vi "COD主界面（列队使用）.vi"() -> (8 "多列列表框":i32(listbox))   [LabVIEW 2016, in "斯坦道CODMn.lvlib"]
uses:
  <vilib>/Utility/miscctls.llb/LVPointTypeDef.ctl
  <vilib>/Analysis/6fits.llb/Curve Fitting Criteria.ctl
  <vilib>/Utility/config.llb/Read Key (I32).vi
  <vilib>/Utility/config.llb/Read Key (Double).vi
  <vilib>/Utility/config.llb/Read Key (Boolean).vi
  <vilib>/Utility/config.llb/Write Key (Double).vi
  <vilib>/Utility/config.llb/Write Key (Boolean).vi
  <vilib>/Utility/config.llb/Write Key (I32).vi
  <vilib>/Waveform/WDTFileIO.llb/Read Waveform from File.vi
  <vilib>/ptbypt/NI_PtbyPt.lvlib
  <vilib>/Utility/config.llb/NI_LVConfig.lvlib
  <vilib>/Analysis/NI_AALPro.lvlib
panel:
  out "CODMn工作状态":T1(ring)
  out "ORP-K":string
  out "ORP-B":string
  out "ORP-A":string
  out "x = y?":bool
  out "稀释倍数解释":string
  in  "CODMn跨度量程选择":enum32{"H", "L", "AUTO"}(ring)=enum."AUTO"
  in  "跨度液浓度":dbl
  in  "水样":dbl
  in  "蒸馏水":dbl
  in  "标液":dbl
  in  "质控样":dbl
  in  "加标回收":dbl
  in  "草酸钠":dbl
  in  "高锰酸钾":dbl
  in  "硫酸":dbl
  out "量程解释说明":string
  in  "高切低阈值:":dbl
  in  "低切高阈值:":dbl
  in  "自动切换量程:":enum16{"关闭", "自动切换测一次", "自动切换测两次"}(ring)
  in  "修正系数":dbl
  in  "标准液浓度":dbl
  in  "温度":dbl
  in  "恒温时间":dbl
  in  "基本量程":enum16{"L", "H"}(ring)
  in  "CODMn零点核查选择":enum16{"零点核查走纯水管", "零点核查走质控管"}(ring)
  in  "锁定按钮":bool
  in  "低量程稀释倍数:":i8=1
  out "切换量程连续测两次":bool
  in  "高量程稀释倍数:":i8=2
  in  "一键写入":bool
  in  "测量模式(公式)":u16(ring)=1 items=["水样测试"=1, "标样核查"=2, "零点核查"=3, "跨度核查"=4, "空白测试"=5, "平行样"=6, "加标回收"=7]
  out "基本量程(显示)":string
  out "测量模式(显示)":string
  in  "量程切换次数":u8
  out "数据时间":string
  out "断电排液标记":bool
  in  "测量模式":T2(ring)
  out "COM":string
  in  "启用5":bool
  in  "校准5":bool
  in  "泵滴定数5":dbl
  in  "浓度5":dbl
  in  "启用4":bool
  in  "校准4":bool
  in  "泵滴定数4":dbl
  in  "浓度4":dbl
  out "波形时间":timestamp
  in  "历史波形":bool
  out "滴定数-ORP值":u16[](array[numeric]) caption="数组"
  in  "关闭 3":bool
  in  "滴定曲线":bool
  out "ORP滴定曲线":u16[](graph)
  out "空白测试标记":bool
  out "跨度核查标记":bool
  out "启动选择 2":u16(ring) items=["水样测试", "标样核查", "零点核查", "跨度核查", "空白测试", "加标回收", "平行样", "校零", "校标"]
  in  "量程选择":enum16{"低量程", "高量程", "0-2量程"}(ring)
  in  "手动控制":bool
  in  "选用水样":enum16{"葡萄糖", "草酸钠"}(ring)
  in  "方程系数":cluster{"X":dbl, "b":dbl, "X^2":dbl} {"X^2" format="%#.6g"; "b" format="%#.6g"; "X" format="%#.6g"}
  out "多项式系数1":dbl[](array[numeric]) caption="多项式系数"
  out "XY图":cluster{"X Values":dbl[], "Y Values":dbl[]}[](graph)
  in  "模型":enum32{"线性", "多项式"}(ring)
  out "启动时间":timestamp format="%<%Y/%m/%d %H:%M:%S>T"
  in  "24H周期设置":bool[](xcontrol)
  in  "关闭 2":bool
  in  "周期设置":bool
  out "r^2":dbl format="%.8g"
  out "拟合公式":string
  out "b":dbl format="%#.4g"
  out "K":dbl format="%#.4f"
  out "当前校准":i32
  in  "启用3":bool
  in  "启用2":bool
  in  "启用1":bool
  in  "校准3":bool
  in  "校准2":bool
  in  "校准1":bool
  in  "泵滴定数3":dbl
  in  "泵滴定数2":dbl
  in  "泵滴定数1":dbl
  in  "浓度3":dbl
  in  "浓度2":dbl
  in  "浓度1":dbl
  in  "写入":bool
  out "测量模式数字":i32
  out "零点核查标记":bool
  out "排液故障":bool
  out "进水样超量程":bool
  out "标样核查标记":bool
  out "平行样测量":bool
  out "加标回收测量":bool
  out "质控样测量":bool
  out "待机":bool
  out "校标错误":bool
  out "校零错误":bool
  out "测量错误":bool
  out "草酸钠报警":bool
  out "高锰酸钾报警":bool
  out "加热故障":bool
  out "温控器故障":bool
  out "ORP故障":bool
  out "排液标记":bool
  out "故障标记":bool
  out "校标标记":bool
  out "校零标记":bool
  out "通讯状态":bool
  out "水样测量":bool
  in  "读取":bool
  in  "返回":bool
  in  "校准配置":bool
  in  "零点泵计量数 2":dbl
  in  "标度泵计量数 2":dbl
  out "标度滴定值":dbl
  out "零点滴定值":dbl
  in  "保存":bool
  in  "关闭":bool
  out "测量数据区":T3 {"单位" items=["ug/L", "mg/L", "ppm", "mg/m3", "cm", "ppb", "ug/m3", "%", "nmol/mol", "umol/mol", "MPN/L", "MPN/100ml", "ng/m3", "NTU", "无量纲", "ms/cm", "us/cm", "℃", "mV", "万个/L"]}
  out "仪器时间":timestamp format="%<%Y/%m/%d %H:%M:%S>T"
  out "秒":u16
  out "分":u16
  out "COD浓度（mg/L)":dbl format="%.2g"
  out "进样管":dbl
  out "高锰酸钾":dbl
  out "草酸钠":dbl
  out "硫酸":dbl
  out "ORP显示":dbl
  out "温度":dbl
  out "加热":bool
  out "搅拌":bool
  out "进硫酸":bool
  out "进加标回收样":bool
  out "进质控样":bool
  out "进标液":bool
  out "进蒸馏水":bool
  out "进水样":bool
  out "进草酸钠":bool
  out "进高锰酸钾":bool
  out "定时启动":bool
  in  "启动":bool
  in  "故障清除":bool
  in  "参数配置":bool
  in  "停止":bool
  in  "单步启动":bool
  out "系统时间":timestamp
  in  "时间校准":bool
  out "报警簇":T4
  out "模式（受控）":u16
  # "测量时间："
  # "(水样~加标回收)"
  # "mV"
  # "℃"
  # "注：遇到加热故障和排液故障时仪器不能正常启动，\n必须排查故障并点击报警清除按钮方可运行。"
  # "mg/L"
  # "泵计量参数设置"
  # "基本参数设置"
  # "校零校标结果"
  # "校零结果："
  # "校零滴定值："
  # "加热恒温温度(℃):"
  # "水样："
  # "高锰酸钾："
  # "校标结果："
  # "标度滴定值："
  # "恒温时间(分钟):"
  # "草酸钠："
  # "蒸馏水："
  # "零点泵计量值："
  # "标准液浓度(mg/L):"
  # "硫酸："
  # "标液："
  # "标度泵计量值："
  # "修正系数："
  # "跨度液浓度："
  # "质控样:"
  # "基本量程(L、H)可选:"
  # "跨度量程选择："
  # "加标回收样："
  # "是否启用"
  # "泵滴定数"
  # "浓度"
  # "辅\n助\n计\n算\n区"
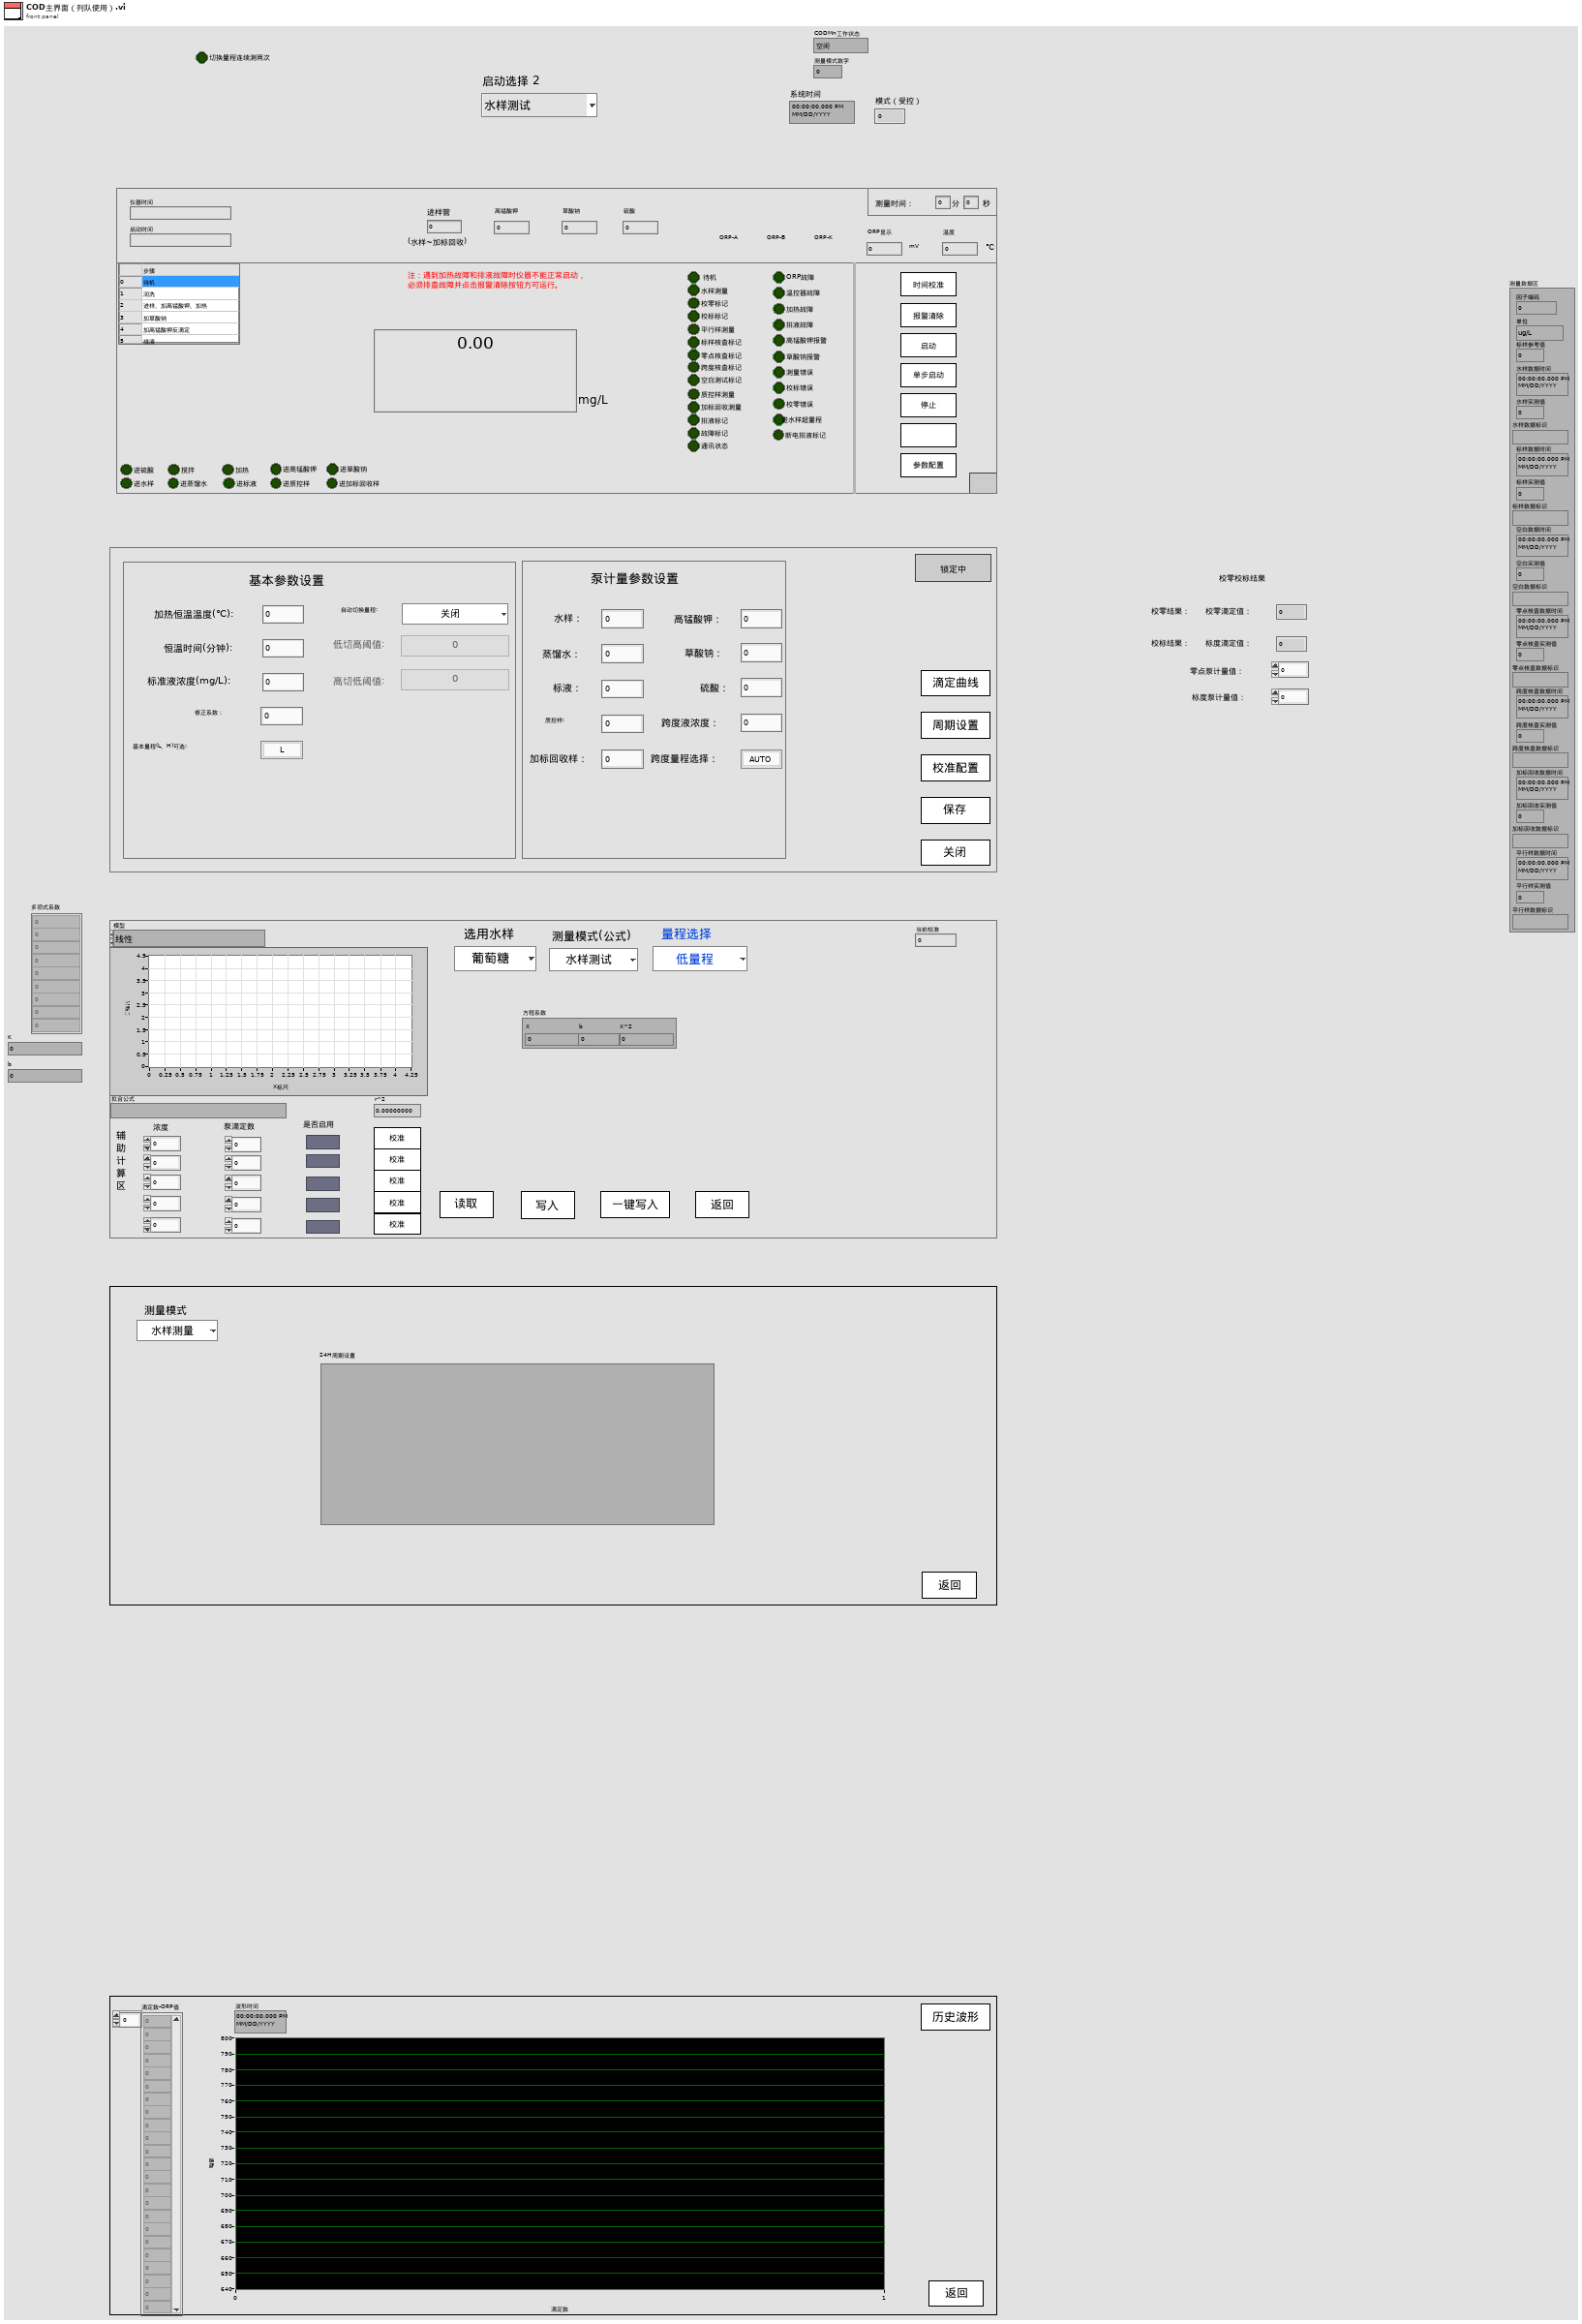
[diagram p1: front panel]
types:
  T1 = enum16{"空闲", "水样测试", "标样核查", "零点核查", "跨度核查", "空白测试", "平行样测试", "质控样", "空白校准", "标样校准", "加标回收"}
  T2 = enum16{"水样测量", "标样核查", "零点核查", "跨度核查", "空白测试", "加标回收", "平行样", "校零", "校标"}
  T3 = cluster{"因子编码":u32, "单位":u16, "标样参考值":sgl, "水样数据时间":timestamp, "水样实测值":sgl, "水样数据标识":string, "标样数据时间":timestamp, "标样实测值":sgl, "标样数据标识":string, "空白数据时间":timestamp, "空白实测值":sgl, "空白数据标识":string, "零点核查数据时间":timestamp, "零点核查实测值":sgl, "零点核查数据标识":string, "跨度核查数据时间":timestamp, "跨度核查实测值":sgl, "跨度核查数据标识":string, "加标回收数据时间":timestamp, "加标回收实测值":sgl, "加标回收数据标识":string, "平行样数据时间":timestamp, "平行样实测值":sgl, "平行样数据标识":string}
  T4 = cluster{"ORP故障":bool, "温控器故障":bool, "加热故障":bool, "高锰酸钾报警":bool, "草酸钠报警":bool, "测量错误":bool, "校零错误":bool, "校标错误":bool, " 进水样超量程":bool, "排液阀故障":bool}
  T5 = typedef "NI_LVConfig.lvlib/Config Data RefNum.ctl" = refnum<k1>
  T6 = enum8{"Enabled", "Disabled", "Disabled and Grayed Out"}
  T7 = cluster{"时间":timestamp, "测量模式":string, "数据类型":string, "检测值":sgl, "单位":string, "数据标识":string, "因子编码":string, "标样参考值":sgl, "ORP-A":sgl, "ORP-B":sgl, "ORP-K":sgl, "COD滴定值":sgl, "高锰酸钾滴定数":sgl, "温度":sgl, "量程":sgl}
  T8 = typedef "NI_AALPro.lvlib/Curve Fitting Criteria.ctl" = u16
  T9 = cluster{"数组 2[0]":sgl, "数组 2[1]":sgl, "数组 2[2]":sgl, "数组 2[3]":sgl, "数组 2[4]":sgl, "数组 2[5]":sgl, "数组 2[6]":sgl, "数组 2[7]":sgl, "数组 2[8]":sgl, "数组 2[9]":sgl, "数组 2[10]":sgl, "数组 2[11]":sgl, "数组 2[12]":sgl, "数组 2[13]":sgl, "数组 2[14]":sgl, "数组 2[15]":sgl, "数组 2[16]":sgl, "数组 2[17]":sgl, "数组 2[18]":sgl, "数组 2[19]":sgl, "数组 2[20]":sgl, "数组 2[21]":sgl, "数组 2[22]":sgl, "数组 2[23]":sgl, "数组 2[24]":sgl, "数组 2[25]":sgl, "数组 2[26]":sgl, "数组 2[27]":sgl, "数组 2[28]":sgl, "数组 2[29]":sgl, "数组 2[30]":sgl, "数组 2[31]":sgl, "数组 2[32]":sgl, "数组 2[33]":sgl, "数组 2[34]":sgl, "数组 2[35]":sgl, "数组 2[36]":sgl, "数组 2[37]":sgl, "数组 2[38]":sgl, "数组 2[39]":sgl, "数组 2[40]":sgl, "数组 2[41]":sgl}
  T10 = cluster{"测量模式":enum16{"水样测量", "标样核查", "零点核查", "跨度核查", "空白测试", "加标回收", "平行样", "校零", "校标"}}
  T11 = cluster{"仪器测试类型":enum16{"水样测试", "标样核查", "空白测试", "跨度核查"}, "周期设置类型":enum16{"定点启动", "间隔启动"}, "定时功能启用":bool, "定时间隔":dbl, "24H周期设置":bool[]}
  T12 = typedef "LVDateTimeRec.ctl" = cluster{"秒数的小数部分":dbl, "秒":i32, "分":i32, "时":i32, "日":i32, "月":i32, "年":i32, "天数（周）":i32, "天数（年）":i32, "DST":i32}
  T13 = typedef "LVPointTypeDef.ctl" = cluster{"Horizontal":i16, "Vertical":i16}
  T14 = cluster{"运行模式":enum16{"维护模式", "常规模式", "应急模式", "质控模式"}}
  T15 = cluster{"时间标识":timestamp, "参数":string, "日志信息":string, "流程参数":string}
  T16 = cluster{"时间标识":timestamp, "设备":string, "日志信息":string}
  T17 = cluster{"时间标识":timestamp, "设备":string, "日志信息":string, "流程参数":string}
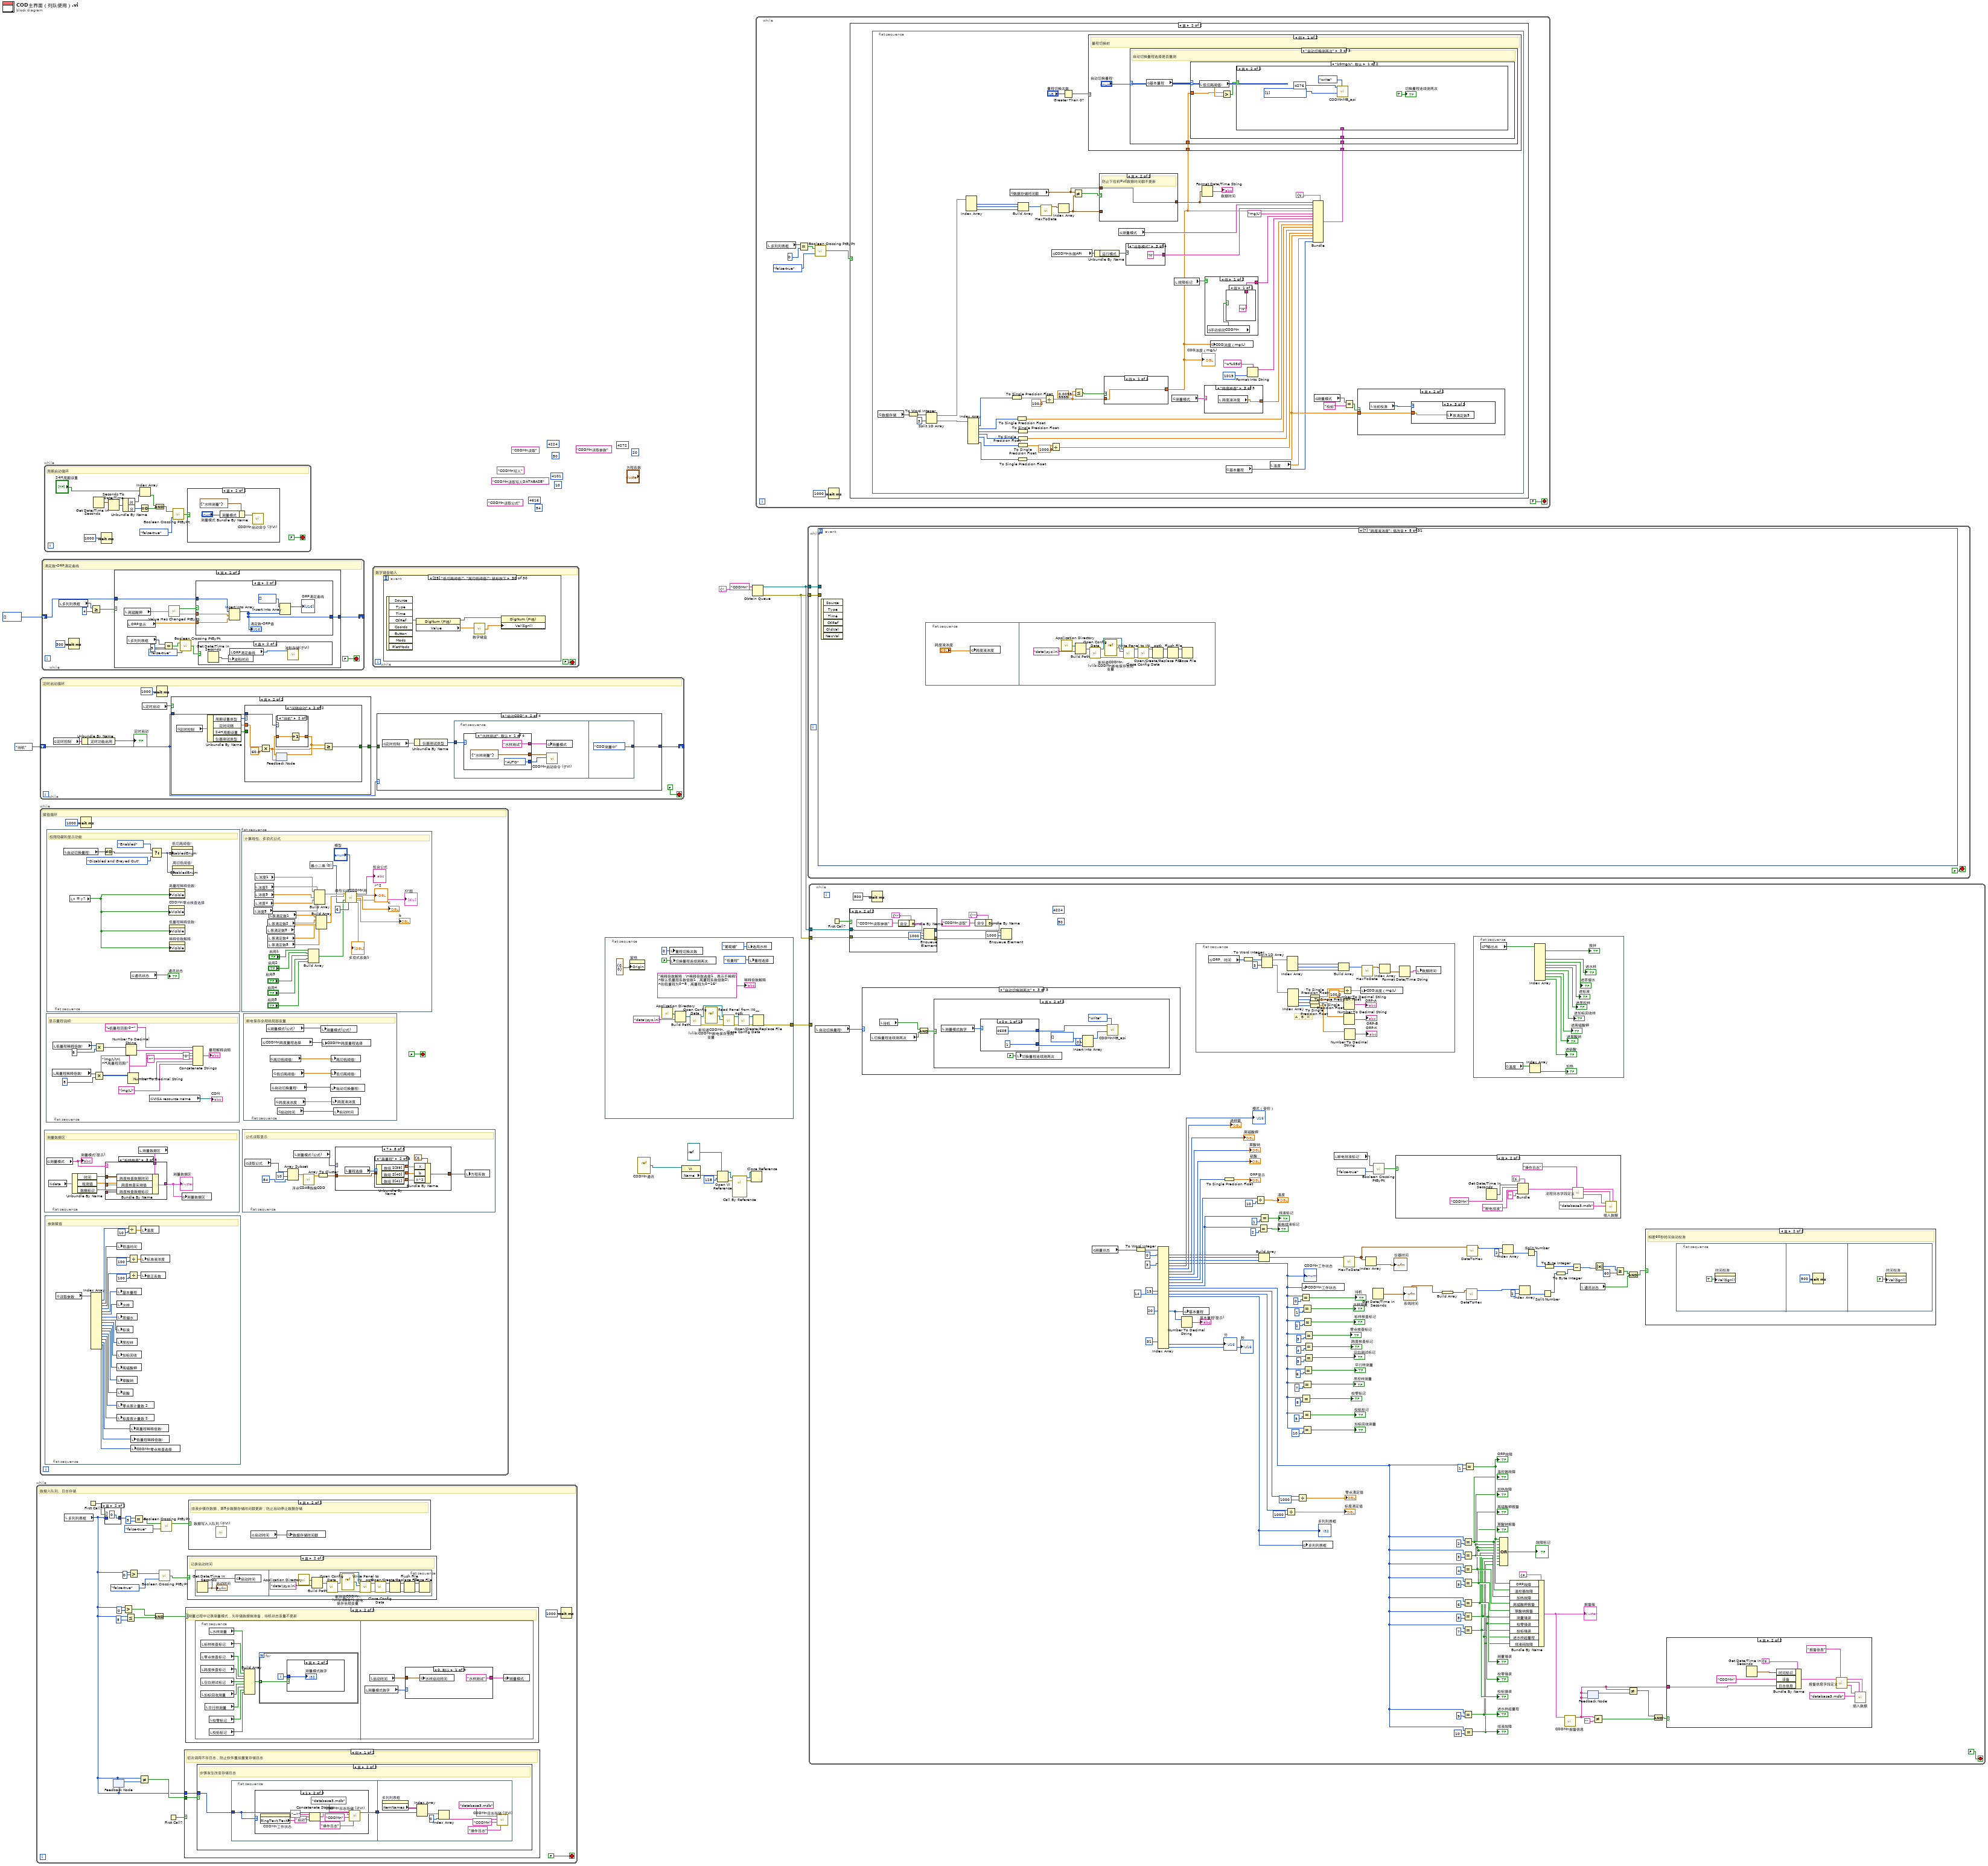
[diagram p0: block diagram]
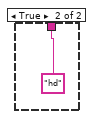
[diagram p4: hidden frame]
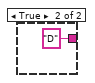
[diagram p5: hidden frame]
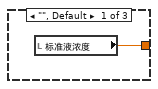
[diagram p6: hidden frame]
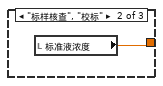
[diagram p7: hidden frame]
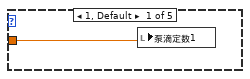
[diagram p9: hidden frame]
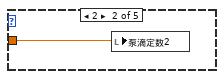
[diagram p10: hidden frame]
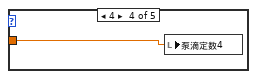
[diagram p11: hidden frame]
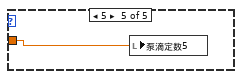
[diagram p12: hidden frame]
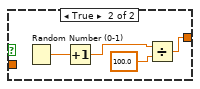
[diagram p13: hidden frame]
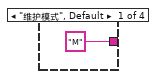
[diagram p14: hidden frame]
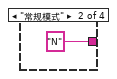
[diagram p15: hidden frame]
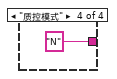
[diagram p16: hidden frame]
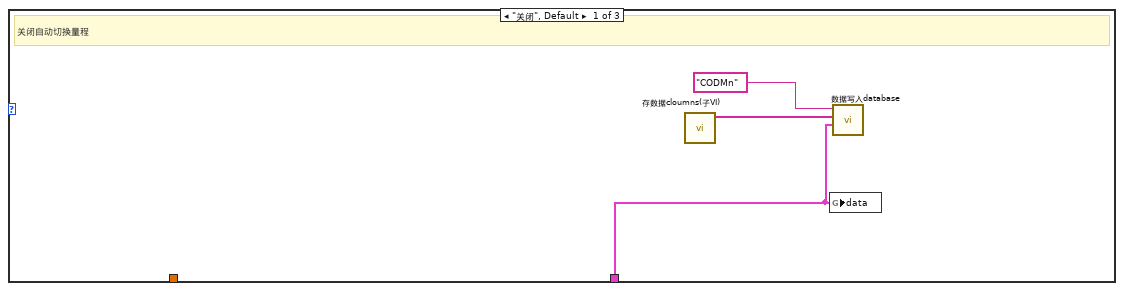
[diagram p17: hidden frame]
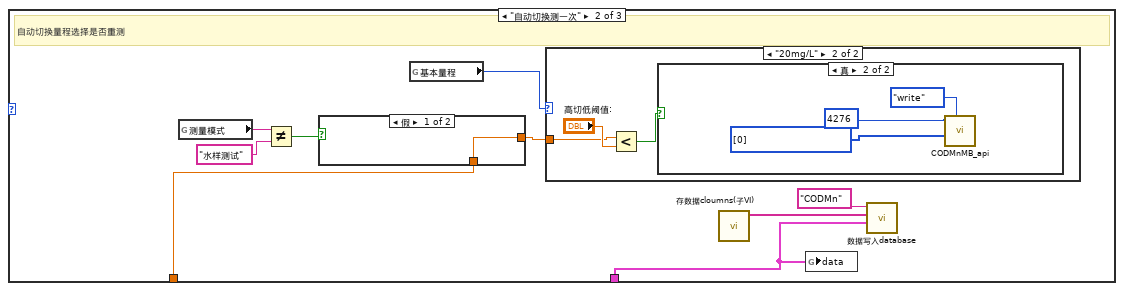
[diagram p18: hidden frame]
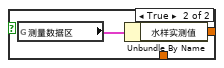
[diagram p19: hidden frame]
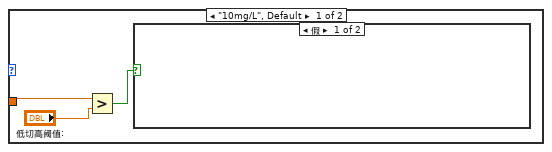
[diagram p20: hidden frame]
diagram:
  (unwired) u16 10 ("number of holding registers")
  (unwired) u16 4101 ("starting address")
  (unwired) u16 94 ("number of holding registers")
  (unwired) u16 4616 ("starting address")
  (unwired) u16 20 ("number of holding registers")
  (unwired) u16 4272 ("starting address")
  (unwired) u16 50 ("number of holding registers")
  (unwired) u16 4224 ("starting address")
  (unwired) "CODMn读取公式" ("名称（未命名）")
  (unwired) "CODMn读取写入DATABASE" ("名称（未命名）")
  (unwired) "CODMn读取参数" ("名称（未命名）")
  (unwired) "CODMn读取" ("名称（未命名）")
  (unwired) "CODMn写入" ("名称（未命名）")
  n1 = while {
    stop <- FALSE stop-if-true
    # "数据入队列、日志存储"
    n2 = local read "多列列表框"() -> (w16:i32)
    n3 = First Call?() -> (First Call?: T/F=w18:bool)
    n4 = case shown="真" w18 {
      tunnel: [w37 u16 0 ("y")] -> w17
      tunnel: w16 -> [w37 _]
      frame False {
      }
      frame True {
      }
    }
    n5 = feedback #1(w16) -> (w22:i32)
    n6 = feedback-in #1(w16) -> ()
    n7 = Greater?(x=w16, y=u16 0) -> (0:w36:bool)
    n8 = Less Or Equal?(x=w16, y=u16 5) -> (x <= y?=w30:bool)
    n9 = Greater?(x=w16, y=u16 0) -> (0:w33:bool)
    n10 = Equal?(x=w17, y=u16 5) -> (x = y?=w26:bool)
    n11 = Not Equal?(x=w16, y=w22) -> (x != y?=w23:bool)
    n12 = And(x=w36, y=w30) -> (x .and. y?=w34:bool)
    n13 = call <vilib>:"Boolean Crossing PtByPt.vi"("direction"=enum16{"either", "false-true", "true-false"}."false-true", "input"=w33) -> ("crossing"=w19:bool)  [unwired: 1 in]
    n14 = call <vilib>:"Boolean Crossing PtByPt.vi"("direction"=enum16{"either", "false-true", "true-false"}."false-true", "input"=w26) -> ("crossing"=w28:bool)  [unwired: 1 in]
    n15 = First Call?() -> (First Call?: T/F=w24:bool)
    n16 = case shown="假" w24 {
      tunnel: w23 -> [w40 _]
      tunnel: w16 -> [w39 _]
      frame False {
        # "初次调用不存日志，防止软件重启重复存储日志"
        n17 = case shown="真" w40 {
          tunnel: w39 -> [_ w42]
          frame False {
          }
          frame True {
            # "步骤发生改变存储日志"
            n18 = flat-sequence {
              tunnel: w42 -> [w43]
              tunnel: [w43] -> w41
              tunnel: w41 -> [w63]
              frame #0 {
                n19 = case shown="1" w43 {
                  frame 0 {
                    n20 = global read "COD测量模式全局.vi" "测量模式"() -> (w50:string)
                    n21 = Concatenate Strings("-->", w50, "结束" ("字符串")) -> (w49:string)
                    n22 = call "CODMn日志存储 (子VI).vi"("table输入"="操作日志", "参数"="CODMn" ("table输入"), "日志信息"=w49, "database"="database3.mdb") -> ()  [unwired: 8 in]
                  }
                  frame 1 {
                    n23 = property on="CODMn工作状态" class="Enum (严格)"() -> ("RingText.Text"=w53:string)  [unwired: 2 in, 2 out]
                    n24 = Concatenate Strings("-->", w53, "启动" ("字符串")) -> (w51:string)
                    n25 = call "CODMn日志存储 (子VI).vi"("table输入"="操作日志", "参数"="CODMn" ("table输入"), "日志信息"=w51, "database"="database3.mdb") -> ()  [unwired: 8 in]
                  }
                  frame 2, Default {
                  }
                }
              }
              frame #1 {
                n26 = property on="多列列表框" class="MCListbox (严格)"() -> ("ItemNames"=w61:string[][])  [unwired: 2 in, 2 out]
                n27 = Index Array(array=w61, index (row)=w63) -> (element=w60:string[])  [unwired: 1 in]
                n28 = Index Array(array=w60, index=0 ("索引")) -> (element=w58:string)
                n29 = call "CODMn日志存储 (子VI).vi"("table输入"="操作日志", "参数"="CODMn" ("table输入"), "日志信息"=w58, "database"="database3.mdb") -> ()  [unwired: 8 in]
              }
            }
          }
        }
      }
      frame True {
      }
    }
    n30 = case shown="真" w34 {
      frame False {
      }
      frame True {
        # "测量过程中记录测量模式，为存储数据做准备，待机状态变量不更新"
        n31 = flat-sequence {
          frame #0 {
            n32 = local read "标样核查标记"() -> (w89:bool)
            n33 = local read "零点核查标记"() -> (w88:bool)
            n34 = local read "跨度核查标记"() -> (w86:bool)
            n35 = local read "空白测试标记"() -> (w85:bool)
            n36 = local read "加标回收测量"() -> (w84:bool)
            n37 = local read "平行样测量"() -> (w83:bool)
            n38 = local read "水样测量"() -> (w90:bool)
            n39 = local read "校零标记"() -> (w82:bool)
            n40 = local read "校标标记"() -> (w81:bool)
            n41 = Build Array(w90, w89, w88, w86, w85, w84, w83, w82, w81) -> (w87:bool[])
            n42 = for {
              tunnel: w87 -> [w92] mode=indexing
              i -> [w91]
              n43 = case shown="真" w92 {
                tunnel: w91 -> [_ w93]
                frame False {
                }
                frame True {
                  "测量模式数字" <- w93
                }
              }
            }
          }
          frame #1 {
            n44 = local read "测量模式数字"() -> (w96:i32)
            n45 = local read "启动时间"() -> (w94:timestamp)
            n46 = case shown="0, 默认" w96 {
              tunnel: ["水样测试" ("测量模式") "标样核查" ("测量模式") "零点核查" ("测量模式") "跨度核查" ("测量模式") "空白测试" ("测量模式") "加标回收" ("测量模式") "平行样" ("测量模式") "校零" ("测量模式") "校标" ("测量模式")] -> w95
              tunnel: w94 -> [w97 _ _ _ _ w103 _ _ _]
              frame 0, Default {
                n47 = global write "COD测量模式全局.vi" "水样启动时间"(w97) -> ()
              }
              frame 1 {
              }
              frame 2 {
              }
              frame 3 {
              }
              frame 4 {
              }
              frame 5 {
                n48 = global write "COD测量模式全局.vi" "加标回收启动时间"(w103) -> ()
              }
              frame 6 {
              }
              frame 7 {
              }
              frame 8 {
              }
            }
            n49 = global write "COD测量模式全局.vi" "测量模式"(w95) -> ()
          }
        }
      }
    }
    n50 = case shown="真" w19 {
      frame False {
      }
      frame True {
        # "记录启动时间"
        n51 = flat-sequence {
          frame #0 {
            n52 = Get Date/Time In Seconds() -> (seconds since 1Jan1904=w66:timestamp)
            "启动时间" <- w66
            n53 = global write "CODMn断电保存全局变量.vi" "启动时间"(w66) -> ()
          }
          frame #1 {
            n54 = call <vilib>:"Application Directory.vi"() -> ("Application Directory"=w80:path)
            n55 = Build Path(base path=w80, name or relative path="data\\sys.ini" ("名称或相对路径")) -> (appended path=w78:path)
            n56 = call <vilib>:"Open Config Data.vi"("configuration file path"=w78) -> ("error out"=w74:errorcluster, "refnum"=w77:T5)  [unwired: 8 in, 1 out]
            n57 = vi-ref "斯坦道CODMn.lvlib:CODMn断电保存全局变量.vi"() -> (w76:refnum<vi>)
            n58 = call <userlib>:"Write Panel to INI__ogtk.vi"("error in (no error)"=w74, "VI ref"=w76, "refnum"=w77) -> ("error out"=w73:errorcluster, "refnum out"=w75:T5)  [unwired: 7 in]
            n59 = call <vilib>:"Close Config Data.vi"("error in (no error)"=w73, "refnum"=w75) -> ("error out"=w68:errorcluster, "file path"=w67:path)  [unwired: 8 in]
            n60 = Open/Create/Replace File(file path (use dialog)=w67, error in=w68) -> (refnum out=w71:refnum<file>, error out=w72:errorcluster)  [unwired: 4 in, 1 out]
            n61 = Flush File(refnum=w71, error in=w72) -> (refnum out=w70:refnum<file>, error out=w69:errorcluster)
            n62 = Close File(refnum=w70, error in=w69) -> ()  [unwired: 2 out]
          }
        }
      }
    }
    n63 = case shown="真" w28 {
      frame False {
      }
      frame True {
        # "排液步骤存数据，第5步数据存储时间戳更新，防止启动停止数据存储"
        n64 = call "数据写入入队列 (子VI).vi"() -> ()  [unwired: 12 in]
        n65 = global read "CODMn断电保存全局变量.vi" "启动时间"() -> (w108:timestamp)
        n66 = global write "COD读取DATA全局.vi" "数据存储时间戳"(w108) -> ()
      }
    }
    n67 = Wait (ms)(milliseconds to wait=u32 1000 ("等待时间（毫秒）")) -> ()  [unwired: 1 out]
  }
  n68 = while {
    stop <- FALSE stop-if-true
    # "赋值循环"
    n69 = flat-sequence {
      frame #0 {
        # "测量数据区"
        n70 = global read "COD测量模式全局.vi" "测量模式"() -> (w305:string)
        "测量模式(显示)" <- w305
        n71 = global read "COD读取DATA全局.vi" "data"() -> (w310:T7)
        n72 = Unbundle By Name(w310) -> ("时间"=w309:timestamp, "检测值"=w308:sgl, "数据标识"=w307:string)
        n73 = local read "测量数据区"() -> (w311:T3)
        n74 = case shown="\"标样核查\"" w305 {
          tunnel: w311 -> [w312 w317 w322 w327 w332 w337 w342 w347]
          tunnel: [w312 w316 w318 w326 w331 w336 w338 w346] -> w306
          tunnel: w309 -> [_ w315 w321 w325 w330 w335 w341 w345]
          tunnel: w308 -> [_ w314 w320 w324 w329 w334 w340 w344]
          tunnel: w307 -> [_ w313 w319 w323 w328 w333 w339 w343]
          frame "", Default {
          }
          frame "水样测试" {
            n75 = Bundle By Name(cluster=w317, "水样数据时间"=w315, "水样实测值"=w314, "水样数据标识"=w313) -> (w316:T3)
          }
          frame "标样核查" {
            n76 = Bundle By Name(cluster=w322, "跨度核查数据时间"=w321, "跨度核查实测值"=w320, "跨度核查数据标识"=w319) -> (w318:T3)
          }
          frame "零点核查" {
            n77 = Bundle By Name(cluster=w327, "零点核查数据时间"=w325, "零点核查实测值"=w324, "零点核查数据标识"=w323) -> (w326:T3)
          }
          frame "加标回收" {
            n78 = Bundle By Name(cluster=w332, "加标回收数据时间"=w330, "加标回收实测值"=w329, "加标回收数据标识"=w328) -> (w331:T3)
          }
          frame "平行样" {
            n79 = Bundle By Name(cluster=w337, "平行样数据时间"=w335, "平行样实测值"=w334, "平行样数据标识"=w333) -> (w336:T3)
          }
          frame "校零" {
            n80 = Bundle By Name(cluster=w342, "空白数据时间"=w341, "空白实测值"=w340, "空白数据标识"=w339) -> (w338:T3)
          }
          frame "校标" {
            n81 = Bundle By Name(cluster=w347, "标样数据时间"=w345, "标样实测值"=w344, "标样数据标识"=w343) -> (w346:T3)
          }
        }
        "测量数据区" <- w306
        n82 = global write "COD读取DATA全局.vi" "测量数据区"(w306) -> ()
      }
    }
    n83 = flat-sequence {
      frame #0 {
        # "参数赋值"
        n84 = global read "COD读取DATA全局.vi" "读取参数"() -> (w111:u16[])
        n85 = Index Array(array=w111) -> (element #1=w123:u16, element #2=w135:u16, element #3=w116:u16, element #4=w121:u16, element #5=w119:u16, element #6=w118:u16, element #7=w134:u16, element #8=w133:u16, element #9=w132:u16, element #10=w131:u16, element #11=w130:u16, element #12=w129:u16, element #13=w128:u16, element #14=w127:u16, element #15=w126:u16, element #16=w114:u16, element #17=w113:u16, element #18=w112:u16)  [unwired: 18 in]
        n86 = local write "恒温时间"(w135) -> ()
        n87 = local write "基本量程"(w119) -> ()
        n88 = local write "水样"(w118) -> ()
        n89 = local write "蒸馏水"(w134) -> ()
        n90 = local write "标液"(w133) -> ()
        n91 = local write "质控样"(w132) -> ()
        n92 = local write "加标回收"(w131) -> ()
        n93 = local write "高锰酸钾"(w130) -> ()
        n94 = local write "草酸钠"(w129) -> ()
        n95 = local write "硫酸"(w128) -> ()
        n96 = local write "零点泵计量数 2"(w127) -> ()
        n97 = local write "标度泵计量数 2"(w126) -> ()
        n98 = Divide(x=w123, y=u16 10) -> (x/y=w124:dbl)
        n99 = Divide(x=w116, y=u16 100) -> (x/y=w115:dbl)
        n100 = Divide(x=w121, y=u16 100) -> (x/y=w120:dbl)
        n101 = local write "高量程稀释倍数:"(w114) -> ()
        n102 = local write "低量程稀释倍数:"(w113) -> ()
        n103 = local write "CODMn零点核查选择"(w112) -> ()
        n104 = local write "温度"(w124) -> ()
        n105 = local write "标准液浓度"(w115) -> ()
        n106 = local write "修正系数"(w120) -> ()
      }
    }
    n107 = flat-sequence {
      frame #0 {
        # "显示量程说明"
        n108 = local read "高量程稀释倍数:"() -> (w357:i8)
        n109 = local read "低量程稀释倍数:"() -> (w367:i8)
        n110 = Multiply(x=w357, y=i8 8) -> (x*y=w355:i8)
        n111 = Multiply(x=w367, y=i8 8) -> (x*y=w359:i8)
        n112 = Number To Decimal String(number=w359) -> (decimal integer string=w364:string)  [unwired: 1 in]
        n113 = Number To Decimal String(number=w355) -> (decimal integer string=w362:string)  [unwired: 1 in]
        n114 = global read "CODMn断电保存全局变量.vi" "VISA resource name"() -> (→"COM":refnum<visa-resource-name>)
        n115 = Concatenate Strings("L低量程范围:0~" ("量程解释说明"), w364, "(mg/L)\n\nH高量程范围:" ("量程解释说明"), "0" ("字符串"), "~" ("量程解释说明"), w362, "(mg/L)" ("量程解释说明")) -> (→"量程解释说明":string)
      }
    }
    n116 = flat-sequence {
      frame #0 {
        # "权限隐藏和显示功能"
        n117 = local read "自动切换量程:"() -> (w373:enum16{"关闭", "自动切换测一次", "自动切换测两次"})
        n118 = local read "x = y?"() -> (w371:bool)
        n119 = Not Equal To 0?(x=w373) -> (x != 0?=w372:bool)
        n120 = global read "COD读取DATA全局.vi" "通讯状态"() -> (→"通讯状态":bool)
        n121 = Select(t=T6."Enabled" ("禁用"), s=w372, f=T6."Disabled and Grayed Out" ("禁用")) -> (s? t:f=w374:T6)
        n122 = property on="CODMn零点核查选择" class="Enum (严格)"("Visible"=w371) -> ()  [unwired: 2 in, 2 out]
        n123 = property on="高量程稀释倍数:" class="DigNum (严格)"("Visible"=w371) -> ()  [unwired: 2 in, 2 out]
        n124 = property on="低量程稀释倍数:" class="DigNum (严格)"("Visible"=w371) -> ()  [unwired: 2 in, 2 out]
        n125 = property on="稀释倍数解释" class="Str"("Visible"=w371) -> ()  [unwired: 2 in, 2 out]
        n126 = property on="低切高阈值:" class="DigNum (严格)"("DisabledEnum"=w374) -> ()  [unwired: 2 in, 2 out]
        n127 = property on="高切低阈值:" class="DigNum (严格)"("DisabledEnum"=w374) -> ()  [unwired: 2 in, 2 out]
      }
    }
    n128 = Wait (ms)(milliseconds to wait=u32 1000 ("等待时间（毫秒）")) -> ()  [unwired: 1 out]
    n129 = flat-sequence {
      frame #0 {
        w295 = T8 0 items=["最小二乘", "最小绝对残差", "Bisquare"] ("method")
        # "计算线性、多项式公式"
        n130 = local read "浓度5"() -> (w286:dbl)
        n131 = local read "浓度4"() -> (w287:dbl)
        n132 = local read "浓度2"() -> (w300:dbl)
        n133 = local read "浓度3"() -> (w301:dbl)
        n134 = local read "浓度1"() -> (w299:dbl)
        n135 = local read "泵滴定数3"() -> (w304:dbl)
        n136 = local read "泵滴定数2"() -> (w303:dbl)
        n137 = local read "泵滴定数4"() -> (w285:dbl)
        n138 = local read "泵滴定数5"() -> (w284:dbl)
        n139 = local read "泵滴定数1"() -> (w302:dbl)
        n140 = Build Array("启用1", "启用2", "启用3", "启用4", "启用5") -> (w278:bool[])
        n141 = Build Array(w299, w300, w301, w287, w286) -> (w297:dbl[])
        n142 = Build Array(w302, w303, w304, w285, w284) -> (w296:dbl[])
        n143 = call "线性公式CODMn用.vi"("标液浓度"=w297, "监测浓度"=w296, "启用"=w278, "method"=w295, "模型"="模型", "精度"=6) -> ("拟合方程"=→"拟合公式":string, "r^2"=→"r^2":dbl, "slope"=→"K":dbl, "intercept"=→"b":dbl, "XY图"=→"XY图":cluster{"X Values":dbl[], "Y Values":dbl[]}[], "Polynomial Coefficients"=→"多项式系数1":dbl[])  [unwired: 8 in]
      }
    }
    n144 = flat-sequence {
      frame #0 {
        # "公式读取显示"
        n145 = global read "COD读取DATA全局.vi" "读取公式"() -> (w143:u16[])
        n146 = Array Subset(array=w143, index=10 ("索引"), length=84 ("长度")) -> (w138:u16[])
        n147 = local read "测量模式(公式)"() -> (w141:u16)
        n148 = call "浮点CDAB转换COD.vi"("数组"=w138) -> ("数组 2"=w139:sgl[])  [unwired: 10 in]
        n149 = Array To Cluster(array=w139) -> (cluster=w142:T9)
        n150 = case shown="7" w141 {
          tunnel: [cluster{"X":dbl, "b":dbl, "X^2":dbl} {"X"=999.0, "b"=999.0, "X^2"=999.0} ("方程系数") w146 w165 w184 w203 w222 w241 w260] -> w140
          tunnel: w142 -> [_ w145 w164 w183 w202 w221 w240 w259]
          frame 0, Default {
          }
          frame 1 {
            n151 = local read "量程选择"() -> (w148:enum16{"低量程", "高量程", "0-2量程"})
            n152 = case shown="\"低量程\", 默认" w148 {
              tunnel: w145 -> [w155 w159 w163]
              tunnel: [w154 w158 w162] -> w151
              tunnel: [w153 w157 w161] -> w150
              tunnel: [w152 w156 w160] -> w149
              frame "低量程", Default {
                n153 = Unbundle By Name(w155) -> ("数组 2[0]"=w154:sgl, "数组 2[1]"=w153:sgl, "数组 2[2]"=w152:sgl)
              }
              frame "高量程" {
                n154 = Unbundle By Name(w159) -> ("数组 2[3]"=w158:sgl, "数组 2[4]"=w157:sgl, "数组 2[5]"=w156:sgl)
              }
              frame "0-2量程" {
                n155 = Unbundle By Name(w163) -> ("数组 2[6]"=w162:sgl, "数组 2[7]"=w161:sgl, "数组 2[8]"=w160:sgl)
              }
            }
            n156 = Bundle By Name(cluster=cluster{"X":dbl, "b":dbl, "X^2":dbl} {"X"=0.0, "b"=0.0, "X^2"=0.0} ("方程系数"), "X"=w151, "b"=w150, "X^2"=w149) -> (w146:cluster{"X":dbl, "b":dbl, "X^2":dbl})
          }
          frame 2 {
            n157 = local read "量程选择"() -> (w167:enum16{"低量程", "高量程", "0-2量程"})
            n158 = case shown="\"高量程\"" w167 {
              tunnel: w164 -> [w174 w178 w182]
              tunnel: [w173 w177 w181] -> w170
              tunnel: [w172 w176 w180] -> w169
              tunnel: [w171 w175 w179] -> w168
              frame "低量程", Default {
                n159 = Unbundle By Name(w174) -> ("数组 2[6]"=w173:sgl, "数组 2[7]"=w172:sgl, "数组 2[8]"=w171:sgl)
              }
              frame "高量程" {
                n160 = Unbundle By Name(w178) -> ("数组 2[9]"=w177:sgl, "数组 2[10]"=w176:sgl, "数组 2[11]"=w175:sgl)
              }
              frame "0-2量程" {
                n161 = Unbundle By Name(w182) -> ("数组 2[6]"=w181:sgl, "数组 2[7]"=w180:sgl, "数组 2[8]"=w179:sgl)
              }
            }
            n162 = Bundle By Name(cluster=cluster{"X":dbl, "b":dbl, "X^2":dbl} {"X"=0.0, "b"=0.0, "X^2"=0.0} ("方程系数"), "X"=w170, "b"=w169, "X^2"=w168) -> (w165:cluster{"X":dbl, "b":dbl, "X^2":dbl})
          }
          frame 3 {
            n163 = local read "量程选择"() -> (w186:enum16{"低量程", "高量程", "0-2量程"})
            n164 = case shown="\"高量程\"" w186 {
              tunnel: w183 -> [w193 w197 w201]
              tunnel: [w192 w196 w200] -> w189
              tunnel: [w191 w195 w199] -> w188
              tunnel: [w190 w194 w198] -> w187
              frame "低量程", Default {
                n165 = Unbundle By Name(w193) -> ("数组 2[12]"=w192:sgl, "数组 2[13]"=w191:sgl, "数组 2[14]"=w190:sgl)
              }
              frame "高量程" {
                n166 = Unbundle By Name(w197) -> ("数组 2[15]"=w196:sgl, "数组 2[16]"=w195:sgl, "数组 2[17]"=w194:sgl)
              }
              frame "0-2量程" {
                n167 = Unbundle By Name(w201) -> ("数组 2[6]"=w200:sgl, "数组 2[7]"=w199:sgl, "数组 2[8]"=w198:sgl)
              }
            }
            n168 = Bundle By Name(cluster=cluster{"X":dbl, "b":dbl, "X^2":dbl} {"X"=0.0, "b"=0.0, "X^2"=0.0} ("方程系数"), "X"=w189, "b"=w188, "X^2"=w187) -> (w184:cluster{"X":dbl, "b":dbl, "X^2":dbl})
          }
          frame 4 {
            n169 = local read "量程选择"() -> (w205:enum16{"低量程", "高量程", "0-2量程"})
            n170 = case shown="\"高量程\"" w205 {
              tunnel: w202 -> [w212 w216 w220]
              tunnel: [w211 w215 w219] -> w208
              tunnel: [w210 w214 w218] -> w207
              tunnel: [w209 w213 w217] -> w206
              frame "低量程", Default {
                n171 = Unbundle By Name(w212) -> ("数组 2[18]"=w211:sgl, "数组 2[19]"=w210:sgl, "数组 2[20]"=w209:sgl)
              }
              frame "高量程" {
                n172 = Unbundle By Name(w216) -> ("数组 2[21]"=w215:sgl, "数组 2[22]"=w214:sgl, "数组 2[23]"=w213:sgl)
              }
              frame "0-2量程" {
                n173 = Unbundle By Name(w220) -> ("数组 2[6]"=w219:sgl, "数组 2[7]"=w218:sgl, "数组 2[8]"=w217:sgl)
              }
            }
            n174 = Bundle By Name(cluster=cluster{"X":dbl, "b":dbl, "X^2":dbl} {"X"=0.0, "b"=0.0, "X^2"=0.0} ("方程系数"), "X"=w208, "b"=w207, "X^2"=w206) -> (w203:cluster{"X":dbl, "b":dbl, "X^2":dbl})
          }
          frame 5 {
            n175 = local read "量程选择"() -> (w224:enum16{"低量程", "高量程", "0-2量程"})
            n176 = case shown="\"高量程\"" w224 {
              tunnel: w221 -> [w231 w235 w239]
              tunnel: [w230 w234 w238] -> w227
              tunnel: [w229 w233 w237] -> w226
              tunnel: [w228 w232 w236] -> w225
              frame "低量程", Default {
                n177 = Unbundle By Name(w231) -> ("数组 2[24]"=w230:sgl, "数组 2[25]"=w229:sgl, "数组 2[26]"=w228:sgl)
              }
              frame "高量程" {
                n178 = Unbundle By Name(w235) -> ("数组 2[27]"=w234:sgl, "数组 2[28]"=w233:sgl, "数组 2[29]"=w232:sgl)
              }
              frame "0-2量程" {
                n179 = Unbundle By Name(w239) -> ("数组 2[6]"=w238:sgl, "数组 2[7]"=w237:sgl, "数组 2[8]"=w236:sgl)
              }
            }
            n180 = Bundle By Name(cluster=cluster{"X":dbl, "b":dbl, "X^2":dbl} {"X"=0.0, "b"=0.0, "X^2"=0.0} ("方程系数"), "X"=w227, "b"=w226, "X^2"=w225) -> (w222:cluster{"X":dbl, "b":dbl, "X^2":dbl})
          }
          frame 6 {
            n181 = local read "量程选择"() -> (w243:enum16{"低量程", "高量程", "0-2量程"})
            n182 = case shown="\"高量程\"" w243 {
              tunnel: w240 -> [w250 w254 w258]
              tunnel: [w249 w253 w257] -> w246
              tunnel: [w248 w252 w256] -> w245
              tunnel: [w247 w251 w255] -> w244
              frame "低量程", Default {
                n183 = Unbundle By Name(w250) -> ("数组 2[30]"=w249:sgl, "数组 2[31]"=w248:sgl, "数组 2[32]"=w247:sgl)
              }
              frame "高量程" {
                n184 = Unbundle By Name(w254) -> ("数组 2[33]"=w253:sgl, "数组 2[34]"=w252:sgl, "数组 2[35]"=w251:sgl)
              }
              frame "0-2量程" {
                n185 = Unbundle By Name(w258) -> ("数组 2[6]"=w257:sgl, "数组 2[7]"=w256:sgl, "数组 2[8]"=w255:sgl)
              }
            }
            n186 = Bundle By Name(cluster=cluster{"X":dbl, "b":dbl, "X^2":dbl} {"X"=0.0, "b"=0.0, "X^2"=0.0} ("方程系数"), "X"=w246, "b"=w245, "X^2"=w244) -> (w241:cluster{"X":dbl, "b":dbl, "X^2":dbl})
          }
          frame 7 {
            n187 = local read "量程选择"() -> (w262:enum16{"低量程", "高量程", "0-2量程"})
            n188 = case shown="\"高量程\"" w262 {
              tunnel: w259 -> [w269 w273 w277]
              tunnel: [w268 w272 w276] -> w265
              tunnel: [w267 w271 w275] -> w264
              tunnel: [w266 w270 w274] -> w263
              frame "低量程", Default {
                n189 = Unbundle By Name(w269) -> ("数组 2[36]"=w268:sgl, "数组 2[37]"=w267:sgl, "数组 2[38]"=w266:sgl)
              }
              frame "高量程" {
                n190 = Unbundle By Name(w273) -> ("数组 2[39]"=w272:sgl, "数组 2[40]"=w271:sgl, "数组 2[41]"=w270:sgl)
              }
              frame "0-2量程" {
                n191 = Unbundle By Name(w277) -> ("数组 2[6]"=w276:sgl, "数组 2[7]"=w275:sgl, "数组 2[8]"=w274:sgl)
              }
            }
            n192 = Bundle By Name(cluster=cluster{"X":dbl, "b":dbl, "X^2":dbl} {"X"=0.0, "b"=0.0, "X^2"=0.0} ("方程系数"), "X"=w265, "b"=w264, "X^2"=w263) -> (w260:cluster{"X":dbl, "b":dbl, "X^2":dbl})
          }
        }
        n193 = local write "方程系数"(w140) -> ()
      }
    }
    n194 = flat-sequence {
      frame #0 {
        # "断电保存全局给局部变量"
        n195 = global read "CODMn断电保存全局变量.vi" "CODMn跨度量程选择"() -> (w353:enum32{"H", "L", "AUTO"})
        n196 = global read "CODMn断电保存全局变量.vi" "测量模式(公式)"() -> (w354:u16)
        n197 = global read "CODMn断电保存全局变量.vi" "高切低阈值:"() -> (w352:dbl)
        n198 = global read "CODMn断电保存全局变量.vi" "自动切换量程:"() -> (w350:enum16{"关闭", "自动切换测一次", "自动切换测两次"})
        n199 = global read "CODMn断电保存全局变量.vi" "低切高阈值:"() -> (w351:dbl)
        n200 = global read "CODMn断电保存全局变量.vi" "跨度液浓度"() -> (w349:dbl)
        n201 = global read "CODMn断电保存全局变量.vi" "启动时间"() -> (w348:timestamp)
        n202 = local write "测量模式(公式)"(w354) -> ()
        n203 = local write "CODMn跨度量程选择"(w353) -> ()
        n204 = local write "自动切换量程:"(w350) -> ()
        n205 = local write "高切低阈值:"(w352) -> ()
        n206 = local write "低切高阈值:"(w351) -> ()
        n207 = local write "跨度液浓度"(w349) -> ()
        n208 = local write "启动时间"(w348) -> ()
      }
    }
  }
  n209 = while {
    shift-right: [w382] -> _
    shift-left: enum16{"待机", "启动COD", "COD测量中", "延时"}."待机" -> [w381]
    stop <- FALSE stop-if-true
    # "定时启动循环"
    n210 = global read "CODMn断电保存全局变量.vi" "定时控制"() -> (w378:T11)
    n211 = Unbundle By Name(w378) -> ("定时功能启用"=→"定时启动":bool)
    n212 = local read "定时启动"() -> (w379:bool)
    n213 = Wait (ms)(milliseconds to wait=u32 1000 ("等待时间（毫秒）")) -> ()  [unwired: 1 out]
    n214 = case shown="真" w379 {
      tunnel: w381 -> [_ w422]
      tunnel: [_ w421] -> w380
      frame False {
      }
      frame True {
        n215 = global read "CODMn断电保存全局变量.vi" "定时控制"() -> (w420:T11)
        n216 = Unbundle By Name(w420) -> ("周期设置类型"=w423:enum16{"定点启动", "间隔启动"}, "定时间隔"=w424:dbl, "24H周期设置"=w425:bool[])  [unwired: 1 out]
        n217 = case shown="\"间隔启动\"" w423 {
          tunnel: w424 -> [_ w442]
          tunnel: w425 -> [w428 _]
          tunnel: w422 -> [w426 w445]
          tunnel: [w427 w440] -> w421
          frame "定点启动", Default {
            n218 = case shown="\"待机\", 默认" w426 {
              tunnel: w428 -> [w436 _]
              tunnel: [w429 _] -> w427
              frame "待机", Default {
                n219 = Get Date/Time In Seconds() -> (seconds since 1Jan1904=w438:timestamp)
                n220 = Seconds To Date/Time(time stamp (now)=w438) -> (date time rec=w437:T12)  [unwired: 1 in]
                n221 = Unbundle By Name(w437) -> ("时"=w435:i32, "分"=w433:i32, "秒"=w434:i32)
                n222 = Equal To 0?(x=w433) -> (x = 0?=w431:bool)
                n223 = Equal To 0?(x=w434) -> (x = 0?=w430:bool)
                n224 = Index Array(array=w436, index=w435) -> (element=w432:bool)
                n225 = Compound Arithmetic op=AND ("复合运算")(w432, w431, w430) -> (w429:bool)
              }
              frame "启动COD" {
              }
            }
          }
          frame "间隔启动" {
            n226 = Multiply(x=w442, y=60.0) -> (x*y=w439:dbl)
            n227 = feedback #2(w439) -> (w444:dbl)
            n228 = case shown="\"待机\"" w445 {
              tunnel: w444 -> [_ w447]
              tunnel: [_ w446] -> w443
              frame Default {
              }
              frame "待机" {
                n229 = Increment(x=w447) -> (x+1=w446:dbl)
              }
            }
            n230 = feedback-in #2(w443) -> ()
            n231 = Greater Or Equal?(x=w443, y=w439) -> (x >= y?=w440:bool)
          }
        }
      }
    }
    n232 = case shown="\"启动COD\"" w381 {
      tunnel: [w385 w391 w410 enum16{"待机", "启动COD", "COD测量中", "延时"}."待机"] -> w382
      tunnel: w380 -> [w388 _ _ _]
      frame "待机", Default {
        n233 = Select(t=enum16{"待机", "启动COD", "COD测量中", "延时"}."启动COD", s=w388, f=enum16{"待机", "启动COD", "COD测量中", "延时"}."待机") -> (s? t:f=w385:enum16{"待机", "启动COD", "COD测量中", "延时"})
      }
      frame "启动COD" {
        n234 = global read "CODMn断电保存全局变量.vi" "定时控制"() -> (w389:T11)
        n235 = Unbundle By Name(w389) -> ("仪器测试类型"=w390:enum16{"水样测试", "标样核查", "空白测试", "跨度核查"})
        n236 = flat-sequence {
          tunnel: w390 -> [w395]
          tunnel: [enum16{"待机", "启动COD", "COD测量中", "延时"}."COD测量中"] -> w391
          frame #0 {
            n237 = case shown="\"水样测试\", 默认" w395 {
              tunnel: [T10 {"测量模式"=enum."水样测量"} ("启动测量模式") T10 {"测量模式"=enum."标样核查"} ("启动测量模式") T10 {"测量模式"=enum."空白测试"} ("启动测量模式") T10 {"测量模式"=enum."跨度核查"} ("启动测量模式")] -> w394
              tunnel: ["水样测试" ("测量模式") "标样核查" ("测量模式") "空白测试" ("测量模式") "跨度核查" ("测量模式")] -> w393
              tunnel: [enum32{"H", "L", "AUTO"}."AUTO" ("CODMn跨度量程选择") w399 enum32{"H", "L", "AUTO"}."L" ("CODMn跨度量程选择") w405] -> w392
              frame "水样测试", Default {
              }
              frame "标样核查" {
                n238 = local read "CODMn跨度量程选择"() -> (w399:enum32{"H", "L", "AUTO"})
              }
              frame "空白测试" {
              }
              frame "跨度核查" {
                n239 = local read "CODMn跨度量程选择"() -> (w405:enum32{"H", "L", "AUTO"})
              }
            }
            n240 = global write "COD测量模式全局.vi" "测量模式"(w393) -> ()
            n241 = call "CODMn启动命令 (子VI).vi"("CODMn量程切换"=w392, "启动测量模式"=w394) -> ()  [unwired: 10 in]
          }
          frame #1 {
          }
        }
      }
      frame "COD测量中" {
        n242 = flat-sequence {
          tunnel: [w411] -> w409
          tunnel: [w418] -> w410
          tunnel: w409 -> [w418]
          frame #0 {
            n243 = global read "运行时序全局变量.vi" "多列列表框"() -> (w416:i32)
            n244 = Equal?(x=w416, y=0) -> (x = y?=w414:bool)
            n245 = Select(t=enum16{"待机", "启动COD", "COD测量中", "延时"}."延时", s=w414, f=enum16{"待机", "启动COD", "COD测量中", "延时"}."COD测量中") -> (s? t:f=w411:enum16{"待机", "启动COD", "COD测量中", "延时"})
          }
          frame #1 {
            n246 = Wait (ms)(milliseconds to wait=u32 5000 ("等待时间（毫秒）")) -> ()  [unwired: 1 out]
          }
        }
      }
      frame "延时" {
      }
    }
  }
  n247 = while {
    shift-right: [w451] -> _
    shift-left: u16[] [] ("ORP滴定曲线") -> [w452]
    stop <- FALSE stop-if-true
    # "滴定数-ORP滴定曲线"
    n248 = local read "多列列表框"() -> (w450:i32)
    n249 = Wait (ms)(milliseconds to wait=u32 300 ("等待时间（毫秒）")) -> ()  [unwired: 1 out]
    n250 = Greater Or Equal?(x=w450, y=4) -> (x >= y?=w448:bool)
    n251 = case shown="真" w448 {
      tunnel: w452 -> [_ w466]
      tunnel: [u16[] [] ("ORP滴定曲线") w465] -> w451
      frame False {
      }
      frame True {
        n252 = local read "高锰酸钾"() -> (w462:dbl)
        n253 = local read "多列列表框"() -> (w460:i32)
        n254 = local read "ORP显示"() -> (w461:dbl)
        n255 = Equal?(x=w460, y=5) -> (x = y?=w458:bool)
        n256 = call <vilib>:"Value Has Changed PtByPt.vi"("input data point"=w462) -> ("has changed"=w464:bool, "output data point"=w463:dbl)  [unwired: 1 in]
        n257 = call <vilib>:"Boolean Crossing PtByPt.vi"("direction"=enum16{"either", "false-true", "true-false"}."false-true", "input"=w458) -> ("crossing"=w456:bool)  [unwired: 1 in]
        n258 = case shown="真" w464 {
          tunnel: w466 -> [w472 w482]
          tunnel: [w471 w481] -> w465
          tunnel: w463 -> [w473 w480]
          tunnel: w461 -> [w469 w479]
          frame False {
            n259 = Equal To 0?(x=w473) -> (x = 0?=w470:bool)
            n260 = case shown="真" w470 {
              tunnel: [w474 w477] -> w471
              tunnel: w472 -> [w474 _]
              tunnel: w469 -> [_ w476]
              frame False {
              }
              frame True {
                n261 = Insert Into Array(array=u16[] [] ("ORP滴定曲线"), index=0 ("索引"), new element=w476) -> (w477:u16[])
                n262 = local write "滴定数-ORP值"(w477) -> ()
              }
            }
          }
          frame True {
            n263 = Insert Into Array(array=w482, index=w480, new element=w479) -> (w481:u16[])
            "滴定数-ORP值" <- w481
            n264 = Insert Into Array(array=u16[] [] ("ORP滴定曲线"), new element=w481) -> (→"ORP滴定曲线":u16[])  [unwired: 1 in]
          }
        }
        n265 = case shown="真" w456 {
          frame False {
          }
          frame True {
            n266 = Get Date/Time In Seconds() -> (seconds since 1Jan1904=w467:timestamp)
            n267 = local write "波形时间"(w467) -> ()
            n268 = local read "ORP滴定曲线"() -> (w468:u16[])
            n269 = call "波形存储(子VI).vi"("ORP滴定曲线"=w468) -> ()  [unwired: 11 in]
          }
        }
      }
    }
  }
  n270 = while "While循环" {
    stop <- FALSE stop-if-true
    # "周期启动循环"
    n271 = Get Date/Time In Seconds() -> (seconds since 1Jan1904=w496:timestamp)
    n272 = Wait (ms)(milliseconds to wait=u32 1000 ("等待时间（毫秒）")) -> ()  [unwired: 1 out]
    n273 = Seconds To Date/Time(time stamp (now)=w496) -> (date time rec=w495:T12)  [unwired: 1 in]
    n274 = Unbundle By Name(w495) -> ("时"=w492:i32, "分"=w494:i32)
    n275 = Equal To 0?(x=w494) -> (x = 0?=w493:bool)
    n276 = Index Array(array="24H周期设置", index=w492) -> (element=w491:bool)
    n277 = And(x=w491, y=w493) -> (x .and. y?=w489:bool)
    n278 = call <vilib>:"Boolean Crossing PtByPt.vi"("direction"=enum16{"either", "false-true", "true-false"}."false-true", "input"=w489) -> ("crossing"=w488:bool)  [unwired: 1 in]
    n279 = case shown="真" w488 {
      frame False {
      }
      frame True {
        n280 = Bundle By Name(cluster=T10 {"测量模式"=enum."水样测量"} ("启动测量模式"), "测量模式"="测量模式") -> (w498:T10)
        n281 = call "CODMn启动命令 (子VI).vi"("启动测量模式"=w498) -> ()  [unwired: 11 in]
      }
    }
  }
  n282 = while {
    stop <- FALSE stop-if-true
    # "数字键盘输入"
    n283 = event shown="[29] \"低切高阈值:\", \"高切低阈值:\": 鼠标按下" {
      selector: _ -> [_ _ _ _ _ _ _ _ _ _ _ _ _ _ _ _ _ _ _ _ _ _ _ _ _ _ _ _ _ _]
      dyn-events: _ -> [_ _ _ _ _ _ _ _ _ _ _ _ _ _ _ _ _ _ _ _ _ _ _ _ _ _ _ _ _ _]
      timeout: _ -> [_ _ _ _ _ _ _ _ _ _ _ _ _ _ _ _ _ _ _ _ _ _ _ _ _ _ _ _ _ _]
      event Timeout {
        n284 = event-data() -> ()  [unwired: 1 in, 3 out]
      }
      event "温度": Mouse Down {
        n285 = event-data() -> ()  [unwired: 1 in, 8 out]
        n286 = local read "温度"() -> (w502:dbl)
        n287 = call "数字键盘.vi"("OldNumber"=w502) -> ("NewNumber"=w501:sgl)
        n288 = local write "温度"(w501) -> ()
      }
      event "恒温时间": Mouse Down {
        n289 = event-data() -> ()  [unwired: 1 in, 8 out]
        n290 = local read "恒温时间"() -> (w503:dbl)
        n291 = call "数字键盘.vi"("OldNumber"=w503) -> ("NewNumber"=w504:sgl)
        n292 = local write "恒温时间"(w504) -> ()
      }
      event "标准液浓度": Mouse Down {
        n293 = event-data() -> ()  [unwired: 1 in, 8 out]
        n294 = local read "标准液浓度"() -> (w506:dbl)
        n295 = call "数字键盘.vi"("OldNumber"=w506) -> ("NewNumber"=w505:sgl)
        n296 = local write "标准液浓度"(w505) -> ()
      }
      event "修正系数": Mouse Down {
        n297 = event-data() -> ()  [unwired: 1 in, 8 out]
        n298 = local read "修正系数"() -> (w507:dbl)
        n299 = call "数字键盘.vi"("OldNumber"=w507) -> ("NewNumber"=w508:sgl)
        n300 = local write "修正系数"(w508) -> ()
      }
      event "水样": Mouse Down {
        n301 = event-data() -> ()  [unwired: 1 in, 8 out]
        n302 = local read "水样"() -> (w509:dbl)
        n303 = call "数字键盘.vi"("OldNumber"=w509) -> ("NewNumber"=w510:sgl)
        n304 = local write "水样"(w510) -> ()
      }
      event "蒸馏水": Mouse Down {
        n305 = event-data() -> ()  [unwired: 1 in, 8 out]
        n306 = local read "蒸馏水"() -> (w511:dbl)
        n307 = call "数字键盘.vi"("OldNumber"=w511) -> ("NewNumber"=w512:sgl)
        n308 = local write "蒸馏水"(w512) -> ()
      }
      event "标液": Mouse Down {
        n309 = event-data() -> ()  [unwired: 1 in, 8 out]
        n310 = local read "标液"() -> (w513:dbl)
        n311 = call "数字键盘.vi"("OldNumber"=w513) -> ("NewNumber"=w514:sgl)
        n312 = local write "标液"(w514) -> ()
      }
      event "质控样": Mouse Down {
        n313 = event-data() -> ()  [unwired: 1 in, 8 out]
        n314 = local read "质控样"() -> (w515:dbl)
        n315 = call "数字键盘.vi"("OldNumber"=w515) -> ("NewNumber"=w516:sgl)
        n316 = local write "质控样"(w516) -> ()
      }
      event "加标回收": Mouse Down {
        n317 = event-data() -> ()  [unwired: 1 in, 8 out]
        n318 = local read "加标回收"() -> (w517:dbl)
        n319 = call "数字键盘.vi"("OldNumber"=w517) -> ("NewNumber"=w518:sgl)
        n320 = local write "加标回收"(w518) -> ()
      }
      event "草酸钠": Mouse Down {
        n321 = event-data() -> ()  [unwired: 1 in, 8 out]
        n322 = local read "草酸钠"() -> (w519:dbl)
        n323 = call "数字键盘.vi"("OldNumber"=w519) -> ("NewNumber"=w520:sgl)
        n324 = local write "草酸钠"(w520) -> ()
      }
      event "高锰酸钾": Mouse Down {
        n325 = event-data() -> ()  [unwired: 1 in, 8 out]
        n326 = local read "高锰酸钾"() -> (w521:dbl)
        n327 = call "数字键盘.vi"("OldNumber"=w521) -> ("NewNumber"=w522:sgl)
        n328 = local write "高锰酸钾"(w522) -> ()
      }
      event "硫酸": Mouse Down {
        n329 = event-data() -> ()  [unwired: 1 in, 8 out]
        n330 = local read "硫酸"() -> (w523:dbl)
        n331 = call "数字键盘.vi"("OldNumber"=w523) -> ("NewNumber"=w524:sgl)
        n332 = local write "硫酸"(w524) -> ()
      }
      event "零点泵计量数 2": Mouse Down {
        n333 = event-data() -> ()  [unwired: 1 in, 8 out]
        n334 = local read "零点泵计量数 2"() -> (w525:dbl)
        n335 = call "数字键盘.vi"("OldNumber"=w525) -> ("NewNumber"=w526:sgl)
        n336 = local write "零点泵计量数 2"(w526) -> ()
      }
      event "标度泵计量数 2": Mouse Down {
        n337 = event-data() -> ()  [unwired: 1 in, 8 out]
        n338 = local read "标度泵计量数 2"() -> (w527:dbl)
        n339 = call "数字键盘.vi"("OldNumber"=w527) -> ("NewNumber"=w528:sgl)
        n340 = local write "标度泵计量数 2"(w528) -> ()
      }
      event "高量程稀释倍数:": Mouse Down {
        n341 = event-data() -> ()  [unwired: 1 in, 8 out]
        n342 = local read "高量程稀释倍数:"() -> (w530:i8)
        n343 = call "数字键盘.vi"("OldNumber"=w530) -> ("NewNumber"=w529:sgl)
        n344 = local write "高量程稀释倍数:"(w529) -> ()
      }
      event "低量程稀释倍数:": Mouse Down {
        n345 = event-data() -> ()  [unwired: 1 in, 8 out]
        n346 = local read "低量程稀释倍数:"() -> (w532:i8)
        n347 = call "数字键盘.vi"("OldNumber"=w532) -> ("NewNumber"=w531:sgl)
        n348 = local write "低量程稀释倍数:"(w531) -> ()
      }
      event "浓度1": Mouse Down {
        n349 = event-data() -> ()  [unwired: 1 in, 8 out]
        n350 = local read "浓度1"() -> (w534:dbl)
        n351 = call "数字键盘.vi"("OldNumber"=w534) -> ("NewNumber"=w533:sgl)
        n352 = property on="浓度1" class="DigNum (严格)"("Val(Sgnl)"=w533) -> ()  [unwired: 2 in, 2 out]
      }
      event "浓度2": Mouse Down {
        n353 = event-data() -> ()  [unwired: 1 in, 8 out]
        n354 = local read "浓度2"() -> (w536:dbl)
        n355 = call "数字键盘.vi"("OldNumber"=w536) -> ("NewNumber"=w535:sgl)
        n356 = property on="浓度2" class="DigNum (严格)"("Val(Sgnl)"=w535) -> ()  [unwired: 2 in, 2 out]
      }
      event "浓度3": Mouse Down {
        n357 = event-data() -> ()  [unwired: 1 in, 8 out]
        n358 = local read "浓度3"() -> (w538:dbl)
        n359 = call "数字键盘.vi"("OldNumber"=w538) -> ("NewNumber"=w537:sgl)
        n360 = property on="浓度3" class="DigNum (严格)"("Val(Sgnl)"=w537) -> ()  [unwired: 2 in, 2 out]
      }
      event "浓度4": Mouse Down {
        n361 = event-data() -> ()  [unwired: 1 in, 8 out]
        n362 = local read "浓度4"() -> (w540:dbl)
        n363 = call "数字键盘.vi"("OldNumber"=w540) -> ("NewNumber"=w539:sgl)
        n364 = property on="浓度4" class="DigNum (严格)"("Val(Sgnl)"=w539) -> ()  [unwired: 2 in, 2 out]
      }
      event "浓度5": Mouse Down {
        n365 = event-data() -> ()  [unwired: 1 in, 8 out]
        n366 = local read "浓度5"() -> (w542:dbl)
        n367 = call "数字键盘.vi"("OldNumber"=w542) -> ("NewNumber"=w541:sgl)
        n368 = property on="浓度5" class="DigNum (严格)"("Val(Sgnl)"=w541) -> ()  [unwired: 2 in, 2 out]
      }
      event "跨度液浓度": Mouse Down {
        n369 = event-data() -> ()  [unwired: 1 in, 8 out]
        n370 = local read "跨度液浓度"() -> (w544:dbl)
        n371 = call "数字键盘.vi"("OldNumber"=w544) -> ("NewNumber"=w543:sgl)
        n372 = property on="跨度液浓度" class="DigNum (严格)"("Val(Sgnl)"=w543) -> ()  [unwired: 2 in, 2 out]
      }
      event "跨度液浓度": Value Change {
        n373 = event-data() -> ()  [unwired: 1 in, 6 out]
        n374 = call <vilib>:"Application Directory.vi"() -> ("Application Directory"=w548:path)
        n375 = Build Path(base path=w548, name or relative path="data\\Set.ini" ("名称或相对路径")) -> (appended path=w550:path)
        n376 = local read "跨度液浓度"() -> (w545:dbl)
        n377 = call <vilib>:"Open Config Data.vi"("configuration file path"=w550) -> ("error out"=w552:errorcluster, "refnum"=w551:T5)  [unwired: 8 in, 1 out]
        n378 = call-poly <vilib>:"Write Key.vi"("section"="CODMn参数" ("key"), "error in (no error)"=w552, "value"=w545, "key"="跨度液浓度", "refnum"=w551) -> ("error out"=w554:errorcluster, "refnum out"=w553:T5)  [unwired: 4 in, 1 out]
        n379 = call <vilib>:"Close Config Data.vi"("error in (no error)"=w554, "refnum"=w553) -> ()  [unwired: 8 in, 2 out]
      }
      event "泵滴定数1": Mouse Down {
        n380 = event-data() -> ()  [unwired: 1 in, 8 out]
        n381 = local read "泵滴定数1"() -> (w556:dbl)
        n382 = call "数字键盘.vi"("OldNumber"=w556) -> ("NewNumber"=w555:sgl)
        n383 = property on="泵滴定数1" class="DigNum (严格)"("Val(Sgnl)"=w555) -> ()  [unwired: 2 in, 2 out]
      }
      event "泵滴定数2": Mouse Down {
        n384 = event-data() -> ()  [unwired: 1 in, 8 out]
        n385 = local read "泵滴定数2"() -> (w558:dbl)
        n386 = call "数字键盘.vi"("OldNumber"=w558) -> ("NewNumber"=w557:sgl)
        n387 = property on="泵滴定数2" class="DigNum (严格)"("Val(Sgnl)"=w557) -> ()  [unwired: 2 in, 2 out]
      }
      event "泵滴定数3": Mouse Down {
        n388 = event-data() -> ()  [unwired: 1 in, 8 out]
        n389 = local read "泵滴定数3"() -> (w560:dbl)
        n390 = call "数字键盘.vi"("OldNumber"=w560) -> ("NewNumber"=w559:sgl)
        n391 = property on="泵滴定数3" class="DigNum (严格)"("Val(Sgnl)"=w559) -> ()  [unwired: 2 in, 2 out]
      }
      event "泵滴定数4": Mouse Down {
        n392 = event-data() -> ()  [unwired: 1 in, 8 out]
        n393 = local read "泵滴定数4"() -> (w562:dbl)
        n394 = call "数字键盘.vi"("OldNumber"=w562) -> ("NewNumber"=w561:sgl)
        n395 = property on="泵滴定数4" class="DigNum (严格)"("Val(Sgnl)"=w561) -> ()  [unwired: 2 in, 2 out]
      }
      event "泵滴定数5": Mouse Down {
        n396 = event-data() -> ()  [unwired: 1 in, 8 out]
        n397 = local read "泵滴定数5"() -> (w564:dbl)
        n398 = call "数字键盘.vi"("OldNumber"=w564) -> ("NewNumber"=w563:sgl)
        n399 = property on="泵滴定数5" class="DigNum (严格)"("Val(Sgnl)"=w563) -> ()  [unwired: 2 in, 2 out]
      }
      event "低切高阈值:", "高切低阈值:": Mouse Down {
        n400 = event-data() -> ("CtlRef"=w568:refnum<vi>)  [unwired: 1 in, 7 out]
        n401 = property class="DigNum (严格)"(reference=w568) -> (reference out=w567:refnum<vi>, "Value"=w566:dbl)  [unwired: 1 in, 1 out]
        n402 = call "数字键盘.vi"("OldNumber"=w566) -> ("NewNumber"=w565:sgl)
        n403 = property class="DigNum (严格)"(reference=w567, "Val(Sgnl)"=w565) -> ()  [unwired: 1 in, 2 out]
      }
    }
  }
  n404 = flat-sequence {
    tunnel: [w569] -> w1
    frame #0 {
      n405 = property on="窗格" class="Pane"("Origin"=T13 {"Horizontal"=0, "Vertical"=0} ("原点")) -> ()  [unwired: 2 in, 2 out]
      n406 = call <vilib>:"Application Directory.vi"() -> ("Application Directory"=w579:path)
      n407 = local write "量程切换次数"(u8 0 ("量程切换次数")) -> ()
      n408 = local write "切换量程连续测两次"(FALSE ("切换量程连续测两次")) -> ()
      n409 = Build Path(base path=w579, name or relative path="data\\sys.ini" ("名称或相对路径")) -> (appended path=w577:path)
      n410 = call <vilib>:"Open Config Data.vi"("configuration file path"=w577) -> ("error out"=w573:errorcluster, "refnum"=w576:T5)  [unwired: 8 in, 1 out]
      n411 = vi-ref "斯坦道CODMn.lvlib:CODMn断电保存全局变量.vi"() -> (w575:refnum<vi>)
      n412 = call <userlib>:"Read Panel from INI__ogtk.vi"("error in (no error)"=w573, "VI ref"=w575, "refnum"=w576) -> ("error out"=w572:errorcluster, "refnum out"=w574:T5)  [unwired: 7 in]
      n413 = call <vilib>:"Close Config Data.vi"("error in (no error)"=w572, "refnum"=w574) -> ("error out"=w571:errorcluster, "file path"=w570:path)  [unwired: 8 in]
      n414 = local write "选用水样"(enum16{"葡萄糖", "草酸钠"}."葡萄糖" ("选用水样")) -> ()
      n415 = local write "量程选择"(enum16{"低量程", "高量程", "0-2量程"}."低量程" ("量程选择")) -> ()
      n416 = Open/Create/Replace File(file path (use dialog)=w570, error in=w571) -> (error out=w569:errorcluster)  [unwired: 4 in, 2 out]
      "稀释倍数解释" <- "稀释倍数解释：\n稀释倍数选择1，表示不稀释\n默认低量程系数倍数1，高量程系数倍数2\n则低量程为0~8，高量程为0~16" ("稀释倍数解释")
    }
  }
  n417 = vi-ref "CODMn通讯.vi"() -> (w9:refnum<vi>)
  n418 = property class="VI"(reference=w9) -> ("Name"=w2:string)  [unwired: 1 in, 2 out]
  n419 = Open VI Reference(type specifier VI Refnum (for type only)=refnum<vi> refnum, vi path=w2, options=128 ("选项")) -> (vi reference=w4:refnum<vi>, error out=w6:errorcluster)  [unwired: 3 in]
  n420 = call-by-ref "?"(reference=w4, error in=w6) -> (reference out=w8:refnum<vi>, error out=w7:errorcluster)  [unwired: 12 in]
  n421 = Close Reference(reference=w8, error in (no error)=w7) -> ()  [unwired: 1 out]
  n422 = Obtain Queue(name (unnamed)="CODMn" ("名称（未命名）"), element data type=cluster{"命令":string} {"命令"="启用模块"} ("元素")) -> (queue out=w11:refnum<queue>, error out=w10:errorcluster)  [unwired: 3 in, 1 out]
  n423 = while {
    stop <- FALSE stop-if-true
    n424 = local read "多列列表框"() -> (w590:i32)
    n425 = Equal?(x=w590, y=0) -> (x = y?=w588:bool)
    n426 = call <vilib>:"Boolean Crossing PtByPt.vi"("direction"=enum16{"either", "false-true", "true-false"}."false-true", "input"=w588) -> ("crossing"=w586:bool)  [unwired: 1 in]
    n427 = Wait (ms)(milliseconds to wait=u32 1000 ("等待时间（毫秒）")) -> ()  [unwired: 1 out]
    n428 = case shown="真" w586 {
      frame False {
      }
      frame True {
        n429 = flat-sequence {
          frame #0 {
            n430 = global read "COD读取DATA全局.vi" "数据存储"() -> (w596:u16[])
            n431 = To Word Integer(number=w596) -> (16bit integer=w612:i16[])
            n432 = Split 1D Array(array=w612, index=3 ("索引")) -> (first subarray=w646:i16[], second subarray=w636:i16[])
            n433 = Index Array(array=w646) -> (element #1=w644:i16, element #2=w643:i16, element #3=w642:i16)  [unwired: 3 in]
            n434 = Index Array(array=w636) -> (element #1=w616:i16, element #2=w640:i16, element #3=w639:i16, element #4=w638:i16, element #5=w637:i16, element #7=w594:i16)  [unwired: 7 in, 1 out]
            n435 = global read "COD读取DATA全局.vi" "数据存储时间戳"() -> (w593:timestamp)
            n436 = To Single Precision Float(number=w616) -> (single precision float=w618:sgl)
            n437 = To Single Precision Float(number=w640) -> (single precision float=w627:sgl)
            n438 = To Single Precision Float(number=w594) -> (single precision float=w621:sgl)
            n439 = Build Array(w644, w643, w642) -> (w641:i16[])
            n440 = To Single Precision Float(number=w639) -> (single precision float=w628:sgl)
            n441 = To Single Precision Float(number=w638) -> (single precision float=w629:sgl)
            n442 = To Single Precision Float(number=w637) -> (single precision float=w633:sgl)
            n443 = call "HexToDate.vi"("数组"=w641) -> ("DATE"=w645:timestamp[])  [unwired: 10 in]
            n444 = Divide(x=w618, y=sgl 100.0) -> (x/y=w617:sgl)
            n445 = Divide(x=w633, y=sgl 1000.0) -> (x/y=w630:sgl)
            n446 = global read "CODMN外部API.vi" "CODMn外围API"() -> (w604:T14)
            n447 = Index Array(array=w645) -> (element=w600:timestamp)  [unwired: 1 in]
            n448 = Greater Than 0?(x="量程切换次数") -> (x > 0?=w606:bool)
            n449 = Not Equal?(x=w593, y=w600) -> (x != y?=w599:bool)
            n450 = Less Or Equal?(x=w617, y=sgl 0.01) -> (x <= y?=w619:bool)
            n451 = Unbundle By Name(w604) -> ("运行模式"=w603:enum16{"维护模式", "常规模式", "应急模式", "质控模式"})
            n452 = case "条件结构" shown="真" w599 {
              tunnel: w600 -> [w648 _]
              tunnel: w593 -> [_ w649]
              tunnel: [w648 w649] -> w597
              frame False {
              }
              frame True {
                # "防止下位机PLC数据时间戳不更新"
              }
            }
            n453 = case shown="假" w619 {
              tunnel: [w665 w666] -> w595
              tunnel: w617 -> [w665 _]
              frame False {
              }
              frame True {
                n454 = Random Number (0-1)() -> (number: 0 to 1=w669:dbl)
                n455 = Increment(x=w669) -> (x+1=w667:dbl)
                n456 = Divide(x=w667, y=sgl 100.0) -> (x/y=w666:dbl)
              }
            }
            "COD浓度（mg/L)" <- w595
            n457 = global read "COD测量模式全局.vi" "测量模式"() -> (w601:string)
            n458 = case shown="\"应急模式\"" w603 {
              tunnel: ["M" ("单位") "N" ("单位") "N" ("单位") "N" ("单位")] -> w623
              frame "维护模式", Default {
              }
              frame "常规模式" {
              }
              frame "应急模式" {
              }
              frame "质控模式" {
              }
            }
            n459 = global read "COD测量模式全局.vi" "测量模式"() -> (w611:string)
            n460 = local read "故障标记"() -> (w609:bool)
            n461 = Format Date/Time String(seconds (now)=w597) -> (date/time string=→"数据时间":string)  [unwired: 2 in]
            n462 = case shown="\"跨度核查\"" w611 {
              tunnel: [w655 w656 w657] -> w610
              frame "", Default {
                n463 = local read "标准液浓度"() -> (w655:dbl)
              }
              frame "标样核查", "校标" {
                n464 = local read "标准液浓度"() -> (w656:dbl)
              }
              frame "跨度核查" {
                n465 = local read "跨度液浓度"() -> (w657:dbl)
              }
            }
            n466 = case shown="假" w609 {
              tunnel: [w651 "D" ("数据标识")] -> w625
              frame False {
                n467 = global read "CODMN外部API.vi" "手动启动CODMn"() -> (w650:bool)
                n468 = case shown="假" w650 {
                  tunnel: ["N" ("数据标识") "hd" ("数据标识")] -> w651
                  frame False {
                  }
                  frame True {
                  }
                }
              }
              frame True {
              }
            }
            n469 = global write "COD浓度全局变量.vi" "COD浓度（mg/L)"(w595) -> ()
            n470 = global read "COD浓度全局变量.vi" "基本量程"() -> (w602:enum16{"10mg/L", "20mg/L"})
            n471 = Format Into String(format string="w%05d" ("格式字符串"), u32 1019 ("因子编码")) -> (resulting string=w626:string)  [unwired: 2 in, 1 out]
            n472 = local read "温度"() -> (w622:dbl)
            n473 = Bundle(cluster=T7 {"时间"=timestamp(0 s since 1904-01-01), "测量模式"="", "数据类型"="", "检测值"=0.0, "单位"="", "数据标识"="", "因子编码"="", "标样参考值"=0.0, "ORP-A"=0.0, "ORP-B"=0.0, "ORP-K"=0.0, "COD滴定值"=0.0, "高锰酸钾滴定数"=0.0, "温度"=0.0, "量程"=0.0} ("data"), "时间"=w597, "测量模式"=w601, "数据类型"=w623, "检测值"=w595, "单位"="mg/L", "数据标识"=w625, "因子编码"=w626, "标样参考值"=w610, "ORP-A"=w627, "ORP-B"=w628, "ORP-K"=w629, "COD滴定值"=w630, "高锰酸钾滴定数"=w621, "温度"=w622, "量程"=w602) -> (w608:T7)
            n474 = case shown="假" w606 {
              tunnel: w595 -> [w675 _]
              tunnel: w608 -> [w674 w730]
              frame False {
                # "量程切换前"
                n475 = case shown="\"自动切换测两次\"" "自动切换量程:" {
                  tunnel: w675 -> [_ w685 w706]
                  tunnel: w674 -> [w677 w681 w705]
                  frame "关闭", Default {
                    # "关闭自动切换量程"
                    n476 = call "存数据cloumns(子VI).vi"() -> ("数组"=w679:string[])  [unwired: 11 in]
                    n477 = global write "COD读取DATA全局.vi" "data"(w677) -> ()
                    n478 = call "数据写入database.vi"("data"=w677, "columns"=w679, "table"="CODMn") -> ()  [unwired: 8 in, 1 out]
                  }
                  frame "自动切换测一次" {
                    # "自动切换量程选择是否重测"
                    n479 = global read "COD测量模式全局.vi" "测量模式"() -> (w688:string)
                    n480 = Not Equal?(x=w688, y="水样测试") -> (x != y?=w686:bool)
                    n481 = case shown="假" w686 {
                      tunnel: [w689 w690] -> w684
                      tunnel: w685 -> [w689 _]
                      frame False {
                      }
                      frame True {
                        n482 = global read "COD读取DATA全局.vi" "测量数据区"() -> (w691:T3)
                        n483 = Unbundle By Name(w691) -> ("水样实测值"=w690:sgl)
                      }
                    }
                    n484 = global read "COD浓度全局变量.vi" "基本量程"() -> (w680:enum16{"10mg/L", "20mg/L"})
                    n485 = case shown="\"20mg/L\"" w680 {
                      tunnel: w684 -> [w692 w698]
                      frame "10mg/L", Default {
                        n486 = Greater?(x=w692, y="低切高阈值:") -> (0:w693:bool)
                        n487 = case shown="假" w693 {
                          frame False {
                          }
                          frame True {
                            n488 = call "CODMnMB_api.vi"("STEP"=enum16{"open", "read", "write", "close"}."write", "values"=u16[] [1], "starting address"=u16 4276) -> ()  [unwired: 5 in, 4 out]
                          }
                        }
                      }
                      frame "20mg/L" {
                        n489 = Less?(x=w698, y="高切低阈值:") -> (x < y?=w699:bool)
                        n490 = case shown="真" w699 {
                          frame False {
                          }
                          frame True {
                            n491 = call "CODMnMB_api.vi"("STEP"=enum16{"open", "read", "write", "close"}."write", "values"=u16[] [0], "starting address"=u16 4276) -> ()  [unwired: 5 in, 4 out]
                          }
                        }
                      }
                    }
                    n492 = call "存数据cloumns(子VI).vi"() -> ("数组"=w683:string[])  [unwired: 11 in]
                    n493 = global write "COD读取DATA全局.vi" "data"(w681) -> ()
                    n494 = call "数据写入database.vi"("data"=w681, "columns"=w683, "table"="CODMn") -> ()  [unwired: 8 in, 1 out]
                  }
                  frame "自动切换测两次" {
                    # "自动切换量程选择是否重测"
                    n495 = global read "COD浓度全局变量.vi" "基本量程"() -> (w704:enum16{"10mg/L", "20mg/L"})
                    n496 = case shown="\"10mg/L\", 默认" w704 {
                      tunnel: w706 -> [w708 w719]
                      tunnel: w705 -> [w707 w718]
                      frame "10mg/L", Default {
                        n497 = local read "低切高阈值:"() -> (w709:dbl)
                        n498 = Greater?(x=w708, y=w709) -> (0:w710:bool)
                        n499 = case shown="真" w710 {
                          tunnel: w707 -> [w711 _]
                          frame False {
                            n500 = call "存数据cloumns(子VI).vi"() -> ("数组"=w713:string[])  [unwired: 11 in]
                            n501 = global write "COD读取DATA全局.vi" "data"(w711) -> ()
                            n502 = call "数据写入database.vi"("data"=w711, "columns"=w713, "table"="CODMn") -> ()  [unwired: 8 in, 1 out]
                          }
                          frame True {
                            n503 = call "CODMnMB_api.vi"("STEP"=enum16{"open", "read", "write", "close"}."write", "values"=u16[] [1], "starting address"=u16 4276) -> ()  [unwired: 5 in, 4 out]
                            "切换量程连续测两次" <- TRUE ("切换量程连续测两次")
                          }
                        }
                      }
                      frame "20mg/L" {
                        n504 = local read "高切低阈值:"() -> (w720:dbl)
                        n505 = Less?(x=w719, y=w720) -> (x < y?=w721:bool)
                        n506 = case shown="假" w721 {
                          tunnel: w718 -> [w722 _]
                          frame False {
                            n507 = call "存数据cloumns(子VI).vi"() -> ("数组"=w724:string[])  [unwired: 11 in]
                            n508 = global write "COD读取DATA全局.vi" "data"(w722) -> ()
                            n509 = call "数据写入database.vi"("data"=w722, "columns"=w724, "table"="CODMn") -> ()  [unwired: 8 in, 1 out]
                          }
                          frame True {
                            n510 = call "CODMnMB_api.vi"("STEP"=enum16{"open", "read", "write", "close"}."write", "values"=u16[] [0], "starting address"=u16 4276) -> ()  [unwired: 5 in, 4 out]
                            n511 = local write "切换量程连续测两次"(TRUE ("切换量程连续测两次")) -> ()
                          }
                        }
                      }
                    }
                  }
                }
              }
              frame True {
                # "防止无限切量程"
                n512 = local write "量程切换次数"(u8 0 ("量程切换次数")) -> ()
                n513 = call "存数据cloumns(子VI).vi"() -> ("数组"=w732:string[])  [unwired: 11 in]
                n514 = call "数据写入database.vi"("data"=w730, "columns"=w732, "table"="CODMn") -> ()  [unwired: 8 in, 1 out]
                n515 = global write "COD读取DATA全局.vi" "data"(w730) -> ()
              }
            }
            n516 = global read "COD测量模式全局.vi" "测量模式"() -> (w615:string)
            n517 = Equal?(x=w615, y="校标") -> (x = y?=w613:bool)
            n518 = case shown="真" w613 {
              tunnel: w621 -> [_ w658]
              frame False {
              }
              frame True {
                n519 = local read "当前校准"() -> (w659:i32)
                n520 = case shown="3" w659 {
                  tunnel: w658 -> [w660 w661 w662 w663 w664]
                  frame 1, Default {
                    n521 = local write "泵滴定数1"(w660) -> ()
                  }
                  frame 2 {
                    n522 = local write "泵滴定数2"(w661) -> ()
                  }
                  frame 3 {
                    n523 = local write "泵滴定数3"(w662) -> ()
                  }
                  frame 4 {
                    n524 = local write "泵滴定数4"(w663) -> ()
                  }
                  frame 5 {
                    n525 = local write "泵滴定数5"(w664) -> ()
                  }
                }
              }
            }
          }
        }
      }
    }
  }
  n526 = while {
    tunnel: w11 -> [w734]
    tunnel: w10 -> [w733]
    stop <- FALSE stop-if-true
    n527 = event shown="[7] \"跨度液浓度\": 值改变" {
      selector: _ -> [_ _ _ _ _ _ _ _ _ _ _ _ _ _ _ _ _ _ _ _ _ _ _ _ _ _ _ _ _ _ _]
      dyn-events: _ -> [_ _ _ _ _ _ _ _ _ _ _ _ _ _ _ _ _ _ _ _ _ _ _ _ _ _ _ _ _ _ _]
      timeout: _ -> [_ _ _ _ _ _ _ _ _ _ _ _ _ _ _ _ _ _ _ _ _ _ _ _ _ _ _ _ _ _ _]
      tunnel: w734 -> [_ _ _ _ _ w823 _ _ _ _ _ _ _ _ _ _ _ _ _ _ _ _ _ _ _ w1426 _ _ _ _ _]
      tunnel: w733 -> [_ _ _ _ _ w822 _ _ _ _ _ _ _ _ _ _ _ _ _ _ _ _ _ _ _ w1425 _ _ _ _ _]
      event "单步启动": Mouse Down {
        n528 = event-data() -> ()  [unwired: 1 in, 8 out]
        n529 = call "单步启动选择对话框.vi"() -> ("启动选择2"=w739:u16)  [unwired: 10 in, 1 out]
        n530 = case shown="3" w739 {
          tunnel: [u16 4610 ("address") u16 4610 ("address") u16 4610 ("address") u16 4610 ("address") u16 4610 ("address") u16 4610 ("address") u16 4610 ("address") u16 4610 ("address") u16 4610 ("address") u16 4610 ("address") u16 4610 ("address") u16 4610 ("address") u16 4610 ("address")] -> w737
          tunnel: [u16 1 ("address") u16 2 ("address") u16 3 ("address") u16 4 ("address") u16 5 ("address") u16 6 ("address") u16 7 ("address") u16 8 ("address") u16 9 ("holding register value") u16 10 ("holding register value") u16 11 ("holding register value") u16 12 ("address") u16 0 ("address")] -> w740
          frame 0 {
          }
          frame 1 {
          }
          frame 2 {
          }
          frame 3 {
          }
          frame 4 {
          }
          frame 5 {
          }
          frame 6 {
          }
          frame 7 {
          }
          frame 8 {
          }
          frame 9 {
          }
          frame 10 {
          }
          frame 11 {
          }
          frame 12, Default {
          }
        }
        n531 = Insert Into Array(array=u16[] [] ("values"), index=0 ("索引"), new element=w740) -> (w736:u16[])
        n532 = call "CODMnMB_api.vi"("STEP"=enum16{"open", "read", "write", "close"}."write", "values"=w736, "starting address"=w737) -> ()  [unwired: 5 in, 4 out]
      }
      event "启动": Mouse Down {
        n533 = event-data() -> ()  [unwired: 1 in, 8 out]
        n534 = flat-sequence {
          tunnel: [w770] -> w769
          tunnel: w769 -> [w776]
          frame #0 {
            n535 = call "启动测量模式选择对话框.vi"() -> ("启动选择 2"=w770:u16)  [unwired: 11 in]
            "启动选择 2" <- w770
          }
          frame #1 {
            n536 = case shown="9, 默认" w776 {
              tunnel: [u16 4608 ("address") u16 4608 ("address") u16 4608 ("address") u16 4608 ("address") u16 4608 ("address") u16 4608 ("address") u16 4608 ("address") u16 4608 ("address") u16 4608 ("address") u16 4608 ("address")] -> w772
              tunnel: [u16 1 ("address") u16 2 ("address") u16 3 ("address") u16 4 ("address") u16 5 ("address") u16 7 ("address") u16 6 ("address") u16 8 ("address") u16 9 ("address") u16 0 ("address")] -> w777
              frame 0 {
              }
              frame 1 {
              }
              frame 2 {
              }
              frame 3 {
              }
              frame 4 {
              }
              frame 5 {
              }
              frame 6 {
              }
              frame 7 {
              }
              frame 8 {
              }
              frame 9, Default {
              }
            }
            n537 = Not Equal?(x=w776, y=u16 9) -> (x != y?=w774:bool)
            n538 = global write "CODMN外部API.vi" "手动启动CODMn"(w774) -> ()
            n539 = Insert Into Array(array=u16[] [] ("values"), index=0 ("索引"), new element=w777) -> (w771:u16[])
            n540 = call "CODMnMB_api.vi"("STEP"=enum16{"open", "read", "write", "close"}."write", "values"=w771, "starting address"=w772) -> ()  [unwired: 5 in, 4 out]
          }
        }
      }
      event "停止": Value Change {
        n541 = event-data() -> ()  [unwired: 1 in, 6 out]
        n542 = Two Button Dialog(message="确认是否停止？" ("消息"), 1:"否" ("F按钮名称（“取消”）"), 2:"是" ("T按钮名称（“确定”）")) -> (T button?=w802:bool)
        n543 = case shown="真" w802 {
          frame False {
          }
          frame True {
            n544 = call "CODMnMB_api.vi"("STEP"=enum16{"open", "read", "write", "close"}."write", "values"=u16[] [11], "starting address"=u16 4608) -> ()  [unwired: 5 in, 4 out]
          }
        }
      }
      event "手动控制": Value Change {
        n545 = event-data() -> ()  [unwired: 1 in, 6 out]
        n546 = call "数字密码键盘.vi"() -> ("NewNumber"=w807:sgl)  [unwired: 1 in]
        n547 = Equal?(x=w807, y=8.0) -> (x = y?=w808:bool)
        n548 = case shown="真" w808 {
          frame False {
            n549 = call "窗口弹出对话框(子VI).vi"("消息"="密码错误") -> ()  [unwired: 10 in, 1 out]
          }
          frame True {
            n550 = call "CODMn手动控制框.vi"() -> ()  [unwired: 12 in]
          }
        }
      }
      event "锁定按钮": Mouse Down {
        n551 = event-data() -> ("CtlRef"=w813:refnum<vi>)  [unwired: 1 in, 7 out]
        n552 = property class="Bool (严格)"(reference=w813) -> ("Value"=w812:bool)  [unwired: 1 in, 2 out]
        n553 = case shown="真" w812 {
          selector: w812 -> [w814 _]
          tunnel: [w814 w815] -> w811
          frame False {
          }
          frame True {
            n554 = call "数字密码键盘.vi"() -> ("NewNumber"=w816:sgl)  [unwired: 1 in]
            n555 = Equal?(x=w816, y=8.0) -> (x = y?=w815:bool)
            n556 = case shown="假" w815 {
              selector: w815 -> [w819 _]
              frame False {
                n557 = One Button Dialog(message="密码错误!" ("消息")) -> ()  [unwired: 1 in, 1 out]
                n558 = local write "锁定按钮"(w819) -> ()
              }
              frame True {
                n559 = One Button Dialog(message="解锁成功!" ("消息")) -> ()  [unwired: 1 in, 1 out]
              }
            }
          }
        }
        "x = y?" <- w811
      }
      event "参数配置": Value Change {
        (unwired) u16 20 ("number of holding registers")
        (unwired) u16 4272 ("starting address")
        n560 = event-data() -> ()  [unwired: 1 in, 6 out]
        n561 = Bundle By Name(cluster=cluster{"命令":string} {"命令"=""} ("元素"), "命令"="CODMn读取参数" ("名称（未命名）")) -> (w824:cluster{"命令":string})
        n562 = call <vilib>:"Application Directory.vi"() -> ("Application Directory"=w827:path)
        n563 = Enqueue Element(queue=w823, element=w824, error in (no error)=w822) -> ()  [unwired: 1 in, 3 out]
        n564 = Build Path(base path=w827, name or relative path="data\\sys.ini" ("名称或相对路径")) -> (appended path=w829:path)
        n565 = call <vilib>:"Open Config Data.vi"("configuration file path"=w829) -> ("error out"=w833:errorcluster, "refnum"=w830:T5)  [unwired: 8 in, 1 out]
        n566 = property on="窗格" class="Pane"("Origin"=T13 {"Horizontal"=0, "Vertical"=650} ("原点")) -> ()  [unwired: 2 in, 2 out]
        n567 = vi-ref "斯坦道CODMn.lvlib:CODMn断电保存全局变量.vi"() -> (w831:refnum<vi>)
        n568 = call <userlib>:"Read Panel from INI__ogtk.vi"("error in (no error)"=w833, "VI ref"=w831, "refnum"=w830) -> ("error out"=w834:errorcluster, "refnum out"=w832:T5)  [unwired: 7 in]
        n569 = call <vilib>:"Close Config Data.vi"("error in (no error)"=w834, "refnum"=w832) -> ("error out"=w835:errorcluster, "file path"=w836:path)  [unwired: 8 in]
        n570 = Open/Create/Replace File(file path (use dialog)=w836, error in=w835) -> (error out=w821:errorcluster)  [unwired: 4 in, 2 out]
        n571 = call <vilib>:"Clear Errors.vi"("error in (no error)"=w821) -> ()  [unwired: 5 in, 2 out]
      }
      event "保存": Mouse Down {
        n572 = event-data() -> ()  [unwired: 1 in, 8 out]
        n573 = local read "CODMn零点核查选择"() -> (w841:enum16{"零点核查走纯水管", "零点核查走质控管"})
        n574 = Multiply(x="温度", y=10.0) -> (x*y=w850:dbl)
        n575 = Multiply(x="标准液浓度", y=100.0) -> (x*y=w844:dbl)
        n576 = Multiply(x="修正系数", y=100.0) -> (x*y=w847:dbl)
        n577 = Build Array(w850, "恒温时间", w844, w847, "基本量程", "水样", "蒸馏水", "标液", "质控样", "加标回收", "高锰酸钾", "草酸钠", "硫酸", "零点泵计量数 2", "标度泵计量数 2", "高量程稀释倍数:", "低量程稀释倍数:", w841) -> (w838:dbl[])
        n578 = call "CODMnMB_api.vi"("STEP"=enum16{"open", "read", "write", "close"}."write", "values"=w838, "starting address"=u16 4272) -> ()  [unwired: 5 in, 4 out]
      }
      event "跨度液浓度": Value Change {
        n579 = event-data() -> ()  [unwired: 1 in, 6 out]
        n580 = flat-sequence {
          frame #0 {
            n581 = global write "CODMn断电保存全局变量.vi" "跨度液浓度"("跨度液浓度") -> ()
          }
          frame #1 {
            n582 = call <vilib>:"Application Directory.vi"() -> ("Application Directory"=w879:path)
            n583 = Build Path(base path=w879, name or relative path="data\\sys.ini" ("名称或相对路径")) -> (appended path=w877:path)
            n584 = call <vilib>:"Open Config Data.vi"("configuration file path"=w877) -> ("error out"=w873:errorcluster, "refnum"=w876:T5)  [unwired: 8 in, 1 out]
            n585 = vi-ref "斯坦道CODMn.lvlib:CODMn断电保存全局变量.vi"() -> (w875:refnum<vi>)
            n586 = call <userlib>:"Write Panel to INI__ogtk.vi"("error in (no error)"=w873, "VI ref"=w875, "refnum"=w876) -> ("error out"=w872:errorcluster, "refnum out"=w874:T5)  [unwired: 7 in]
            n587 = call <vilib>:"Close Config Data.vi"("error in (no error)"=w872, "refnum"=w874) -> ("error out"=w867:errorcluster, "file path"=w866:path)  [unwired: 8 in]
            n588 = Open/Create/Replace File(file path (use dialog)=w866, error in=w867) -> (refnum out=w870:refnum<file>, error out=w871:errorcluster)  [unwired: 4 in, 1 out]
            n589 = Flush File(refnum=w870, error in=w871) -> (refnum out=w869:refnum<file>, error out=w868:errorcluster)
            n590 = Close File(refnum=w869, error in=w868) -> ()  [unwired: 2 out]
          }
        }
      }
      event "校准配置": Value Change {
        n591 = event-data() -> ()  [unwired: 1 in, 6 out]
        n592 = property on="窗格" class="Pane"("Origin"=T13 {"Horizontal"=0, "Vertical"=1300} ("原点")) -> ()  [unwired: 2 in, 2 out]
        n593 = call <vilib>:"Application Directory.vi"() -> ("Application Directory"=w930:path)
        n594 = Build Path(base path=w930, name or relative path="data\\Set.ini" ("名称或相对路径")) -> (appended path=w928:path)
        n595 = call <vilib>:"Open Config Data.vi"("configuration file path"=w928) -> ("error out"=w898:errorcluster, "refnum"=w899:T5)  [unwired: 8 in, 1 out]
        n596 = call-poly <vilib>:"Read Key.vi"("section"="CODMn模型选择" ("key"), "error in (no error)"=w898, "key"="线性和多项式", "refnum"=w899) -> ("error out"=w894:errorcluster, "value"=w897:i32, "refnum out"=w895:T5)  [unwired: 4 in, 1 out]
        n597 = local write "模型"(w897) -> ()
        n598 = call-poly <vilib>:"Read Key.vi"("section"="标线选择", "error in (no error)"=w894, "key"="选用水样", "refnum"=w895) -> ("error out"=w892:errorcluster, "value"=w896:i32, "refnum out"=w893:T5)  [unwired: 4 in, 1 out]
        n599 = local write "选用水样"(w896) -> ()
        n600 = local read "量程选择"() -> (w905:enum16{"低量程", "高量程", "0-2量程"})
        n601 = case shown="0, 默认" w896 {
          tunnel: ["葡萄糖标线" ("section") "草酸钠标线" ("section")] -> w904
          frame 0, Default {
          }
          frame 1 {
          }
        }
        n602 = case shown="\"0-2量程\"" w905 {
          tunnel: ["低量程" "高量程" "0-2量程"] -> w903
          frame "低量程", Default {
          }
          frame "高量程" {
          }
          frame "0-2量程" {
          }
        }
        n603 = Concatenate Strings(w904, w903) -> (w902:string)
        n604 = call-poly <vilib>:"Read Key.vi"("section"=w902, "error in (no error)"=w892, "key"="浓度1", "refnum"=w893) -> ("error out"=w934:errorcluster, "value"=w932:dbl, "refnum out"=w933:T5)  [unwired: 4 in, 1 out]
        n605 = local write "浓度1"(w932) -> ()
        n606 = call-poly <vilib>:"Read Key.vi"("section"=w902, "error in (no error)"=w934, "key"="浓度2", "refnum"=w933) -> ("error out"=w948:errorcluster, "value"=w935:dbl, "refnum out"=w947:T5)  [unwired: 4 in, 1 out]
        n607 = local write "浓度2"(w935) -> ()
        n608 = call-poly <vilib>:"Read Key.vi"("section"=w902, "error in (no error)"=w948, "key"="浓度3", "refnum"=w947) -> ("error out"=w949:errorcluster, "value"=w937:dbl, "refnum out"=w946:T5)  [unwired: 4 in, 1 out]
        n609 = local write "浓度3"(w937) -> ()
        n610 = call-poly <vilib>:"Read Key.vi"("section"=w902, "error in (no error)"=w949, "key"="泵滴定数1", "refnum"=w946) -> ("error out"=w950:errorcluster, "value"=w939:dbl, "refnum out"=w945:T5)  [unwired: 4 in, 1 out]
        n611 = local write "泵滴定数1"(w939) -> ()
        n612 = call-poly <vilib>:"Read Key.vi"("section"=w902, "error in (no error)"=w950, "key"="泵滴定数2", "refnum"=w945) -> ("error out"=w944:errorcluster, "value"=w942:dbl, "refnum out"=w951:T5)  [unwired: 4 in, 1 out]
        n613 = local write "泵滴定数2"(w942) -> ()
        n614 = call-poly <vilib>:"Read Key.vi"("section"=w902, "error in (no error)"=w944, "key"="泵滴定数3", "refnum"=w951) -> ("error out"=w956:errorcluster, "value"=w955:dbl, "refnum out"=w952:T5)  [unwired: 4 in, 1 out]
        n615 = local write "泵滴定数3"(w955) -> ()
        n616 = call-poly <vilib>:"Read Key.vi"("section"=w902, "error in (no error)"=w956, "key"="浓度4", "refnum"=w952) -> ("error out"=w957:errorcluster, "value"=w885:dbl, "refnum out"=w953:T5)  [unwired: 4 in, 1 out]
        n617 = local write "浓度4"(w885) -> ()
        n618 = call-poly <vilib>:"Read Key.vi"("section"=w902, "error in (no error)"=w957, "key"="浓度5", "refnum"=w953) -> ("error out"=w890:errorcluster, "value"=w884:dbl, "refnum out"=w891:T5)  [unwired: 4 in, 1 out]
        n619 = local write "浓度5"(w884) -> ()
        n620 = call-poly <vilib>:"Read Key.vi"("section"=w902, "error in (no error)"=w890, "key"="泵滴定数4", "refnum"=w891) -> ("error out"=w958:errorcluster, "value"=w883:dbl, "refnum out"=w954:T5)  [unwired: 4 in, 1 out]
        n621 = local write "泵滴定数4"(w883) -> ()
        n622 = call-poly <vilib>:"Read Key.vi"("section"=w902, "error in (no error)"=w958, "key"="泵滴定数5", "refnum"=w954) -> ("error out"=w888:errorcluster, "value"=w882:dbl, "refnum out"=w889:T5)  [unwired: 4 in, 1 out]
        n623 = local write "泵滴定数5"(w882) -> ()
        n624 = call-poly <vilib>:"Read Key.vi"("section"=w902, "error in (no error)"=w888, "key"="当前选用的校准", "refnum"=w889) -> ("error out"=w924:errorcluster, "value"=w926:i32, "refnum out"=w925:T5)  [unwired: 4 in, 1 out]
        n625 = local write "当前校准"(w926) -> ()
        n626 = call-poly <vilib>:"Read Key.vi"("section"=w902, "error in (no error)"=w924, "key"="启用1", "refnum"=w925) -> ("error out"=w921:errorcluster, "value"=w910:bool, "refnum out"=w922:T5)  [unwired: 4 in, 1 out]
        n627 = local write "启用1"(w910) -> ()
        n628 = call-poly <vilib>:"Read Key.vi"("section"=w902, "error in (no error)"=w921, "key"="启用2", "refnum"=w922) -> ("error out"=w919:errorcluster, "value"=w909:bool, "refnum out"=w920:T5)  [unwired: 4 in, 1 out]
        n629 = local write "启用2"(w909) -> ()
        n630 = call-poly <vilib>:"Read Key.vi"("section"=w902, "error in (no error)"=w919, "key"="启用3", "refnum"=w920) -> ("error out"=w917:errorcluster, "value"=w908:bool, "refnum out"=w918:T5)  [unwired: 4 in, 1 out]
        n631 = local write "启用3"(w908) -> ()
        n632 = call-poly <vilib>:"Read Key.vi"("section"=w902, "error in (no error)"=w917, "key"="启用4", "refnum"=w918) -> ("error out"=w915:errorcluster, "value"=w881:bool, "refnum out"=w916:T5)  [unwired: 4 in, 1 out]
        n633 = local write "启用4"(w881) -> ()
        n634 = call-poly <vilib>:"Read Key.vi"("section"=w902, "error in (no error)"=w915, "key"="启用5", "refnum"=w916) -> ("error out"=w886:errorcluster, "value"=w880:bool, "refnum out"=w887:T5)  [unwired: 4 in, 1 out]
        n635 = local write "启用5"(w880) -> ()
        n636 = call <vilib>:"Close Config Data.vi"("error in (no error)"=w886, "refnum"=w887) -> ()  [unwired: 8 in, 2 out]
      }
      event "选用水样": Value Change {
        (unwired) "浓度6" ("key")
        n637 = event-data() -> ()  [unwired: 1 in, 6 out]
        n638 = property on="窗格" class="Pane"("Origin"=T13 {"Horizontal"=0, "Vertical"=1300} ("原点")) -> ()  [unwired: 2 in, 2 out]
        n639 = local read "量程选择"() -> (w982:enum16{"低量程", "高量程", "0-2量程"})
        n640 = case shown="\"0-2量程\"" w982 {
          tunnel: ["低量程" "高量程" "0-2量程"] -> w983
          frame "低量程", Default {
          }
          frame "高量程" {
          }
          frame "0-2量程" {
          }
        }
        n641 = case shown="\"葡萄糖\", 默认" "选用水样" {
          tunnel: ["葡萄糖标线" ("section") "草酸钠标线" ("section")] -> w984
          frame "葡萄糖", Default {
          }
          frame "草酸钠" {
          }
        }
        n642 = call <vilib>:"Application Directory.vi"() -> ("Application Directory"=w1008:path)
        n643 = Build Path(base path=w1008, name or relative path="data\\Set.ini" ("名称或相对路径")) -> (appended path=w1006:path)
        n644 = call <vilib>:"Open Config Data.vi"("configuration file path"=w1006) -> ("error out"=w1009:errorcluster, "refnum"=w1010:T5)  [unwired: 8 in, 1 out]
        n645 = Concatenate Strings(w984, w983) -> (w981:string)
        n646 = call-poly <vilib>:"Read Key.vi"("section"=w981, "error in (no error)"=w1009, "key"="浓度1", "refnum"=w1010) -> ("error out"=w1014:errorcluster, "value"=w1012:dbl, "refnum out"=w1013:T5)  [unwired: 4 in, 1 out]
        n647 = local write "浓度1"(w1012) -> ()
        n648 = call-poly <vilib>:"Read Key.vi"("section"=w981, "error in (no error)"=w1014, "key"="浓度2", "refnum"=w1013) -> ("error out"=w1028:errorcluster, "value"=w1015:dbl, "refnum out"=w1027:T5)  [unwired: 4 in, 1 out]
        n649 = local write "浓度2"(w1015) -> ()
        n650 = call-poly <vilib>:"Read Key.vi"("section"=w981, "error in (no error)"=w1028, "key"="浓度3", "refnum"=w1027) -> ("error out"=w1029:errorcluster, "value"=w1017:dbl, "refnum out"=w1026:T5)  [unwired: 4 in, 1 out]
        n651 = local write "浓度3"(w1017) -> ()
        n652 = call-poly <vilib>:"Read Key.vi"("section"=w981, "error in (no error)"=w1029, "key"="泵滴定数1", "refnum"=w1026) -> ("error out"=w1030:errorcluster, "value"=w1019:dbl, "refnum out"=w1025:T5)  [unwired: 4 in, 1 out]
        n653 = local write "泵滴定数1"(w1019) -> ()
        n654 = call-poly <vilib>:"Read Key.vi"("section"=w981, "error in (no error)"=w1030, "key"="泵滴定数2", "refnum"=w1025) -> ("error out"=w1024:errorcluster, "value"=w1022:dbl, "refnum out"=w1031:T5)  [unwired: 4 in, 1 out]
        n655 = local write "泵滴定数2"(w1022) -> ()
        n656 = call-poly <vilib>:"Read Key.vi"("section"=w981, "error in (no error)"=w1024, "key"="泵滴定数3", "refnum"=w1031) -> ("error out"=w1036:errorcluster, "value"=w1035:dbl, "refnum out"=w1032:T5)  [unwired: 4 in, 1 out]
        n657 = local write "泵滴定数3"(w1035) -> ()
        n658 = call-poly <vilib>:"Read Key.vi"("section"=w981, "error in (no error)"=w1036, "key"="浓度4", "refnum"=w1032) -> ("error out"=w1037:errorcluster, "value"=w976:dbl, "refnum out"=w1033:T5)  [unwired: 4 in, 1 out]
        n659 = local write "浓度4"(w976) -> ()
        n660 = call-poly <vilib>:"Read Key.vi"("section"=w981, "error in (no error)"=w1037, "key"="浓度5", "refnum"=w1033) -> ("error out"=w979:errorcluster, "value"=w975:dbl, "refnum out"=w980:T5)  [unwired: 4 in, 1 out]
        n661 = local write "浓度5"(w975) -> ()
        n662 = call-poly <vilib>:"Read Key.vi"("section"=w981, "error in (no error)"=w979, "key"="泵滴定数4", "refnum"=w980) -> ("error out"=w1038:errorcluster, "value"=w974:dbl, "refnum out"=w1034:T5)  [unwired: 4 in, 1 out]
        n663 = local write "泵滴定数4"(w974) -> ()
        n664 = call-poly <vilib>:"Read Key.vi"("section"=w981, "error in (no error)"=w1038, "key"="泵滴定数5", "refnum"=w1034) -> ("error out"=w977:errorcluster, "value"=w973:dbl, "refnum out"=w978:T5)  [unwired: 4 in, 1 out]
        n665 = local write "泵滴定数5"(w973) -> ()
        n666 = call-poly <vilib>:"Read Key.vi"("section"=w981, "error in (no error)"=w977, "key"="当前选用的校准", "refnum"=w978) -> ("error out"=w1002:errorcluster, "value"=w1004:i32, "refnum out"=w1003:T5)  [unwired: 4 in, 1 out]
        n667 = local write "当前校准"(w1004) -> ()
        n668 = call-poly <vilib>:"Read Key.vi"("section"=w981, "error in (no error)"=w1002, "key"="启用1", "refnum"=w1003) -> ("error out"=w999:errorcluster, "value"=w988:bool, "refnum out"=w1000:T5)  [unwired: 4 in, 1 out]
        n669 = local write "启用1"(w988) -> ()
        n670 = call-poly <vilib>:"Read Key.vi"("section"=w981, "error in (no error)"=w999, "key"="启用2", "refnum"=w1000) -> ("error out"=w997:errorcluster, "value"=w987:bool, "refnum out"=w998:T5)  [unwired: 4 in, 1 out]
        n671 = local write "启用2"(w987) -> ()
        n672 = call-poly <vilib>:"Read Key.vi"("section"=w981, "error in (no error)"=w997, "key"="启用3", "refnum"=w998) -> ("error out"=w995:errorcluster, "value"=w986:bool, "refnum out"=w996:T5)  [unwired: 4 in, 1 out]
        n673 = local write "启用3"(w986) -> ()
        n674 = call-poly <vilib>:"Read Key.vi"("section"=w981, "error in (no error)"=w995, "key"="启用4", "refnum"=w996) -> ("error out"=w993:errorcluster, "value"=w970:bool, "refnum out"=w994:T5)  [unwired: 4 in, 1 out]
        n675 = local write "启用4"(w970) -> ()
        n676 = call-poly <vilib>:"Read Key.vi"("section"=w981, "error in (no error)"=w993, "key"="启用5", "refnum"=w994) -> ("error out"=w971:errorcluster, "value"=w969:bool, "refnum out"=w972:T5)  [unwired: 4 in, 1 out]
        n677 = local write "启用5"(w969) -> ()
        n678 = call <vilib>:"Close Config Data.vi"("error in (no error)"=w971, "refnum"=w972) -> ()  [unwired: 8 in, 2 out]
      }
      event "量程选择": Value Change {
        n679 = event-data() -> ()  [unwired: 1 in, 6 out]
        n680 = property on="窗格" class="Pane"("Origin"=T13 {"Horizontal"=0, "Vertical"=1300} ("原点")) -> ()  [unwired: 2 in, 2 out]
        n681 = local read "选用水样"() -> (w1065:enum16{"葡萄糖", "草酸钠"})
        n682 = case shown="\"葡萄糖\", 默认" w1065 {
          tunnel: ["葡萄糖标线" ("section") "草酸钠标线" ("section")] -> w1064
          frame "葡萄糖", Default {
          }
          frame "草酸钠" {
          }
        }
        n683 = case shown="\"0-2量程\"" "量程选择" {
          tunnel: ["低量程" "高量程" "0-2量程"] -> w1061
          frame "低量程", Default {
          }
          frame "高量程" {
          }
          frame "0-2量程" {
          }
        }
        n684 = call <vilib>:"Application Directory.vi"() -> ("Application Directory"=w1088:path)
        n685 = Build Path(base path=w1088, name or relative path="data\\Set.ini" ("名称或相对路径")) -> (appended path=w1086:path)
        n686 = call <vilib>:"Open Config Data.vi"("configuration file path"=w1086) -> ("error out"=w1089:errorcluster, "refnum"=w1090:T5)  [unwired: 8 in, 1 out]
        n687 = Concatenate Strings(w1064, w1061) -> (w1063:string)
        n688 = call-poly <vilib>:"Read Key.vi"("section"=w1063, "error in (no error)"=w1089, "key"="浓度1", "refnum"=w1090) -> ("error out"=w1094:errorcluster, "value"=w1092:dbl, "refnum out"=w1093:T5)  [unwired: 4 in, 1 out]
        n689 = local write "浓度1"(w1092) -> ()
        n690 = call-poly <vilib>:"Read Key.vi"("section"=w1063, "error in (no error)"=w1094, "key"="浓度2", "refnum"=w1093) -> ("error out"=w1108:errorcluster, "value"=w1095:dbl, "refnum out"=w1107:T5)  [unwired: 4 in, 1 out]
        n691 = local write "浓度2"(w1095) -> ()
        n692 = call-poly <vilib>:"Read Key.vi"("section"=w1063, "error in (no error)"=w1108, "key"="浓度3", "refnum"=w1107) -> ("error out"=w1109:errorcluster, "value"=w1097:dbl, "refnum out"=w1106:T5)  [unwired: 4 in, 1 out]
        n693 = local write "浓度3"(w1097) -> ()
        n694 = call-poly <vilib>:"Read Key.vi"("section"=w1063, "error in (no error)"=w1109, "key"="泵滴定数1", "refnum"=w1106) -> ("error out"=w1110:errorcluster, "value"=w1099:dbl, "refnum out"=w1105:T5)  [unwired: 4 in, 1 out]
        n695 = local write "泵滴定数1"(w1099) -> ()
        n696 = call-poly <vilib>:"Read Key.vi"("section"=w1063, "error in (no error)"=w1110, "key"="泵滴定数2", "refnum"=w1105) -> ("error out"=w1104:errorcluster, "value"=w1102:dbl, "refnum out"=w1111:T5)  [unwired: 4 in, 1 out]
        n697 = local write "泵滴定数2"(w1102) -> ()
        n698 = call-poly <vilib>:"Read Key.vi"("section"=w1063, "error in (no error)"=w1104, "key"="泵滴定数3", "refnum"=w1111) -> ("error out"=w1116:errorcluster, "value"=w1115:dbl, "refnum out"=w1112:T5)  [unwired: 4 in, 1 out]
        n699 = local write "泵滴定数3"(w1115) -> ()
        n700 = call-poly <vilib>:"Read Key.vi"("section"=w1063, "error in (no error)"=w1116, "key"="浓度4", "refnum"=w1112) -> ("error out"=w1117:errorcluster, "value"=w1052:dbl, "refnum out"=w1113:T5)  [unwired: 4 in, 1 out]
        n701 = local write "浓度4"(w1052) -> ()
        n702 = call-poly <vilib>:"Read Key.vi"("section"=w1063, "error in (no error)"=w1117, "key"="浓度5", "refnum"=w1113) -> ("error out"=w1059:errorcluster, "value"=w1051:dbl, "refnum out"=w1060:T5)  [unwired: 4 in, 1 out]
        n703 = local write "浓度5"(w1051) -> ()
        n704 = call-poly <vilib>:"Read Key.vi"("section"=w1063, "error in (no error)"=w1059, "key"="泵滴定数4", "refnum"=w1060) -> ("error out"=w1118:errorcluster, "value"=w1050:dbl, "refnum out"=w1114:T5)  [unwired: 4 in, 1 out]
        n705 = local write "泵滴定数4"(w1050) -> ()
        n706 = call-poly <vilib>:"Read Key.vi"("section"=w1063, "error in (no error)"=w1118, "key"="泵滴定数5", "refnum"=w1114) -> ("error out"=w1057:errorcluster, "value"=w1049:dbl, "refnum out"=w1058:T5)  [unwired: 4 in, 1 out]
        n707 = local write "泵滴定数5"(w1049) -> ()
        n708 = call-poly <vilib>:"Read Key.vi"("section"=w1063, "error in (no error)"=w1057, "key"="当前选用的校准", "refnum"=w1058) -> ("error out"=w1082:errorcluster, "value"=w1084:i32, "refnum out"=w1083:T5)  [unwired: 4 in, 1 out]
        n709 = local write "当前校准"(w1084) -> ()
        n710 = call-poly <vilib>:"Read Key.vi"("section"=w1063, "error in (no error)"=w1082, "key"="启用1", "refnum"=w1083) -> ("error out"=w1079:errorcluster, "value"=w1068:bool, "refnum out"=w1080:T5)  [unwired: 4 in, 1 out]
        n711 = local write "启用1"(w1068) -> ()
        n712 = call-poly <vilib>:"Read Key.vi"("section"=w1063, "error in (no error)"=w1079, "key"="启用2", "refnum"=w1080) -> ("error out"=w1077:errorcluster, "value"=w1067:bool, "refnum out"=w1078:T5)  [unwired: 4 in, 1 out]
        n713 = local write "启用2"(w1067) -> ()
        n714 = call-poly <vilib>:"Read Key.vi"("section"=w1063, "error in (no error)"=w1077, "key"="启用3", "refnum"=w1078) -> ("error out"=w1075:errorcluster, "value"=w1066:bool, "refnum out"=w1076:T5)  [unwired: 4 in, 1 out]
        n715 = local write "启用3"(w1066) -> ()
        n716 = call-poly <vilib>:"Read Key.vi"("section"=w1063, "error in (no error)"=w1075, "key"="启用4", "refnum"=w1076) -> ("error out"=w1073:errorcluster, "value"=w1054:bool, "refnum out"=w1074:T5)  [unwired: 4 in, 1 out]
        n717 = local write "启用4"(w1054) -> ()
        n718 = call-poly <vilib>:"Read Key.vi"("section"=w1063, "error in (no error)"=w1073, "key"="启用5", "refnum"=w1074) -> ("error out"=w1055:errorcluster, "value"=w1053:bool, "refnum out"=w1056:T5)  [unwired: 4 in, 1 out]
        n719 = local write "启用5"(w1053) -> ()
        n720 = call <vilib>:"Close Config Data.vi"("error in (no error)"=w1055, "refnum"=w1056) -> ()  [unwired: 8 in, 2 out]
      }
      event "周期设置": Value Change {
        n721 = event-data() -> ()  [unwired: 1 in, 6 out]
        n722 = call "数字密码键盘.vi"() -> ("NewNumber"=w1129:sgl)  [unwired: 1 in]
        n723 = Equal?(x=w1129, y=8.0) -> (x = y?=w1130:bool)
        n724 = case shown="真" w1130 {
          frame False {
            n725 = call "窗口弹出对话框(子VI).vi"("消息"="密码错误") -> ()  [unwired: 10 in, 1 out]
          }
          frame True {
            n726 = call "窗口弹出对话框(子VI).vi"("消息"="登录成功") -> ("true"=w1133:bool)  [unwired: 10 in]
            n727 = case shown="真" w1133 {
              frame False {
              }
              frame True {
                n728 = property on="窗格" class="Pane"("Origin"=T13 {"Horizontal"=0, "Vertical"=1950} ("原点")) -> ()  [unwired: 2 in, 2 out]
              }
            }
          }
        }
      }
      event "返回": Value Change {
        (unwired) "泵滴定数6" ("key")
        w1149 = "CODMn" ("section")
        n729 = event-data() -> ()  [unwired: 1 in, 6 out]
        n730 = property on="窗格" class="Pane"("Origin"=T13 {"Horizontal"=0, "Vertical"=0} ("原点")) -> ()  [unwired: 2 in, 2 out]
        n731 = call <vilib>:"Application Directory.vi"() -> ("Application Directory"=w1202:path)
        n732 = Build Path(base path=w1202, name or relative path="data\\Set.ini" ("名称或相对路径")) -> (appended path=w1200:path)
        n733 = call <vilib>:"Open Config Data.vi"("configuration file path"=w1200) -> ("error out"=w1198:errorcluster, "refnum"=w1199:T5)  [unwired: 8 in, 1 out]
        n734 = local read "浓度1"() -> (w1196:dbl)
        n735 = local read "浓度2"() -> (w1180:dbl)
        n736 = call-poly <vilib>:"Write Key.vi"("section"=w1149, "error in (no error)"=w1198, "value"=w1196, "key"="浓度1", "refnum"=w1199) -> ("error out"=w1195:errorcluster, "refnum out"=w1194:T5)  [unwired: 4 in, 1 out]
        n737 = local read "浓度3"() -> (w1176:dbl)
        n738 = call-poly <vilib>:"Write Key.vi"("section"=w1149, "error in (no error)"=w1195, "value"=w1180, "key"="浓度2", "refnum"=w1194) -> ("error out"=w1193:errorcluster, "refnum out"=w1192:T5)  [unwired: 4 in, 1 out]
        n739 = local read "泵滴定数1"() -> (w1174:dbl)
        n740 = call-poly <vilib>:"Write Key.vi"("section"=w1149, "error in (no error)"=w1193, "value"=w1176, "key"="浓度3", "refnum"=w1192) -> ("error out"=w1191:errorcluster, "refnum out"=w1190:T5)  [unwired: 4 in, 1 out]
        n741 = call-poly <vilib>:"Write Key.vi"("section"=w1149, "error in (no error)"=w1191, "value"=w1174, "key"="泵滴定数1", "refnum"=w1190) -> ("error out"=w1189:errorcluster, "refnum out"=w1188:T5)  [unwired: 4 in, 1 out]
        n742 = local read "泵滴定数2"() -> (w1172:dbl)
        n743 = call-poly <vilib>:"Write Key.vi"("section"=w1149, "error in (no error)"=w1189, "value"=w1172, "key"="泵滴定数2", "refnum"=w1188) -> ("error out"=w1187:errorcluster, "refnum out"=w1186:T5)  [unwired: 4 in, 1 out]
        n744 = local read "泵滴定数3"() -> (w1170:dbl)
        n745 = local read "浓度4"() -> (w1137:dbl)
        n746 = call-poly <vilib>:"Write Key.vi"("section"=w1149, "error in (no error)"=w1187, "value"=w1170, "key"="泵滴定数3", "refnum"=w1186) -> ("error out"=w1185:errorcluster, "refnum out"=w1184:T5)  [unwired: 4 in, 1 out]
        n747 = call-poly <vilib>:"Write Key.vi"("section"=w1149, "error in (no error)"=w1185, "value"=w1137, "key"="浓度4", "refnum"=w1184) -> ("error out"=w1178:errorcluster, "refnum out"=w1179:T5)  [unwired: 4 in, 1 out]
        n748 = local read "浓度5"() -> (w1136:dbl)
        n749 = call-poly <vilib>:"Write Key.vi"("section"=w1149, "error in (no error)"=w1178, "value"=w1136, "key"="浓度5", "refnum"=w1179) -> ("error out"=w1146:errorcluster, "refnum out"=w1147:T5)  [unwired: 4 in, 1 out]
        n750 = local read "泵滴定数4"() -> (w1138:dbl)
        n751 = call-poly <vilib>:"Write Key.vi"("section"=w1149, "error in (no error)"=w1146, "value"=w1138, "key"="泵滴定数4", "refnum"=w1147) -> ("error out"=w1183:errorcluster, "refnum out"=w1182:T5)  [unwired: 4 in, 1 out]
        n752 = local read "泵滴定数5"() -> (w1139:dbl)
        n753 = call-poly <vilib>:"Write Key.vi"("section"=w1149, "error in (no error)"=w1183, "value"=w1139, "key"="泵滴定数5", "refnum"=w1182) -> ("error out"=w1144:errorcluster, "refnum out"=w1145:T5)  [unwired: 4 in, 1 out]
        n754 = local read "启用1"() -> (w1158:bool)
        n755 = call-poly <vilib>:"Write Key.vi"("section"=w1149, "error in (no error)"=w1144, "value"=w1158, "key"="启用1", "refnum"=w1145) -> ("error out"=w1154:errorcluster, "refnum out"=w1157:T5)  [unwired: 4 in, 1 out]
        n756 = local read "启用2"() -> (w1155:bool)
        n757 = call-poly <vilib>:"Write Key.vi"("section"=w1149, "error in (no error)"=w1154, "value"=w1155, "key"="启用2", "refnum"=w1157) -> ("error out"=w1165:errorcluster, "refnum out"=w1164:T5)  [unwired: 4 in, 1 out]
        n758 = local read "启用3"() -> (w1153:bool)
        n759 = call-poly <vilib>:"Write Key.vi"("section"=w1149, "error in (no error)"=w1165, "value"=w1153, "key"="启用3", "refnum"=w1164) -> ("error out"=w1163:errorcluster, "refnum out"=w1162:T5)  [unwired: 4 in, 1 out]
        n760 = local read "启用4"() -> (w1141:bool)
        n761 = call-poly <vilib>:"Write Key.vi"("section"=w1149, "error in (no error)"=w1163, "value"=w1141, "key"="启用4", "refnum"=w1162) -> ("error out"=w1161:errorcluster, "refnum out"=w1160:T5)  [unwired: 4 in, 1 out]
        n762 = local read "启用5"() -> (w1140:bool)
        n763 = call-poly <vilib>:"Write Key.vi"("section"=w1149, "error in (no error)"=w1161, "value"=w1140, "key"="启用5", "refnum"=w1160) -> ("error out"=w1142:errorcluster, "refnum out"=w1143:T5)  [unwired: 4 in, 1 out]
        n764 = call <vilib>:"Close Config Data.vi"("error in (no error)"=w1142, "refnum"=w1143) -> ()  [unwired: 8 in, 2 out]
      }
      event "关闭", "关闭 2", "关闭 3": Value Change {
        n765 = event-data() -> ()  [unwired: 1 in, 6 out]
        n766 = property on="窗格" class="Pane"("Origin"=T13 {"Horizontal"=0, "Vertical"=0} ("原点")) -> ()  [unwired: 2 in, 2 out]
      }
      event Application Instance Close {
        n767 = event-data() -> ()  [unwired: 1 in, 4 out]
      }
      event "时间校准": Value Change {
        n768 = event-data() -> ()  [unwired: 1 in, 6 out]
        n769 = flat-sequence {
          frame #0 {
            n770 = Get Date/Time In Seconds() -> (seconds since 1Jan1904=w1211:timestamp)
            n771 = Build Array(w1211) -> (w1210:timestamp[])
            n772 = call "DateToHex.vi"("DATE"=w1210) -> ("数组"=w1208:u16[])  [unwired: 10 in]
            n773 = Insert Into Array(array=u16[] [1] ("values"), index=1 ("索引"), new element=w1208) -> (w1204:u16[])
            n774 = call "CODMnMB_api.vi"("STEP"=enum16{"open", "read", "write", "close"}."write", "values"=w1204, "starting address"=u16 4612) -> ()  [unwired: 5 in, 4 out]
          }
        }
      }
      event "故障清除": Value Change {
        n775 = event-data() -> ()  [unwired: 1 in, 6 out]
        n776 = call "CODMnMB_api.vi"("STEP"=enum16{"open", "read", "write", "close"}."write", "values"=u16[] [1], "starting address"=u16 4611) -> ()  [unwired: 5 in, 4 out]
      }
      event "定时启动": Mouse Down {
        n777 = event-data() -> ()  [unwired: 1 in, 8 out]
        n778 = flat-sequence {
          frame #0 {
            n779 = global read "CODMn断电保存全局变量.vi" "定时控制"() -> (w1215:T11)
            n780 = call "周期设置.vi"("定时控制参数输入"=w1215) -> ("定时控制参数输出"=w1216:T11)  [unwired: 10 in]
            n781 = global write "CODMn断电保存全局变量.vi" "定时控制"(w1216) -> ()
          }
          frame #1 {
            n782 = call <vilib>:"Application Directory.vi"() -> ("Application Directory"=w1230:path)
            n783 = Build Path(base path=w1230, name or relative path="data\\sys.ini" ("名称或相对路径")) -> (appended path=w1228:path)
            n784 = call <vilib>:"Open Config Data.vi"("configuration file path"=w1228) -> ("error out"=w1224:errorcluster, "refnum"=w1227:T5)  [unwired: 8 in, 1 out]
            n785 = vi-ref "斯坦道CODMn.lvlib:CODMn断电保存全局变量.vi"() -> (w1226:refnum<vi>)
            n786 = call <userlib>:"Write Panel to INI__ogtk.vi"("error in (no error)"=w1224, "VI ref"=w1226, "refnum"=w1227) -> ("error out"=w1223:errorcluster, "refnum out"=w1225:T5)  [unwired: 7 in]
            n787 = call <vilib>:"Close Config Data.vi"("error in (no error)"=w1223, "refnum"=w1225) -> ("error out"=w1218:errorcluster, "file path"=w1217:path)  [unwired: 8 in]
            n788 = Open/Create/Replace File(file path (use dialog)=w1217, error in=w1218) -> (refnum out=w1221:refnum<file>, error out=w1222:errorcluster)  [unwired: 4 in, 1 out]
            n789 = Flush File(refnum=w1221, error in=w1222) -> (refnum out=w1220:refnum<file>, error out=w1219:errorcluster)
            n790 = Close File(refnum=w1220, error in=w1219) -> ()  [unwired: 2 out]
          }
        }
      }
      event "测量模式(公式)": Value Change {
        n791 = event-data() -> ()  [unwired: 1 in, 6 out]
        n792 = flat-sequence {
          frame #0 {
            n793 = global write "CODMn断电保存全局变量.vi" "测量模式(公式)"("测量模式(公式)") -> ()
          }
          frame #1 {
            n794 = call <vilib>:"Application Directory.vi"() -> ("Application Directory"=w1245:path)
            n795 = Build Path(base path=w1245, name or relative path="data\\sys.ini" ("名称或相对路径")) -> (appended path=w1243:path)
            n796 = call <vilib>:"Open Config Data.vi"("configuration file path"=w1243) -> ("error out"=w1239:errorcluster, "refnum"=w1242:T5)  [unwired: 8 in, 1 out]
            n797 = vi-ref "斯坦道CODMn.lvlib:CODMn断电保存全局变量.vi"() -> (w1241:refnum<vi>)
            n798 = call <userlib>:"Write Panel to INI__ogtk.vi"("error in (no error)"=w1239, "VI ref"=w1241, "refnum"=w1242) -> ("error out"=w1238:errorcluster, "refnum out"=w1240:T5)  [unwired: 7 in]
            n799 = call <vilib>:"Close Config Data.vi"("error in (no error)"=w1238, "refnum"=w1240) -> ("error out"=w1233:errorcluster, "file path"=w1232:path)  [unwired: 8 in]
            n800 = Open/Create/Replace File(file path (use dialog)=w1232, error in=w1233) -> (refnum out=w1236:refnum<file>, error out=w1237:errorcluster)  [unwired: 4 in, 1 out]
            n801 = Flush File(refnum=w1236, error in=w1237) -> (refnum out=w1235:refnum<file>, error out=w1234:errorcluster)
            n802 = Close File(refnum=w1235, error in=w1234) -> ()  [unwired: 2 out]
          }
        }
      }
      event "CODMn跨度量程选择": Value Change {
        n803 = event-data() -> ()  [unwired: 1 in, 6 out]
        n804 = flat-sequence {
          frame #0 {
            n805 = global write "CODMn断电保存全局变量.vi" "CODMn跨度量程选择"("CODMn跨度量程选择") -> ()
          }
          frame #1 {
            n806 = call <vilib>:"Application Directory.vi"() -> ("Application Directory"=w1260:path)
            n807 = Build Path(base path=w1260, name or relative path="data\\sys.ini" ("名称或相对路径")) -> (appended path=w1258:path)
            n808 = call <vilib>:"Open Config Data.vi"("configuration file path"=w1258) -> ("error out"=w1254:errorcluster, "refnum"=w1257:T5)  [unwired: 8 in, 1 out]
            n809 = vi-ref "斯坦道CODMn.lvlib:CODMn断电保存全局变量.vi"() -> (w1256:refnum<vi>)
            n810 = call <userlib>:"Write Panel to INI__ogtk.vi"("error in (no error)"=w1254, "VI ref"=w1256, "refnum"=w1257) -> ("error out"=w1253:errorcluster, "refnum out"=w1255:T5)  [unwired: 7 in]
            n811 = call <vilib>:"Close Config Data.vi"("error in (no error)"=w1253, "refnum"=w1255) -> ("error out"=w1248:errorcluster, "file path"=w1247:path)  [unwired: 8 in]
            n812 = Open/Create/Replace File(file path (use dialog)=w1247, error in=w1248) -> (refnum out=w1251:refnum<file>, error out=w1252:errorcluster)  [unwired: 4 in, 1 out]
            n813 = Flush File(refnum=w1251, error in=w1252) -> (refnum out=w1250:refnum<file>, error out=w1249:errorcluster)
            n814 = Close File(refnum=w1250, error in=w1249) -> ()  [unwired: 2 out]
          }
        }
      }
      event "CODMn零点核查选择": Value Change {
        n815 = event-data() -> ()  [unwired: 1 in, 6 out]
        n816 = global write "CODMn断电保存全局变量.vi" "CODMn零点核查选择"("CODMn零点核查选择") -> ()
      }
      event "校准1", "校准2", "校准3", "校准4", "校准5": Value Change {
        n817 = event-data() -> ()  [unwired: 1 in, 6 out]
        n818 = flat-sequence {
          frame #0 {
            n819 = Build Array("校准1", "校准2", "校准3", "校准4", "校准5") -> (w1264:bool[])
            n820 = for {
              tunnel: w1264 -> [w1275] mode=indexing
              i -> [w1268]
              n821 = case shown="4" w1268 {
                tunnel: ["浓度1" "浓度2" "浓度3" "浓度4" "浓度5"] -> w1271
                frame 0, Default {
                }
                frame 1 {
                }
                frame 2 {
                }
                frame 3 {
                }
                frame 4 {
                }
              }
              n822 = Multiply(x=w1271, y=100.0) -> (x*y=w1269:dbl)
              n823 = Insert Into Array(array=u16[] [] ("values"), index=0 ("索引"), new element=w1269) -> (w1272:u16[])
              n824 = case shown="真" w1275 {
                tunnel: w1272 -> [_ w1282]
                tunnel: w1268 -> [_ w1285]
                frame False {
                }
                frame True {
                  n825 = Increment(x=w1285) -> (x+1=→"当前校准":i32)
                  n826 = call "CODMnMB_api.vi"("STEP"=enum16{"open", "read", "write", "close"}."write", "values"=w1282, "starting address"=u16 4274) -> ()  [unwired: 5 in, 4 out]
                }
              }
            }
          }
          frame #1 {
            n827 = local read "当前校准"() -> (w1292:i32)
            n828 = case shown="5" w1292 {
              tunnel: [w1296 w1297 w1298 w1299 w1300] -> w1291
              frame 1, Default {
                n829 = local read "浓度1"() -> (w1296:dbl)
              }
              frame 2 {
                n830 = local read "浓度2"() -> (w1297:dbl)
              }
              frame 3 {
                n831 = local read "浓度3"() -> (w1298:dbl)
              }
              frame 4 {
                n832 = local read "浓度4"() -> (w1299:dbl)
              }
              frame 5 {
                n833 = local read "浓度5"() -> (w1300:dbl)
              }
            }
            n834 = Not Equal To 0?(x=w1291) -> (x != 0?=w1289:bool)
            n835 = case shown="真" w1289 {
              tunnel: [u16 8 ("address") u16 9 ("address")] -> w1295
              tunnel: ["校零" ("测量模式") "校标" ("测量模式")] -> w1290
              frame False {
              }
              frame True {
              }
            }
            n836 = global write "COD测量模式全局.vi" "测量模式"(w1290) -> ()
            n837 = Insert Into Array(array=u16[] [] ("values"), index=0 ("索引"), new element=w1295) -> (w1286:u16[])
            n838 = call "CODMnMB_api.vi"("STEP"=enum16{"open", "read", "write", "close"}."write", "values"=w1286, "starting address"=u16 4608 ("address")) -> ()  [unwired: 5 in, 4 out]
          }
          frame #2 {
            n839 = call <vilib>:"Application Directory.vi"() -> ("Application Directory"=w1312:path)
            n840 = Build Path(base path=w1312, name or relative path="data\\Set.ini" ("名称或相对路径")) -> (appended path=w1314:path)
            n841 = local read "当前校准"() -> (w1307:i32)
            n842 = call <vilib>:"Open Config Data.vi"("configuration file path"=w1314) -> ("error out"=w1310:errorcluster, "refnum"=w1311:T5)  [unwired: 8 in, 1 out]
            n843 = call-poly <vilib>:"Write Key.vi"("section"="CODMn", "error in (no error)"=w1310, "value"=w1307, "key"="当前选用的校准" ("section"), "refnum"=w1311) -> ("error out"=w1305:errorcluster, "refnum out"=w1306:T5)  [unwired: 4 in, 1 out]
            n844 = call <vilib>:"Close Config Data.vi"("error in (no error)"=w1305, "refnum"=w1306) -> ()  [unwired: 8 in, 2 out]
          }
        }
      }
      event "自动切换量程:", "低切高阈值:", "高切低阈值:": Value Change {
        n845 = event-data() -> ()  [unwired: 1 in, 6 out]
        n846 = flat-sequence {
          frame #0 {
            n847 = local read "自动切换量程:"() -> (w1317:enum16{"关闭", "自动切换测一次", "自动切换测两次"})
            n848 = local read "低切高阈值:"() -> (w1316:dbl)
            n849 = local read "高切低阈值:"() -> (w1315:dbl)
            n850 = global write "CODMn断电保存全局变量.vi" "自动切换量程:"(w1317) -> ()
            n851 = global write "CODMn断电保存全局变量.vi" "低切高阈值:"(w1316) -> ()
            n852 = global write "CODMn断电保存全局变量.vi" "高切低阈值:"(w1315) -> ()
          }
          frame #1 {
            n853 = call <vilib>:"Application Directory.vi"() -> ("Application Directory"=w1331:path)
            n854 = Build Path(base path=w1331, name or relative path="data\\sys.ini" ("名称或相对路径")) -> (appended path=w1329:path)
            n855 = call <vilib>:"Open Config Data.vi"("configuration file path"=w1329) -> ("error out"=w1325:errorcluster, "refnum"=w1328:T5)  [unwired: 8 in, 1 out]
            n856 = vi-ref "斯坦道CODMn.lvlib:CODMn断电保存全局变量.vi"() -> (w1327:refnum<vi>)
            n857 = call <userlib>:"Write Panel to INI__ogtk.vi"("error in (no error)"=w1325, "VI ref"=w1327, "refnum"=w1328) -> ("error out"=w1324:errorcluster, "refnum out"=w1326:T5)  [unwired: 7 in]
            n858 = call <vilib>:"Close Config Data.vi"("error in (no error)"=w1324, "refnum"=w1326) -> ("error out"=w1319:errorcluster, "file path"=w1318:path)  [unwired: 8 in]
            n859 = Open/Create/Replace File(file path (use dialog)=w1318, error in=w1319) -> (refnum out=w1322:refnum<file>, error out=w1323:errorcluster)  [unwired: 4 in, 1 out]
            n860 = Flush File(refnum=w1322, error in=w1323) -> (refnum out=w1321:refnum<file>, error out=w1320:errorcluster)
            n861 = Close File(refnum=w1321, error in=w1320) -> ()  [unwired: 2 out]
          }
        }
      }
      event "模型": Value Change {
        n862 = event-data() -> ()  [unwired: 1 in, 6 out]
        n863 = call <vilib>:"Application Directory.vi"() -> ("Application Directory"=w1341:path)
        n864 = Build Path(base path=w1341, name or relative path="data\\Set.ini" ("名称或相对路径")) -> (appended path=w1339:path)
        n865 = call <vilib>:"Open Config Data.vi"("configuration file path"=w1339) -> ("error out"=w1337:errorcluster, "refnum"=w1338:T5)  [unwired: 8 in, 1 out]
        n866 = local read "模型"() -> (w1332:enum32{"线性", "多项式"})
        n867 = call-poly <vilib>:"Write Key.vi"("section"="CODMn模型选择" ("key"), "error in (no error)"=w1337, "value"=w1332, "key"="线性和多项式", "refnum"=w1338) -> ("error out"=w1333:errorcluster, "refnum out"=w1334:T5)  [unwired: 4 in, 1 out]
        n868 = call <vilib>:"Close Config Data.vi"("error in (no error)"=w1333, "refnum"=w1334) -> ()  [unwired: 8 in, 2 out]
      }
      event "浓度1", "浓度2", "浓度3", "泵滴定数1", "泵滴定数2", "泵滴定数3", "启用1", "启用2", "启用3", "浓度4", "浓度5", "泵滴定数4", "泵滴定数5", "启用4", "启用5": Value Change {
        n869 = event-data() -> ()  [unwired: 1 in, 6 out]
        n870 = local read "选用水样"() -> (w1357:enum16{"葡萄糖", "草酸钠"})
        n871 = local read "量程选择"() -> (w1356:enum16{"低量程", "高量程", "0-2量程"})
        n872 = case shown="\"0-2量程\"" w1356 {
          tunnel: ["低量程" "高量程" "0-2量程"] -> w1354
          frame "低量程", Default {
          }
          frame "高量程" {
          }
          frame "0-2量程" {
          }
        }
        n873 = call <vilib>:"Application Directory.vi"() -> ("Application Directory"=w1416:path)
        n874 = case shown="\"葡萄糖\", 默认" w1357 {
          tunnel: ["葡萄糖标线" ("section") "草酸钠标线" ("section")] -> w1363
          frame "葡萄糖", Default {
          }
          frame "草酸钠" {
          }
        }
        n875 = Build Path(base path=w1416, name or relative path="data\\Set.ini" ("名称或相对路径")) -> (appended path=w1414:path)
        n876 = call <vilib>:"Open Config Data.vi"("configuration file path"=w1414) -> ("error out"=w1412:errorcluster, "refnum"=w1413:T5)  [unwired: 8 in, 1 out]
        n877 = local read "浓度1"() -> (w1410:dbl)
        n878 = Concatenate Strings(w1363, w1354) -> (w1355:string)
        n879 = local read "浓度2"() -> (w1394:dbl)
        n880 = call-poly <vilib>:"Write Key.vi"("section"=w1355, "error in (no error)"=w1412, "value"=w1410, "key"="浓度1", "refnum"=w1413) -> ("error out"=w1409:errorcluster, "refnum out"=w1408:T5)  [unwired: 4 in, 1 out]
        n881 = local read "浓度3"() -> (w1390:dbl)
        n882 = call-poly <vilib>:"Write Key.vi"("section"=w1355, "error in (no error)"=w1409, "value"=w1394, "key"="浓度2", "refnum"=w1408) -> ("error out"=w1407:errorcluster, "refnum out"=w1406:T5)  [unwired: 4 in, 1 out]
        n883 = local read "泵滴定数1"() -> (w1388:dbl)
        n884 = call-poly <vilib>:"Write Key.vi"("section"=w1355, "error in (no error)"=w1407, "value"=w1390, "key"="浓度3", "refnum"=w1406) -> ("error out"=w1405:errorcluster, "refnum out"=w1404:T5)  [unwired: 4 in, 1 out]
        n885 = call-poly <vilib>:"Write Key.vi"("section"=w1355, "error in (no error)"=w1405, "value"=w1388, "key"="泵滴定数1", "refnum"=w1404) -> ("error out"=w1403:errorcluster, "refnum out"=w1402:T5)  [unwired: 4 in, 1 out]
        n886 = local read "泵滴定数2"() -> (w1386:dbl)
        n887 = call-poly <vilib>:"Write Key.vi"("section"=w1355, "error in (no error)"=w1403, "value"=w1386, "key"="泵滴定数2", "refnum"=w1402) -> ("error out"=w1401:errorcluster, "refnum out"=w1400:T5)  [unwired: 4 in, 1 out]
        n888 = local read "泵滴定数3"() -> (w1384:dbl)
        n889 = local read "浓度4"() -> (w1353:dbl)
        n890 = call-poly <vilib>:"Write Key.vi"("section"=w1355, "error in (no error)"=w1401, "value"=w1384, "key"="泵滴定数3", "refnum"=w1400) -> ("error out"=w1399:errorcluster, "refnum out"=w1398:T5)  [unwired: 4 in, 1 out]
        n891 = local read "浓度5"() -> (w1352:dbl)
        n892 = call-poly <vilib>:"Write Key.vi"("section"=w1355, "error in (no error)"=w1399, "value"=w1353, "key"="浓度4", "refnum"=w1398) -> ("error out"=w1392:errorcluster, "refnum out"=w1393:T5)  [unwired: 4 in, 1 out]
        n893 = call-poly <vilib>:"Write Key.vi"("section"=w1355, "error in (no error)"=w1392, "value"=w1352, "key"="浓度5", "refnum"=w1393) -> ("error out"=w1350:errorcluster, "refnum out"=w1351:T5)  [unwired: 4 in, 1 out]
        n894 = local read "泵滴定数4"() -> (w1349:dbl)
        n895 = call-poly <vilib>:"Write Key.vi"("section"=w1355, "error in (no error)"=w1350, "value"=w1349, "key"="泵滴定数4", "refnum"=w1351) -> ("error out"=w1397:errorcluster, "refnum out"=w1396:T5)  [unwired: 4 in, 1 out]
        n896 = local read "泵滴定数5"() -> (w1348:dbl)
        n897 = call-poly <vilib>:"Write Key.vi"("section"=w1355, "error in (no error)"=w1397, "value"=w1348, "key"="泵滴定数5", "refnum"=w1396) -> ("error out"=w1346:errorcluster, "refnum out"=w1347:T5)  [unwired: 4 in, 1 out]
        n898 = local read "启用1"() -> (w1372:bool)
        n899 = call-poly <vilib>:"Write Key.vi"("section"=w1355, "error in (no error)"=w1346, "value"=w1372, "key"="启用1", "refnum"=w1347) -> ("error out"=w1368:errorcluster, "refnum out"=w1371:T5)  [unwired: 4 in, 1 out]
        n900 = local read "启用2"() -> (w1369:bool)
        n901 = call-poly <vilib>:"Write Key.vi"("section"=w1355, "error in (no error)"=w1368, "value"=w1369, "key"="启用2", "refnum"=w1371) -> ("error out"=w1379:errorcluster, "refnum out"=w1378:T5)  [unwired: 4 in, 1 out]
        n902 = local read "启用3"() -> (w1367:bool)
        n903 = call-poly <vilib>:"Write Key.vi"("section"=w1355, "error in (no error)"=w1379, "value"=w1367, "key"="启用3", "refnum"=w1378) -> ("error out"=w1377:errorcluster, "refnum out"=w1376:T5)  [unwired: 4 in, 1 out]
        n904 = local read "启用4"() -> (w1342:bool)
        n905 = call-poly <vilib>:"Write Key.vi"("section"=w1355, "error in (no error)"=w1377, "value"=w1342, "key"="启用4", "refnum"=w1376) -> ("error out"=w1375:errorcluster, "refnum out"=w1374:T5)  [unwired: 4 in, 1 out]
        n906 = local read "启用5"() -> (w1343:bool)
        n907 = call-poly <vilib>:"Write Key.vi"("section"=w1355, "error in (no error)"=w1375, "value"=w1343, "key"="启用5", "refnum"=w1374) -> ("error out"=w1344:errorcluster, "refnum out"=w1345:T5)  [unwired: 4 in, 1 out]
        n908 = local read "选用水样"() -> (w1362:enum16{"葡萄糖", "草酸钠"})
        n909 = call-poly <vilib>:"Write Key.vi"("section"="标线选择", "error in (no error)"=w1344, "value"=w1362, "key"="选用水样", "refnum"=w1345) -> ("error out"=w1359:errorcluster, "refnum out"=w1360:T5)  [unwired: 4 in, 1 out]
        n910 = call <vilib>:"Close Config Data.vi"("error in (no error)"=w1359, "refnum"=w1360) -> ()  [unwired: 8 in, 2 out]
      }
      event "读取": Value Change {
        (unwired) u16 94 ("number of holding registers")
        (unwired) u16 4616 ("starting address")
        n911 = event-data() -> ()  [unwired: 1 in, 6 out]
        n912 = Bundle By Name(cluster=cluster{"命令":string} {"命令"=""} ("元素"), "命令"="CODMn读取公式" ("名称（未命名）")) -> (w1422:cluster{"命令":string})
        n913 = Enqueue Element(queue=w1426, element=w1422, error in (no error)=w1425) -> ()  [unwired: 1 in, 3 out]
      }
      event "写入": Mouse Down {
        n914 = event-data() -> ()  [unwired: 1 in, 8 out]
        n915 = local read "模型"() -> (w1430:enum32{"线性", "多项式"})
        n916 = case shown="\"多项式\"" w1430 {
          tunnel: [w1432 w1475] -> w1428
          tunnel: [w1431 w1474] -> w1427
          frame "线性", Default {
            n917 = local read "测量模式(公式)"() -> (w1433:u16)
            n918 = case shown="7" w1433 {
              tunnel: [u16 4626 ("starting address") w1440 w1445 w1450 w1455 w1460 w1465 w1470] -> w1432
              frame 0, Default {
              }
              frame 1 {
                n919 = local read "量程选择"() -> (w1439:enum16{"低量程", "高量程", "0-2量程"})
                n920 = case shown="\"低量程\", 默认" w1439 {
                  tunnel: [u16 4626 ("starting address") u16 4632 ("starting address") u16 4638 ("starting address")] -> w1440
                  frame "低量程", Default {
                  }
                  frame "高量程" {
                  }
                  frame "0-2量程" {
                  }
                }
              }
              frame 2 {
                n921 = local read "量程选择"() -> (w1444:enum16{"低量程", "高量程", "0-2量程"})
                n922 = case shown="\"低量程\", 默认" w1444 {
                  tunnel: [u16 4638 ("starting address") u16 4644 ("starting address") u16 4638 ("starting address")] -> w1445
                  frame "低量程", Default {
                  }
                  frame "高量程" {
                  }
                  frame "0-2量程" {
                  }
                }
              }
              frame 3 {
                n923 = local read "量程选择"() -> (w1449:enum16{"低量程", "高量程", "0-2量程"})
                n924 = case shown="\"低量程\", 默认" w1449 {
                  tunnel: [u16 4650 ("starting address") u16 4656 ("starting address") u16 4638 ("starting address")] -> w1450
                  frame "低量程", Default {
                  }
                  frame "高量程" {
                  }
                  frame "0-2量程" {
                  }
                }
              }
              frame 4 {
                n925 = local read "量程选择"() -> (w1454:enum16{"低量程", "高量程", "0-2量程"})
                n926 = case shown="\"低量程\", 默认" w1454 {
                  tunnel: [u16 4662 ("starting address") u16 4668 ("starting address") u16 4638 ("starting address")] -> w1455
                  frame "低量程", Default {
                  }
                  frame "高量程" {
                  }
                  frame "0-2量程" {
                  }
                }
              }
              frame 5 {
                n927 = local read "量程选择"() -> (w1459:enum16{"低量程", "高量程", "0-2量程"})
                n928 = case shown="\"低量程\", 默认" w1459 {
                  tunnel: [u16 4674 ("starting address") u16 4680 ("starting address") u16 4638 ("starting address")] -> w1460
                  frame "低量程", Default {
                  }
                  frame "高量程" {
                  }
                  frame "0-2量程" {
                  }
                }
              }
              frame 6 {
                n929 = local read "量程选择"() -> (w1464:enum16{"低量程", "高量程", "0-2量程"})
                n930 = case shown="\"低量程\", 默认" w1464 {
                  tunnel: [u16 4686 ("starting address") u16 4692 ("starting address") u16 4638 ("starting address")] -> w1465
                  frame "低量程", Default {
                  }
                  frame "高量程" {
                  }
                  frame "0-2量程" {
                  }
                }
              }
              frame 7 {
                n931 = local read "量程选择"() -> (w1469:enum16{"低量程", "高量程", "0-2量程"})
                n932 = case shown="\"低量程\", 默认" w1469 {
                  tunnel: [u16 4698 ("starting address") u16 4704 ("starting address") u16 4638 ("starting address")] -> w1470
                  frame "低量程", Default {
                  }
                  frame "高量程" {
                  }
                  frame "0-2量程" {
                  }
                }
              }
            }
            n933 = local read "K"() -> (w1437:dbl)
            n934 = local read "b"() -> (w1436:dbl)
            n935 = Build Array(w1437, w1436, 0.0 ("元素")) -> (w1435:dbl[])
            n936 = call "浮点转CDAB整形cod.vi"("浮点数"=w1435) -> ("CDAB整形输出"=w1431:u16[])  [unwired: 10 in]
          }
          frame "多项式" {
            # "b,k,c"
            n937 = local read "测量模式(公式)"() -> (w1476:u16)
            n938 = case shown="1" w1476 {
              tunnel: [u16 4626 ("starting address") w1484 w1489 w1494 w1499 w1504 w1509 w1514] -> w1475
              frame 0, Default {
              }
              frame 1 {
                n939 = local read "量程选择"() -> (w1483:enum16{"低量程", "高量程", "0-2量程"})
                n940 = case shown="\"低量程\", 默认" w1483 {
                  tunnel: [u16 4626 ("starting address") u16 4632 ("starting address") u16 4638 ("starting address")] -> w1484
                  frame "低量程", Default {
                  }
                  frame "高量程" {
                  }
                  frame "0-2量程" {
                  }
                }
              }
              frame 2 {
                n941 = local read "量程选择"() -> (w1488:enum16{"低量程", "高量程", "0-2量程"})
                n942 = case shown="\"低量程\", 默认" w1488 {
                  tunnel: [u16 4638 ("starting address") u16 4644 ("starting address") u16 4638 ("starting address")] -> w1489
                  frame "低量程", Default {
                  }
                  frame "高量程" {
                  }
                  frame "0-2量程" {
                  }
                }
              }
              frame 3 {
                n943 = local read "量程选择"() -> (w1493:enum16{"低量程", "高量程", "0-2量程"})
                n944 = case shown="\"低量程\", 默认" w1493 {
                  tunnel: [u16 4650 ("starting address") u16 4656 ("starting address") u16 4638 ("starting address")] -> w1494
                  frame "低量程", Default {
                  }
                  frame "高量程" {
                  }
                  frame "0-2量程" {
                  }
                }
              }
              frame 4 {
                n945 = local read "量程选择"() -> (w1498:enum16{"低量程", "高量程", "0-2量程"})
                n946 = case shown="\"低量程\", 默认" w1498 {
                  tunnel: [u16 4662 ("starting address") u16 4668 ("starting address") u16 4638 ("starting address")] -> w1499
                  frame "低量程", Default {
                  }
                  frame "高量程" {
                  }
                  frame "0-2量程" {
                  }
                }
              }
              frame 5 {
                n947 = local read "量程选择"() -> (w1503:enum16{"低量程", "高量程", "0-2量程"})
                n948 = case shown="\"低量程\", 默认" w1503 {
                  tunnel: [u16 4674 ("starting address") u16 4680 ("starting address") u16 4638 ("starting address")] -> w1504
                  frame "低量程", Default {
                  }
                  frame "高量程" {
                  }
                  frame "0-2量程" {
                  }
                }
              }
              frame 6 {
                n949 = local read "量程选择"() -> (w1508:enum16{"低量程", "高量程", "0-2量程"})
                n950 = case shown="\"低量程\", 默认" w1508 {
                  tunnel: [u16 4686 ("starting address") u16 4692 ("starting address") u16 4638 ("starting address")] -> w1509
                  frame "低量程", Default {
                  }
                  frame "高量程" {
                  }
                  frame "0-2量程" {
                  }
                }
              }
              frame 7 {
                n951 = local read "量程选择"() -> (w1513:enum16{"低量程", "高量程", "0-2量程"})
                n952 = case shown="\"低量程\", 默认" w1513 {
                  tunnel: [u16 4698 ("starting address") u16 4704 ("starting address") u16 4638 ("starting address")] -> w1514
                  frame "低量程", Default {
                  }
                  frame "高量程" {
                  }
                  frame "0-2量程" {
                  }
                }
              }
            }
            n953 = local read "多项式系数1"() -> (w1481:dbl[])
            n954 = Index Array(array=w1481) -> (element #1=w1478:dbl, element #2=w1479:dbl, element #3=w1477:dbl)  [unwired: 3 in]
            n955 = Build Array(w1479, w1478, w1477) -> (w1480:dbl[])
            n956 = call "浮点转CDAB整形cod.vi"("浮点数"=w1480) -> ("CDAB整形输出"=w1474:u16[])  [unwired: 10 in]
          }
        }
        n957 = call "CODMnMB_api.vi"("STEP"=enum16{"open", "read", "write", "close"}."write", "values"=w1427, "starting address"=w1428) -> ()  [unwired: 5 in, 4 out]
      }
      event "一键写入": Value Change {
        n958 = event-data() -> ()  [unwired: 1 in, 6 out]
        n959 = local read "模型"() -> (w1518:enum32{"线性", "多项式"})
        n960 = case shown="\"多项式\"" w1518 {
          frame "线性", Default {
            n961 = property on="测量模式(公式)" class="Ring (严格)"() -> ("NumItems"=w1519:u32)  [unwired: 2 in, 2 out]
            n962 = for {
              N: w1519 -> [_]
              i -> [w1524]
              n963 = Increment(x=w1524) -> (x+1=w1523:i32)
              n964 = local read "K"() -> (w1528:dbl)
              n965 = case shown="1" w1523 {
                tunnel: [u16 4626 ("starting address") w1534 w1539 w1544 w1549 w1554 w1559 w1564] -> w1521
                frame 0, Default {
                }
                frame 1 {
                  n966 = local read "量程选择"() -> (w1533:enum16{"低量程", "高量程", "0-2量程"})
                  n967 = case shown="\"低量程\", 默认" w1533 {
                    tunnel: [u16 4626 ("starting address") u16 4632 ("starting address") u16 4638 ("starting address")] -> w1534
                    frame "低量程", Default {
                    }
                    frame "高量程" {
                    }
                    frame "0-2量程" {
                    }
                  }
                }
                frame 2 {
                  n968 = local read "量程选择"() -> (w1538:enum16{"低量程", "高量程", "0-2量程"})
                  n969 = case shown="\"低量程\", 默认" w1538 {
                    tunnel: [u16 4638 ("starting address") u16 4644 ("starting address") u16 4638 ("starting address")] -> w1539
                    frame "低量程", Default {
                    }
                    frame "高量程" {
                    }
                    frame "0-2量程" {
                    }
                  }
                }
                frame 3 {
                  n970 = local read "量程选择"() -> (w1543:enum16{"低量程", "高量程", "0-2量程"})
                  n971 = case shown="\"低量程\", 默认" w1543 {
                    tunnel: [u16 4650 ("starting address") u16 4656 ("starting address") u16 4638 ("starting address")] -> w1544
                    frame "低量程", Default {
                    }
                    frame "高量程" {
                    }
                    frame "0-2量程" {
                    }
                  }
                }
                frame 4 {
                  n972 = local read "量程选择"() -> (w1548:enum16{"低量程", "高量程", "0-2量程"})
                  n973 = case shown="\"高量程\"" w1548 {
                    tunnel: [u16 4662 ("starting address") u16 4668 ("starting address") u16 4638 ("starting address")] -> w1549
                    frame "低量程", Default {
                    }
                    frame "高量程" {
                    }
                    frame "0-2量程" {
                    }
                  }
                }
                frame 5 {
                  n974 = local read "量程选择"() -> (w1553:enum16{"低量程", "高量程", "0-2量程"})
                  n975 = case shown="\"低量程\", 默认" w1553 {
                    tunnel: [u16 4674 ("starting address") u16 4680 ("starting address") u16 4638 ("starting address")] -> w1554
                    frame "低量程", Default {
                    }
                    frame "高量程" {
                    }
                    frame "0-2量程" {
                    }
                  }
                }
                frame 6 {
                  n976 = local read "量程选择"() -> (w1558:enum16{"低量程", "高量程", "0-2量程"})
                  n977 = case shown="\"低量程\", 默认" w1558 {
                    tunnel: [u16 4686 ("starting address") u16 4692 ("starting address") u16 4638 ("starting address")] -> w1559
                    frame "低量程", Default {
                    }
                    frame "高量程" {
                    }
                    frame "0-2量程" {
                    }
                  }
                }
                frame 7 {
                  n978 = local read "量程选择"() -> (w1563:enum16{"低量程", "高量程", "0-2量程"})
                  n979 = case shown="\"低量程\", 默认" w1563 {
                    tunnel: [u16 4698 ("starting address") u16 4704 ("starting address") u16 4638 ("starting address")] -> w1564
                    frame "低量程", Default {
                    }
                    frame "高量程" {
                    }
                    frame "0-2量程" {
                    }
                  }
                }
              }
              n980 = local read "b"() -> (w1529:dbl)
              n981 = Build Array(w1528, w1529, 0.0 ("元素")) -> (w1530:dbl[])
              n982 = call "浮点转CDAB整形cod.vi"("浮点数"=w1530) -> ("CDAB整形输出"=w1527:u16[])  [unwired: 10 in]
              n983 = Insert Into Array(array=u16[] [], index=0 ("索引"), new element=w1527) -> (w1520:u16[])
              n984 = call "CODMnMB_api.vi"("STEP"=enum16{"open", "read", "write", "close"}."write", "values"=w1520, "starting address"=w1521) -> ()  [unwired: 5 in, 4 out]
            }
          }
          frame "多项式" {
            # "b,k,c"
            n985 = property on="测量模式(公式)" class="Ring (严格)"() -> ("NumItems"=w1568:u32)  [unwired: 2 in, 2 out]
            n986 = for {
              N: w1568 -> [_]
              i -> [w1573]
              n987 = local read "多项式系数1"() -> (w1577:dbl[])
              n988 = Increment(x=w1573) -> (x+1=w1572:i32)
              n989 = case shown="2" w1572 {
                tunnel: [u16 4626 ("starting address") w1584 w1589 w1594 w1599 w1604 w1609 w1614] -> w1569
                frame 0, Default {
                }
                frame 1 {
                  n990 = local read "量程选择"() -> (w1583:enum16{"低量程", "高量程", "0-2量程"})
                  n991 = case shown="\"低量程\", 默认" w1583 {
                    tunnel: [u16 4626 ("starting address") u16 4632 ("starting address") u16 4638 ("starting address")] -> w1584
                    frame "低量程", Default {
                    }
                    frame "高量程" {
                    }
                    frame "0-2量程" {
                    }
                  }
                }
                frame 2 {
                  n992 = local read "量程选择"() -> (w1588:enum16{"低量程", "高量程", "0-2量程"})
                  n993 = case shown="\"低量程\", 默认" w1588 {
                    tunnel: [u16 4638 ("starting address") u16 4644 ("starting address") u16 4638 ("starting address")] -> w1589
                    frame "低量程", Default {
                    }
                    frame "高量程" {
                    }
                    frame "0-2量程" {
                    }
                  }
                }
                frame 3 {
                  n994 = local read "量程选择"() -> (w1593:enum16{"低量程", "高量程", "0-2量程"})
                  n995 = case shown="\"低量程\", 默认" w1593 {
                    tunnel: [u16 4650 ("starting address") u16 4656 ("starting address") u16 4638 ("starting address")] -> w1594
                    frame "低量程", Default {
                    }
                    frame "高量程" {
                    }
                    frame "0-2量程" {
                    }
                  }
                }
                frame 4 {
                  n996 = local read "量程选择"() -> (w1598:enum16{"低量程", "高量程", "0-2量程"})
                  n997 = case shown="\"低量程\", 默认" w1598 {
                    tunnel: [u16 4662 ("starting address") u16 4668 ("starting address") u16 4638 ("starting address")] -> w1599
                    frame "低量程", Default {
                    }
                    frame "高量程" {
                    }
                    frame "0-2量程" {
                    }
                  }
                }
                frame 5 {
                  n998 = local read "量程选择"() -> (w1603:enum16{"低量程", "高量程", "0-2量程"})
                  n999 = case shown="\"低量程\", 默认" w1603 {
                    tunnel: [u16 4674 ("starting address") u16 4680 ("starting address") u16 4638 ("starting address")] -> w1604
                    frame "低量程", Default {
                    }
                    frame "高量程" {
                    }
                    frame "0-2量程" {
                    }
                  }
                }
                frame 6 {
                  n1000 = local read "量程选择"() -> (w1608:enum16{"低量程", "高量程", "0-2量程"})
                  n1001 = case shown="\"低量程\", 默认" w1608 {
                    tunnel: [u16 4686 ("starting address") u16 4692 ("starting address") u16 4638 ("starting address")] -> w1609
                    frame "低量程", Default {
                    }
                    frame "高量程" {
                    }
                    frame "0-2量程" {
                    }
                  }
                }
                frame 7 {
                  n1002 = local read "量程选择"() -> (w1613:enum16{"低量程", "高量程", "0-2量程"})
                  n1003 = case shown="\"低量程\", 默认" w1613 {
                    tunnel: [u16 4698 ("starting address") u16 4704 ("starting address") u16 4638 ("starting address")] -> w1614
                    frame "低量程", Default {
                    }
                    frame "高量程" {
                    }
                    frame "0-2量程" {
                    }
                  }
                }
              }
              n1004 = Index Array(array=w1577) -> (element #1=w1580:dbl, element #2=w1579:dbl, element #3=w1581:dbl)  [unwired: 3 in]
              n1005 = Build Array(w1579, w1580, w1581) -> (w1578:dbl[])
              n1006 = call "浮点转CDAB整形cod.vi"("浮点数"=w1578) -> ("CDAB整形输出"=w1576:u16[])  [unwired: 10 in]
              n1007 = Insert Into Array(array=u16[] [], index=0 ("索引"), new element=w1576) -> (w1570:u16[])
              n1008 = call "CODMnMB_api.vi"("STEP"=enum16{"open", "read", "write", "close"}."write", "values"=w1570, "starting address"=w1569) -> ()  [unwired: 5 in, 4 out]
            }
          }
        }
      }
      event "滴定曲线": Value Change {
        n1009 = event-data() -> ()  [unwired: 1 in, 6 out]
        n1010 = property on="窗格" class="Pane"("Origin"=T13 {"Horizontal"=0, "Vertical"=3200} ("原点")) -> ()  [unwired: 2 in, 2 out]
      }
      event "历史波形": Value Change {
        n1011 = event-data() -> ()  [unwired: 1 in, 6 out]
        n1012 = call-poly <vilib>:"Read Waveforms from File.vi"() -> ("error out"=w1619:errorcluster, "first waveform in record"=w1620:waveform(dbl))  [unwired: 6 in, 2 out]
        n1013 = case shown="无错误" w1619 {
          tunnel: w1620 -> [w1623 _]
          frame No Error {
            n1014 = Unbundle By Name(w1623) -> ("t0"=→"波形时间":timestamp, "Y"=w1622:dbl[])  [unwired: 2 out]
            n1015 = local write "滴定数-ORP值"(w1622) -> ()
            n1016 = local write "ORP滴定曲线"(w1622) -> ()
          }
          frame Error {
            n1017 = One Button Dialog(message="打开失败" ("消息")) -> ()  [unwired: 1 in, 1 out]
          }
        }
      }
      event Timeout {
        n1018 = event-data() -> ()  [unwired: 1 in, 3 out]
      }
    }
  }
  n1019 = while {
    tunnel: w11 -> [w1630]
    tunnel: w10 -> [w1629]
    tunnel: w1 -> [_]
    stop <- FALSE stop-if-true
    (unwired) u16 50 ("number of holding registers")
    (unwired) u16 4224 ("starting address")
    n1020 = local read "自动切换量程:"() -> (w1638:enum16{"关闭", "自动切换测一次", "自动切换测两次"})
    n1021 = First Call?() -> (First Call?: T/F=w1625:bool)
    n1022 = case shown="真" w1625 {
      tunnel: w1630 -> [w1752 w1757]
      tunnel: w1629 -> [w1751 w1756]
      tunnel: [w1752 w1755] -> w1628
      tunnel: [w1751 w1754] -> w1627
      frame False {
      }
      frame True {
        n1023 = Bundle By Name(cluster=cluster{"命令":string} {"命令"=""} ("元素"), "命令"="CODMn读取参数" ("名称（未命名）")) -> (w1760:cluster{"命令":string})
        n1024 = Enqueue Element(queue=w1757, element=w1760, timeout in ms (-1)=1000 ("超时毫秒(-1)"), error in (no error)=w1756) -> (queue out=w1755:refnum<queue>, error out=w1754:errorcluster)  [unwired: 1 out]
      }
    }
    n1025 = case shown="\"自动切换测两次\"" w1638 {
      frame "关闭", Default {
      }
      frame "自动切换测一次" {
      }
      frame "自动切换测两次" {
        n1026 = local read "切换量程连续测两次"() -> (w1799:bool)
        n1027 = local read "待机"() -> (w1800:bool)
        n1028 = Compound Arithmetic op=AND ("复合运算")(w1800, w1799) -> (w1798:bool)
        n1029 = case shown="真" w1798 {
          frame False {
          }
          frame True {
            n1030 = local read "测量模式数字"() -> (w1805:i32)
            n1031 = case shown="0" w1805 {
              tunnel: [u16 4608 ("address") u16 4608 ("address") u16 4608 ("address") u16 4608 ("address") u16 4608 ("address") u16 4608 ("address") u16 4608 ("address") u16 4608 ("address") u16 4608 ("address") u16 4608 ("address")] -> w1801
              tunnel: [u16 1 ("address") u16 2 ("address") u16 3 ("address") u16 4 ("address") u16 5 ("address") u16 7 ("address") u16 6 ("address") u16 8 ("address") u16 9 ("address") u16 0 ("address")] -> w1808
              frame 0 {
              }
              frame 1 {
              }
              frame 2 {
              }
              frame 3 {
              }
              frame 4 {
              }
              frame 5 {
              }
              frame 6 {
              }
              frame 7 {
              }
              frame 8 {
              }
              frame 9, Default {
              }
            }
            n1032 = local write "切换量程连续测两次"(FALSE ("切换量程连续测两次")) -> ()
            n1033 = Insert Into Array(array=u16[] [] ("values"), index=0 ("索引"), new element=w1808) -> (w1802:u16[])
            n1034 = call "CODMnMB_api.vi"("STEP"=enum16{"open", "read", "write", "close"}."write", "values"=w1802, "starting address"=w1801) -> ()  [unwired: 5 in, 4 out]
          }
        }
      }
    }
    n1035 = Wait (ms)(milliseconds to wait=u32 500 ("等待时间（毫秒）")) -> ()  [unwired: 1 out]
    n1036 = Bundle By Name(cluster=cluster{"命令":string} {"命令"=""} ("元素"), "命令"="CODMn读取" ("名称（未命名）")) -> (w1632:cluster{"命令":string})
    n1037 = Enqueue Element(queue=w1628, element=w1632, timeout in ms (-1)=1000 ("超时毫秒(-1)"), error in (no error)=w1627) -> ()  [unwired: 3 out]
    n1038 = global read "COD读取DATA全局.vi" "测量状态"() -> (w1631:u16[])
    n1039 = To Word Integer(number=w1631) -> (16bit integer=w1667:i16[])
    n1040 = Index Array(array=w1667, index #1=0 ("索引"), index #4=3 ("索引"), index #14=13 ("索引"), index #15=14 ("索引"), index #21=20 ("索引"), index #32=31 ("索引")) -> (element #1=w1689:i16, element #2=w1688:i16, element #3=w1687:i16, element #4=w1635:i16, element #5=→"模式（受控）":i16, element #6=→"进样管":i16, element #7=→"高锰酸钾":i16, element #8=→"草酸钠":i16, element #9=→"硫酸":i16, element #10=w1666:i16, element #11=w1728:i16, element #12=w1648:i16, element #13=w1637:i16, element #14=w1745:i16, element #15=w1703:i16, element #16=w1636:i16, element #21=w1639:i16, element #33=→"分":i16, element #34=→"秒":i16)  [unwired: 28 in, 15 out]
    "多列列表框" <- w1636
    "CODMn工作状态" <- w1635
    n1041 = Number To Decimal String(number=w1639) -> (decimal integer string=→"基本量程(显示)":string)  [unwired: 1 in]
    n1042 = global write "COD浓度全局变量.vi" "基本量程"(w1639) -> ()
    n1043 = flat-sequence {
      frame #0 {
        # "A，B，K"
        n1044 = global read "COD读取DATA全局.vi" "ORP、时间"() -> (w1773:u16[])
        n1045 = To Word Integer(number=w1773) -> (16bit integer=w1796:i16[])
        n1046 = Split 1D Array(array=w1796, index=3 ("索引")) -> (first subarray=w1776:i16[], second subarray=w1795:i16[])
        n1047 = Index Array(array=w1776) -> (element #1=w1780:i16, element #2=w1779:i16, element #3=w1778:i16)  [unwired: 3 in]
        n1048 = Index Array(array=w1795) -> (element #1=w1790:i16, element #2=w1794:i16, element #3=w1793:i16, element #4=w1792:i16)  [unwired: 4 in]
        n1049 = To Single Precision Float(number=w1793) -> (single precision float=w1783:sgl)
        n1050 = To Single Precision Float(number=w1790) -> (single precision float=w1789:sgl)
        n1051 = To Single Precision Float(number=w1794) -> (single precision float=w1787:sgl)
        n1052 = To Single Precision Float(number=w1792) -> (single precision float=w1782:sgl)
        n1053 = Build Array(w1780, w1779, w1778) -> (w1777:i16[])
        n1054 = Divide(x=w1789, y=sgl 100.0) -> (x/y=w1788:sgl)
        n1055 = Number To Decimal String(number=w1787) -> (decimal integer string=→"ORP-A":string)  [unwired: 1 in]
        n1056 = Number To Decimal String(number=w1783) -> (decimal integer string=→"ORP-B":string)  [unwired: 1 in]
        n1057 = Number To Decimal String(number=w1782) -> (decimal integer string=→"ORP-K":string)  [unwired: 1 in]
        n1058 = local write "COD浓度（mg/L)"(w1788) -> ()
        n1059 = call "HexToDate.vi"("数组"=w1777) -> ("DATE"=w1781:timestamp[])  [unwired: 10 in]
        n1060 = Index Array(array=w1781) -> (element=w1774:timestamp)  [unwired: 1 in]
        n1061 = Format Date/Time String(seconds (now)=w1774) -> (date/time string=w1775:string)  [unwired: 2 in]
        n1062 = local write "数据时间"(w1775) -> ()
      }
    }
    n1063 = To Single Precision Float(number=w1666) -> (single precision float=→"ORP显示":sgl)
    n1064 = Divide(x=w1728, y=u16 10) -> (x/y=→"温度":dbl)
    n1065 = Equal?(x=w1648, y=u16 2) -> (x = y?=→"断电排液标记":bool)
    n1066 = Build Array(w1689, w1688, w1687) -> (w1690:i16[])
    n1067 = Equal?(x=w1648, y=u16 1) -> (x = y?=→"排液标记":bool)
    n1068 = Divide(x=w1703, y=u16 1000) -> (x/y=→"标度滴定值":dbl)
    n1069 = Divide(x=w1745, y=u16 1000) -> (x/y=→"零点滴定值":dbl)
    n1070 = Equal?(x=w1635, y=u16 0) -> (x = y?=→"待机":bool)
    n1071 = Equal?(x=w1635, y=u16 8) -> (x = y?=→"校零标记":bool)
    n1072 = Equal?(x=w1635, y=u16 9) -> (x = y?=→"校标标记":bool)
    n1073 = Equal?(x=w1635, y=u16 1) -> (x = y?=→"水样测量":bool)
    n1074 = Equal?(x=w1635, y=u16 7) -> (x = y?=→"质控样测量":bool)
    n1075 = Equal?(x=w1635, y=u16 10) -> (x = y?=→"加标回收测量":bool)
    n1076 = global write "COD测量模式全局.vi" "CODMn工作状态"(w1635) -> ()
    n1077 = Equal?(x=w1635, y=u16 2) -> (x = y?=→"标样核查标记":bool)
    n1078 = global write "运行时序全局变量.vi" "多列列表框"(w1636) -> ()
    n1079 = Equal?(x=w1635, y=u16 6) -> (x = y?=→"平行样测量":bool)
    n1080 = Equal?(x=w1635, y=u16 3) -> (x = y?=→"零点核查标记":bool)
    n1081 = Equal?(x=w1635, y=u16 4) -> (x = y?=→"跨度核查标记":bool)
    n1082 = Equal?(x=w1635, y=u16 5) -> (x = y?=→"空白测试标记":bool)
    n1083 = local read "断电排液标记"() -> (w1646:bool)
    n1084 = call "HexToDate.vi"("数组"=w1690) -> ("DATE"=w1685:timestamp[])  [unwired: 10 in]
    n1085 = Index Array(array=w1685) -> (element=→"仪器时间":timestamp)  [unwired: 1 in]
    n1086 = Get Date/Time In Seconds() -> (seconds since 1Jan1904=w1684:timestamp)
    "系统时间" <- w1684
    n1087 = call <vilib>:"Boolean Crossing PtByPt.vi"("direction"=enum16{"either", "false-true", "true-false"}."false-true", "input"=w1646) -> ("crossing"=w1645:bool)  [unwired: 1 in]
    n1088 = case shown="真" w1645 {
      frame False {
      }
      frame True {
        n1089 = Get Date/Time In Seconds() -> (seconds since 1Jan1904=w1837:timestamp)
        n1090 = Bundle(cluster=T15 {"时间标识"=timestamp(0 s since 1904-01-01), "参数"="", "日志信息"="", "流程参数"=""} ("data in"), "时间标识"=w1837, "参数"="CODMn" ("table输入"), "日志信息"="断电排液", "流程参数"="" ("table输入")) -> (w1835:T15)
        n1091 = call "流程日志字段定义.vi"("table输入"="操作日志", "data in"=w1835) -> ("table输出"=w1840:string, "columns"=w1841:string[], "data out"=w1842:T17)  [unwired: 7 in]
        n1092 = call "插入数据.vi"("data"=w1842, "columns"=w1841, "database"="database3.mdb", "table"=w1840) -> ()  [unwired: 7 in, 1 out]
      }
    }
    n1093 = Build Array(w1684) -> (w1683:timestamp[])
    n1094 = Equal?(x=w1637, y=u16 2) -> (x = y?=w1659:bool)
    "温控器故障" <- w1659
    n1095 = Equal?(x=w1637, y=u16 3) -> (x = y?=w1658:bool)
    "加热故障" <- w1658
    n1096 = Equal?(x=w1637, y=u16 4) -> (x = y?=w1657:bool)
    "高锰酸钾报警" <- w1657
    n1097 = Equal?(x=w1637, y=u16 5) -> (x = y?=w1656:bool)
    "草酸钠报警" <- w1656
    n1098 = Equal?(x=w1637, y=u16 6) -> (x = y?=w1655:bool)
    "测量错误" <- w1655
    n1099 = Equal?(x=w1637, y=u16 8) -> (x = y?=w1654:bool)
    "校零错误" <- w1654
    n1100 = Equal?(x=w1637, y=u16 7) -> (x = y?=w1653:bool)
    "校标错误" <- w1653
    n1101 = Equal?(x=w1637, y=u16 9) -> (x = y?=w1652:bool)
    "进水样超量程" <- w1652
    n1102 = Equal?(x=w1637, y=u16 10) -> (x = y?=w1651:bool)
    "排液故障" <- w1651
    n1103 = Equal?(x=w1637, y=u16 1) -> (x = y?=w1660:bool)
    "ORP故障" <- w1660
    n1104 = call "DateToHex.vi"("DATE"=w1683) -> ("数组"=w1682:u16[])  [unwired: 10 in]
    n1105 = call "DateToHex.vi"("DATE"=w1685) -> ("数组"=w1677:u16[])  [unwired: 10 in]
    n1106 = flat-sequence {
      frame #0 {
        n1107 = global read "COD读取DATA全局.vi" "M输出点"() -> (w1771:bool[])
        n1108 = global read "COD读取DATA全局.vi" "温度"() -> (w1772:bool[])
        n1109 = Index Array(array=w1772) -> (element=→"加热":bool)  [unwired: 1 in]
        n1110 = Index Array(array=w1771) -> (element #1=→"搅拌":bool, element #4=→"进水样":bool, element #5=→"进蒸馏水":bool, element #6=→"进标液":bool, element #7=→"进质控样":bool, element #8=→"进加标回收样":bool, element #9=→"进高锰酸钾":bool, element #10=→"进草酸钠":bool, element #11=→"进硫酸":bool)  [unwired: 11 in, 2 out]
      }
    }
    n1111 = Compound Arithmetic op=OR ("复合运算")(w1660, w1659, w1658, w1657, w1656, w1655, w1653, w1654, w1652, w1651) -> (→"故障标记":bool)
    n1112 = Index Array(array=w1677, index=2 ("索引")) -> (element=w1679:u16)
    n1113 = Bundle By Name(cluster=T4 {"ORP故障"=FALSE, "温控器故障"=FALSE, "加热故障"=FALSE, "高锰酸钾报警"=FALSE, "草酸钠报警"=FALSE, "测量错误"=FALSE, "校零错误"=FALSE, "校标错误"=FALSE, " 进水样超量程"=FALSE, "排液阀故障"=FALSE} ("报警簇"), "ORP故障"=w1660, "温控器故障"=w1659, "加热故障"=w1658, "高锰酸钾报警"=w1657, "草酸钠报警"=w1656, "测量错误"=w1655, "校零错误"=w1654, "校标错误"=w1653, "进水样超量程"=w1652, "排液阀故障"=w1651) -> (w1695:T4)
    "报警簇" <- w1695
    n1114 = Index Array(array=w1682, index=2 ("索引")) -> (element=w1680:u16)
    n1115 = Split Number(x=w1679) -> (hi(x)=w1673:u8)  [unwired: 1 out]
    n1116 = Split Number(x=w1680) -> (hi(x)=w1676:u8)  [unwired: 1 out]
    n1117 = To Byte Integer(number=w1673) -> (8bit integer=w1672:i8)
    n1118 = To Byte Integer(number=w1676) -> (8bit integer=w1675:i8)
    n1119 = call "CODMn报警信息.vi"("报警簇"=w1695) -> ("CODMN报警信息"=w1696:string)  [unwired: 10 in]
    n1120 = Subtract(x=w1672, y=w1675) -> (x-y=w1674:i8)
    n1121 = local read "通讯状态"() -> (w1643:bool)
    n1122 = feedback #3(w1696) -> (w1697:string)
    n1123 = feedback-in #3(w1696) -> ()
    n1124 = Not Equal?(x=w1696, y="") -> (x != y?=w1701:bool)
    n1125 = Absolute Value(x=w1674) -> (abs(x)=w1671:i8)
    n1126 = Greater Or Equal?(x=w1671, y=i8 60) -> (x >= y?=w1644:bool)
    n1127 = Not Equal?(x=w1696, y=w1697) -> (x != y?=w1698:bool)
    n1128 = And(x=w1644, y=w1643) -> (x .and. y?=w1642:bool)
    n1129 = case shown="真" w1642 {
      frame False {
      }
      frame True {
        # "相差60秒时间自动校准"
        n1130 = flat-sequence {
          frame #0 {
            n1131 = property on="时间校准" class="Bool (严格)"("Val(Sgnl)"=TRUE ("值(信号)")) -> ()  [unwired: 2 in, 2 out]
          }
          frame #1 {
            n1132 = Wait (ms)(milliseconds to wait=u32 500 ("等待时间（毫秒）")) -> ()  [unwired: 1 out]
          }
          frame #2 {
            n1133 = property on="时间校准" class="Bool (严格)"("Val(Sgnl)"=FALSE ("值(信号)")) -> ()  [unwired: 2 in, 2 out]
          }
        }
      }
    }
    n1134 = And(x=w1698, y=w1701) -> (x .and. y?=w1699:bool)
    n1135 = case shown="真" w1699 {
      tunnel: w1696 -> [_ w1843]
      frame False {
      }
      frame True {
        n1136 = Get Date/Time In Seconds() -> (seconds since 1Jan1904=w1845:timestamp)
        n1137 = Bundle By Name(cluster=T16 {"时间标识"=timestamp(0 s since 1904-01-01), "设备"="", "日志信息"=""} ("data in"), "时间标识"=w1845, "设备"="CODMn", "日志信息"=w1843) -> (w1846:T16)
        n1138 = call "报警信息字段定义.vi"("table输入"="报警信息", "data in"=w1846) -> ("table输出"=w1850:string, "columns"=w1851:string[], "data out"=w1852:T16)  [unwired: 7 in]
        n1139 = call "插入数据.vi"("data"=w1852, "columns"=w1851, "database"="database3.mdb", "table"=w1850) -> ()  [unwired: 7 in, 1 out]
      }
    }
  }
